vi "VIP_Phase_3.vi"() -> ()   [LabVIEW 2024]
uses:
  <vilib>/DAQmx/read.llb/DAQmx Read (Digital 1D Bool 1Chan 1Samp).vi
  <vilib>/Utility/file.llb/Write To Spreadsheet File (DBL).vi
  <vilib>/DAQmx/create/channels.llb/DAQmx Create Channel (DI-Digital Input).vi
  <vilib>/DAQmx/miscellaneous.llb/DAQmx Fill In Error Info.vi
  <vilib>/ptbypt/NI_PtbyPt.lvlib
panel:
  in  "LED 4":tag="Dev1/port0/line23"
  in  "LED 3":tag="Dev1/port0/line22"
  in  "LED 2":tag="Dev1/port0/line21"
  out "LED 4 (i)":dbl
  out "LED 3 (i)":dbl
  out "LED 2 (i)":dbl
  in  "LED 1":tag="Dev1/port0/line20"
  out "LED 1(i)":dbl
  out "4.2":bool
  out "mouse 4.2":cluster{"Y":dbl[], "Y":dbl[]}[](graph)
  out "mouse 4.1":cluster{"Y":dbl[], "Y":dbl[]}[](graph)
  in  "fake 4.2":bool
  in  "fake 4.1":bool
  out "ratio 4.2R":cluster{"Y":dbl[], "Y":dbl[]}[](graph)=[{"Y"=[2.5380001068115234, 12.063000202178955, 24.592000007629395, 36.145999908447266, 48.69600009918213, 58.23899984359741, 67.79099988937378, 81.40899991989136, 91.96199989318848, 99.9980001449585], "Y"=[0.0, 0.0, 0.0, 0.0, 0.0, 0.0, 0.0, 0.0, 0.0, 0.0]}]
  out "ratio 4.1L":cluster{"Y":dbl[], "Y":dbl[]}[](graph)=[{"Y"=[2.5380001068115234, 12.063000202178955, 24.592000007629395, 36.145999908447266, 48.69600009918213, 58.23899984359741, 67.79099988937378, 81.40899991989136, 91.96199989318848, 99.9980001449585], "Y"=[0.0, 0.0, 0.0, 0.0, 0.0, 0.0, 0.0, 0.0, 0.0, 0.0]}]
  out "ratio 4.2R":dbl
  out "ratio 4.1L":dbl
  in  "water dur (ms) 4.2":dbl=11.5
  in  "water port 4.2":tag="Dev1/port2/line0"
  out "Mouse path 4":path=path "C:/Users/Administrator/Documents/LabVIEW Data/a-lick-20140707-145848"
  out "Mouse file 4":string="a-lick-20140707-145848"
  in  "Mouse ID 4":string
  in  "water dur (ms) 4.1":dbl=9.0
  in  "water port 4.1":tag="Dev1/port1/line7"
  in  "free water 4.2":bool
  in  "free water 4.1":bool
  out "4.1":bool
  out "state 4.2":enum16{"waiting", "sound", "ITI"}(ring)=enum."ITI"
  out "state 4.1":enum16{"waiting", "sound", "ITI"}(ring)=enum."ITI"
  out "water # 4.1L":dbl
  out "water # 4.2R":dbl
  out "lick # 4.2R":dbl
  out "lick # 4.1L":dbl
  out "last water 4.2R":dbl
  out "last water 4.1L":dbl
  out "mistake # 4.2R":dbl
  out "mistake # 4.1L":dbl
  out "ratio 3.2R":cluster{"Y":dbl[], "Y":dbl[]}[](graph)=[{"Y"=[2.5380001068115234, 12.063000202178955, 24.592000007629395, 36.145999908447266, 48.69600009918213, 58.23899984359741, 67.79099988937378, 81.40899991989136, 91.96199989318848, 99.9980001449585], "Y"=[0.0, 0.0, 0.0, 0.0, 0.0, 0.0, 0.0, 0.0, 0.0, 0.0]}]
  out "ratio 3.1L":cluster{"Y":dbl[], "Y":dbl[]}[](graph)=[{"Y"=[2.5380001068115234, 12.063000202178955, 24.592000007629395, 36.145999908447266, 48.69600009918213, 58.23899984359741, 67.79099988937378, 81.40899991989136, 91.96199989318848, 99.9980001449585], "Y"=[0.0, 0.0, 0.0, 0.0, 0.0, 0.0, 0.0, 0.0, 0.0, 0.0]}]
  in  "free water 3.2":bool
  in  "free water 3.1":bool
  in  "water dur (ms) 3. 2":dbl=27.0
  in  "water dur (ms) 3.1":dbl=27.0
  out "mouse 3.2":cluster{"Y":dbl[], "Y":dbl[]}[](graph)
  out "mouse 3.1":cluster{"Y":dbl[], "Y":dbl[]}[](graph)
  in  "fake 3.2":bool
  in  "fake 3.1":bool
  out "last water 3.2R":dbl
  out "last water 3.1L":dbl
  out "mistake # 3.2R":dbl
  out "mistake # 3.1L":dbl
  out "water # 3.2R":dbl
  out "water # 3.1L":dbl
  out "lick # 3.2R":dbl
  out "lick # 3.1L":dbl
  out "ratio 3.2R":dbl
  out "ratio 3.1L":dbl
  in  "water port 3.2":tag="Dev1/port1/line6"
  out "3.2":bool
  out "state 3.2":enum16{"waiting", "sound", "ITI"}(ring)=enum."ITI"
  out "state 3.1":enum16{"waiting", "sound", "ITI"}(ring)=enum."ITI"
  out "3.1":bool
  out "Mouse path 3":path=path "C:/Users/Administrator/Documents/LabVIEW Data/a-lick-20140707-145848"
  out "Mouse file 3":string="a-lick-20140707-145848"
  in  "water port 3.1":tag="Dev1/port1/line5"
  in  "Mouse ID 3":string
  out "ratio 2.2R":cluster{"Y":dbl[], "Y":dbl[]}[](graph)=[{"Y"=[2.5380001068115234, 12.063000202178955, 24.592000007629395, 36.145999908447266, 48.69600009918213, 58.23899984359741, 67.79099988937378, 81.40899991989136, 91.96199989318848, 99.9980001449585], "Y"=[0.0, 0.0, 0.0, 0.0, 0.0, 0.0, 0.0, 0.0, 0.0, 0.0]}]
  out "ratio 2.1L":cluster{"Y":dbl[], "Y":dbl[]}[](graph)=[{"Y"=[2.5380001068115234, 12.063000202178955, 24.592000007629395, 36.145999908447266, 48.69600009918213, 58.23899984359741, 67.79099988937378, 81.40899991989136, 91.96199989318848, 99.9980001449585], "Y"=[0.0, 0.0, 0.0, 0.0, 0.0, 0.0, 0.0, 0.0, 0.0, 0.0]}]
  out "ratio 1.2R":cluster{"Y":dbl[], "Y":dbl[]}[](graph)=[{"Y"=[2.5380001068115234, 12.063000202178955, 24.592000007629395, 36.145999908447266, 48.69600009918213, 58.23899984359741, 67.79099988937378, 81.40899991989136, 91.96199989318848, 99.9980001449585], "Y"=[0.0, 0.0, 0.0, 0.0, 0.0, 0.0, 0.0, 0.0, 0.0, 0.0]}]
  out "mouse 2.2":cluster{"Y":dbl[], "Y":dbl[]}[](graph)
  out "mouse 2.1":cluster{"Y":dbl[], "Y":dbl[]}[](graph)
  in  "free water 2.2":bool
  in  "free water 2.1":bool
  out "last water 2.2R":dbl
  out "last water 2.1L":dbl
  out "mistake # 2.2R":dbl
  out "mistake # 2.1L":dbl
  out "water # 2.2R":dbl
  out "water # 2.1L":dbl
  out "lick  #  2.2R":dbl
  out "lick  #  2.1L":dbl
  out "2.1":bool
  out "ratio 2.2R":dbl
  out "ratio 2.1L":dbl
  out "2.2":bool
  in  "fake 2.2":bool
  in  "fake 2.1":bool
  out "Mouse path 2":path=path "C:/Users/Administrator/Documents/LabVIEW Data/a-lick-20140707-145848"
  out "Mouse file 2":string="a-lick-20140707-145848"
  in  "Mouse ID 2":string
  in  "water dur (ms) 2.2":dbl=27.5
  in  "water dur (ms) 2.1":dbl=36.5
  in  "water port 2.2":tag="Dev1/port1/line4"
  in  "water port 2.1":tag="Dev1/port1/line3"
  out "state 2.2":enum16{"waiting", "sound", "ITI"}(ring)=enum."ITI"
  out "state 2.1":enum16{"waiting", "sound", "ITI"}(ring)=enum."ITI"
  in  "sound port 2":tag="Dev1/ao1"
  out "time (s)":dbl=103.38100004196167
  out "mistake # 1.2R":dbl
  out "mistake # 1.1L":dbl
  in  "water dur (ms) 1.1":dbl=36.0
  in  "water port 1.1":tag="Dev1/port1/line1"
  in  "water dur (ms) 1.2":dbl=28.0
  in  "water port 1.2":tag="Dev1/port1/line2"
  out "1.1":bool
  out "1.2":bool
  out "state 1.2":enum16{"waiting", "sound", "ITI"}(ring)=enum."ITI"
  out "lick # 1.2R":dbl
  out "water # 1.2R":dbl
  in  "fake 1.2":bool
  in  "free water 1.2":bool
  out "mouse 1.2":cluster{"Y":dbl[], "Y":dbl[]}[](graph)
  out "ratio 1.2R":dbl
  out "last water 1.2R":dbl
  out "ratio 1.1L":dbl
  out "ratio 1.1L":cluster{"Y":dbl[], "Y":dbl[]}[](graph)=[{"Y"=[2.5380001068115234, 12.063000202178955, 24.592000007629395, 36.145999908447266, 48.69600009918213, 58.23899984359741, 67.79099988937378, 81.40899991989136, 91.96199989318848, 99.9980001449585], "Y"=[0.0, 0.0, 0.0, 0.0, 0.0, 0.0, 0.0, 0.0, 0.0, 0.0]}]
  in  "free water 1.1":bool
  out "Right Speaker":dbl=5.0
  out "Left Speaker":dbl=5.0
  in  "sound file 2":path=path "C:/Users/cvm-gritton-lab/Documents/Lab View Programs/Lab View Programs/LabVIEW VIs/Tones/New_Phase_2_Sounds/200k_target2.wav"
  in  "ITI max (ms)":dbl=7000.0
  in  "ITI min (ms)":dbl=5000.0
  in  "reaction dur (ms)":dbl=1750.0
  in  "sound dur (ms)":dbl=3000.0
  in  "sound file 1":path=path "C:/Users/cvm-gritton-lab/Documents/Lab View Programs/Lab View Programs/LabVIEW VIs/Tones/New_Phase_2_Sounds/200k_target1.wav"
  in  "sound port 1":tag="Dev1/ao0"
  out "trial state":T1(ring)=enum."ITI"
  out "trial #":dbl=10.0
  out "current sound":dbl=1.0
  out "next sound":dbl[](array[numeric])
  out "Mouse path 1":path=path "C:/Users/Administrator/Documents/LabVIEW Data/a-lick-20140707-145848"
  in  "fake 1.1":bool
  out "mouse 1.1":cluster{"Y":dbl[], "Y":dbl[]}[](graph)
  out "ITI (s)":dbl=6.5
  out "last water 1.1L":dbl
  out "state 1.1":enum16{"waiting", "sound", "ITI"}(ring)=enum."ITI"
  out "water # 1.1L":dbl
  out "lick # 1.1L":dbl
  out "Mouse file 1":string="a-lick-20140707-145848"
  out "data folder":path=path "C:/LabVIEW VIs/LabVIEW data"
  in  "Mouse ID 1":string="VIP_1"
  in  "lick port":tag="Dev1/port0/line0:7"
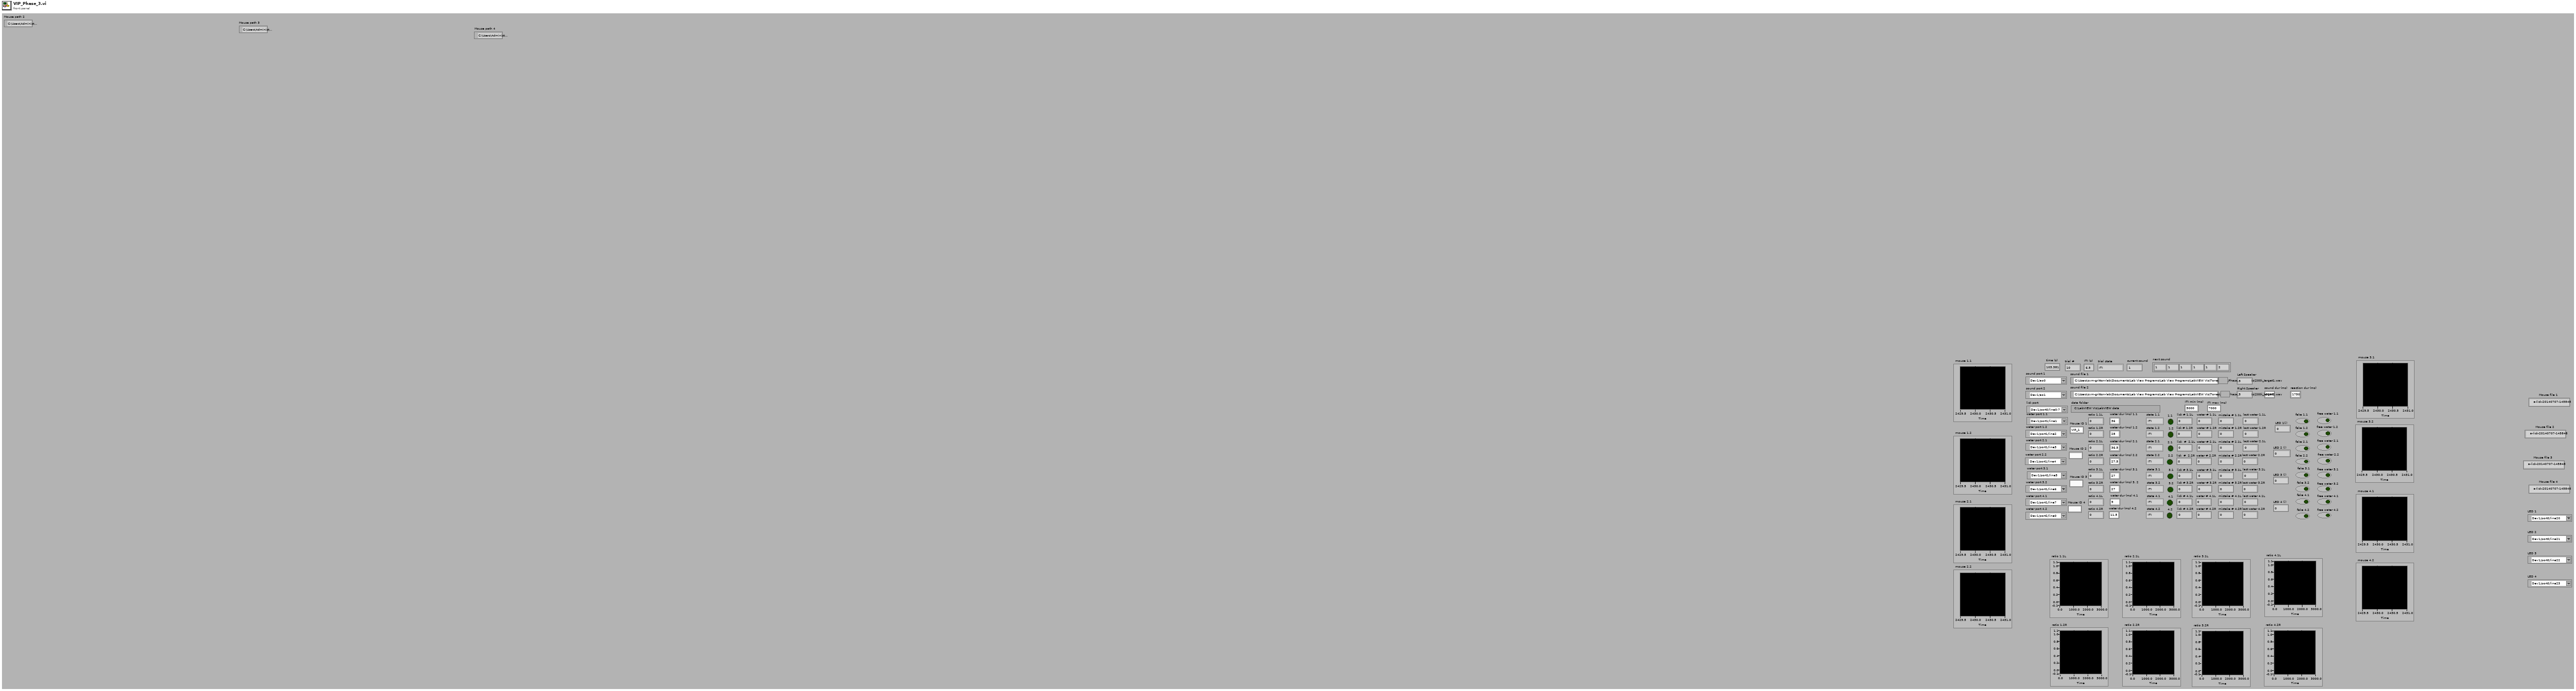
[diagram p1: front panel]
types:
  T1 = enum16{"prepare", "sound", "reaction window", "ITI", "free water", "graph", "data collection"}
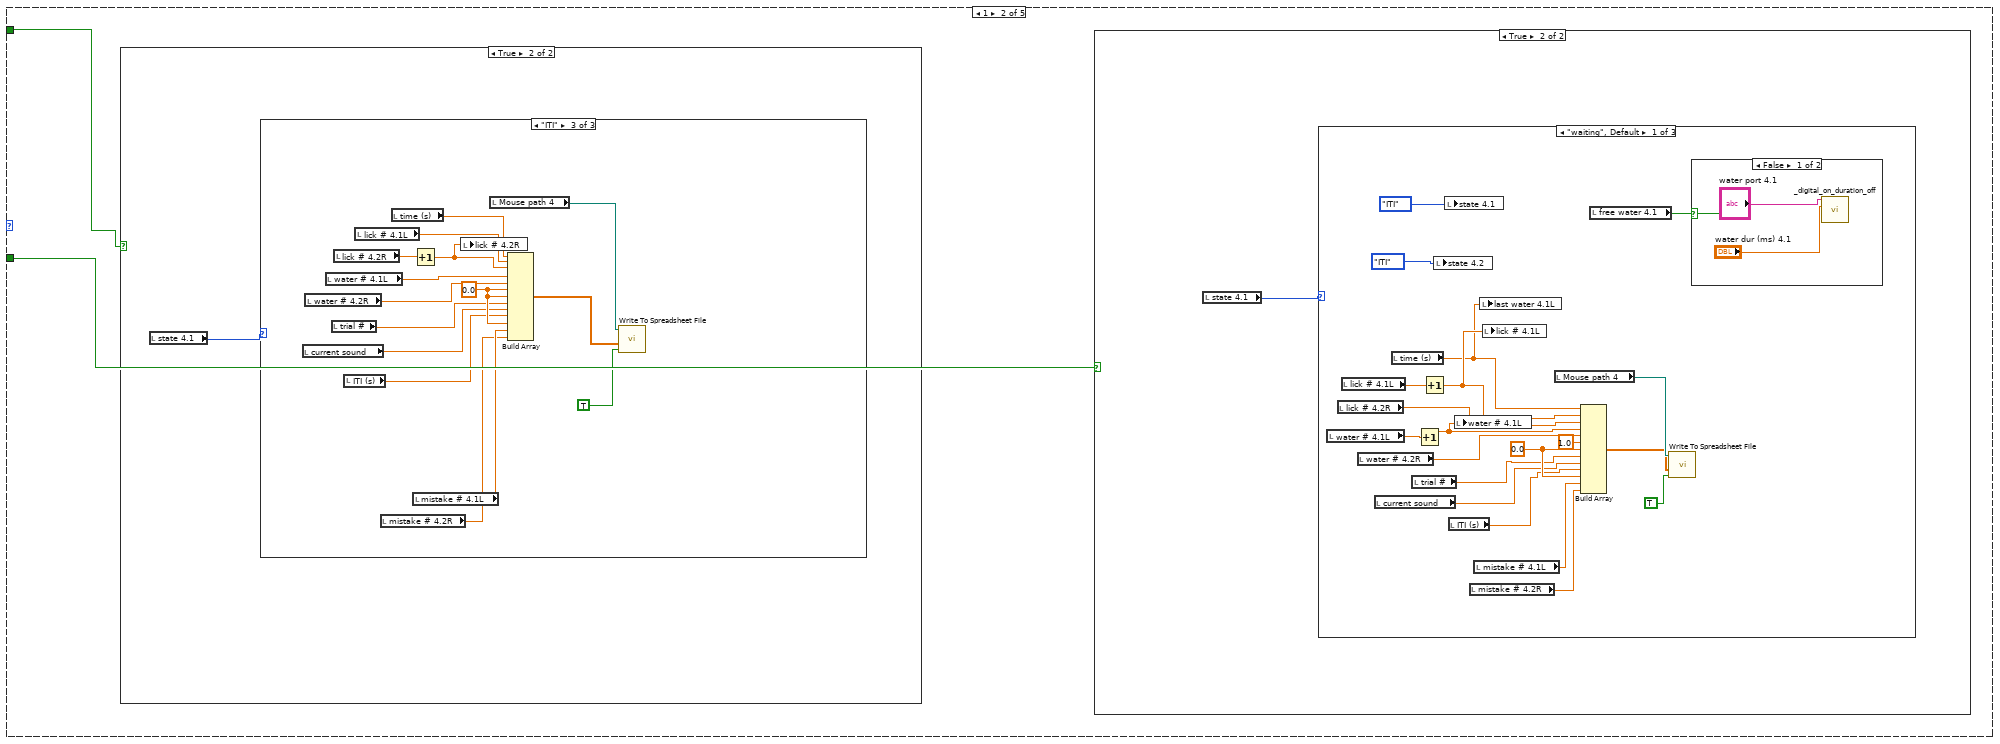
[diagram p3: hidden frame]
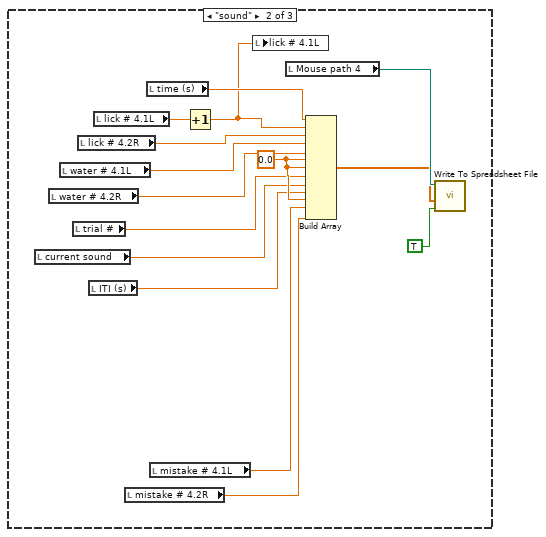
[diagram p6: hidden frame]
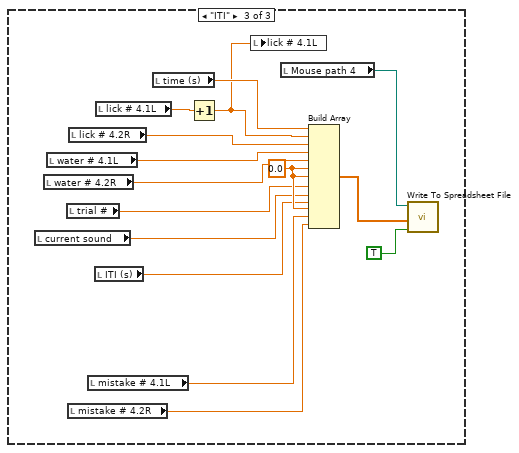
[diagram p7: hidden frame]
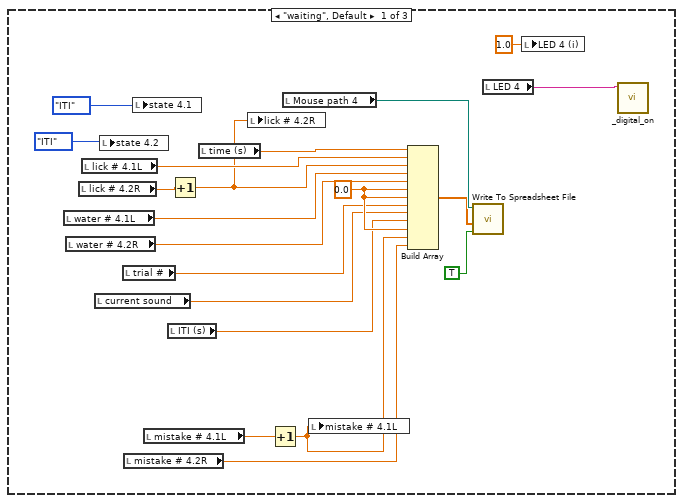
[diagram p9: hidden frame]
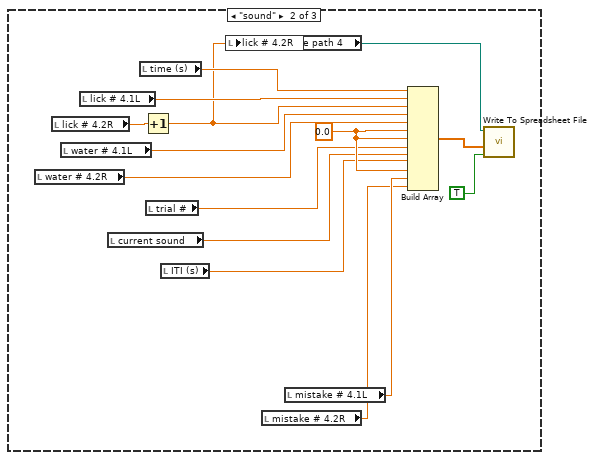
[diagram p10: hidden frame]
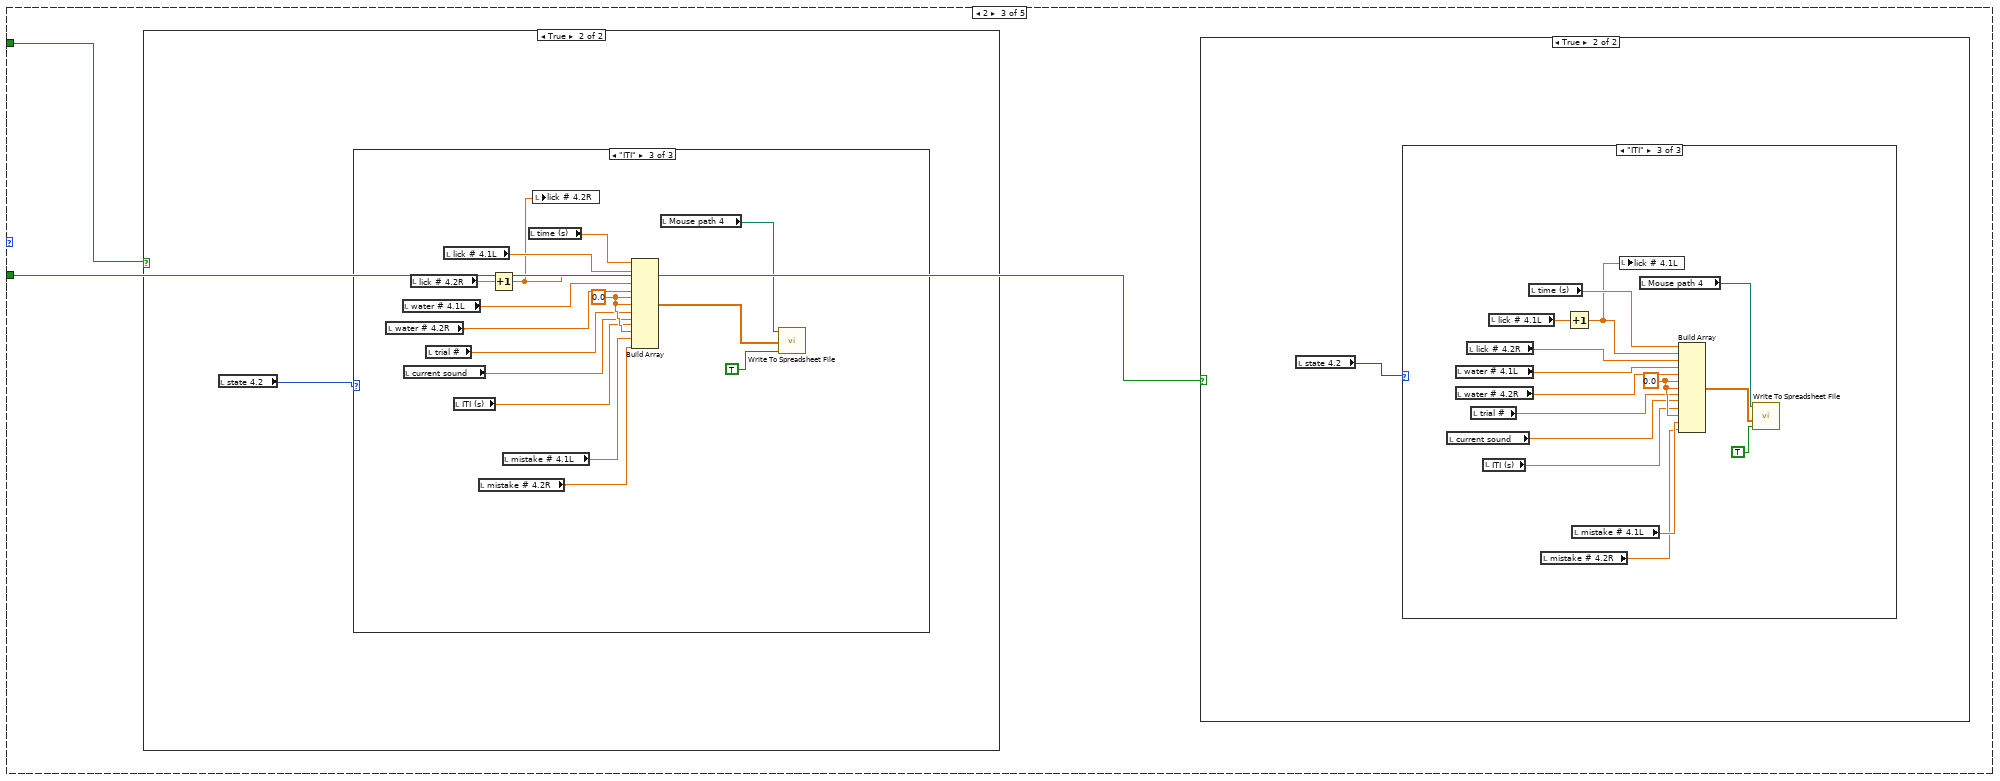
[diagram p11: hidden frame]
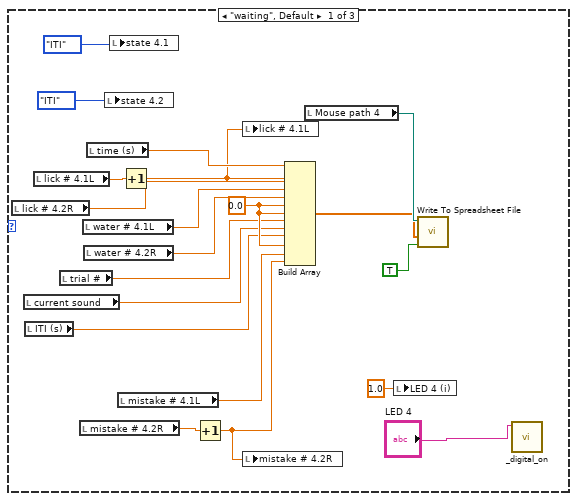
[diagram p13: hidden frame]
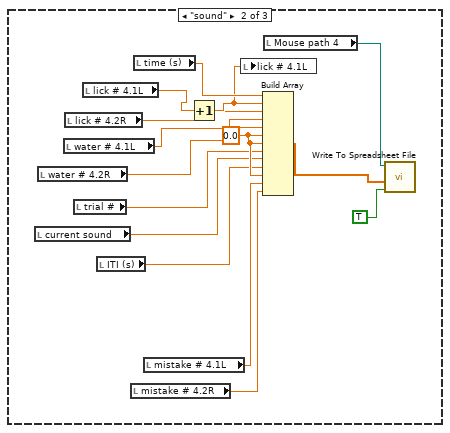
[diagram p14: hidden frame]
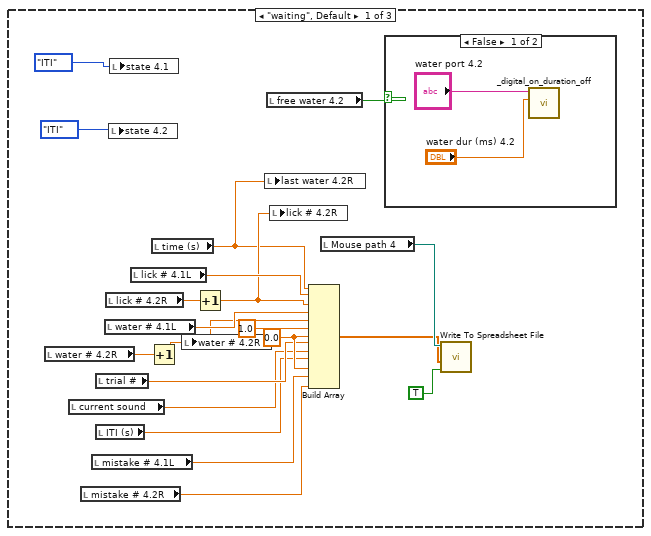
[diagram p16: hidden frame]
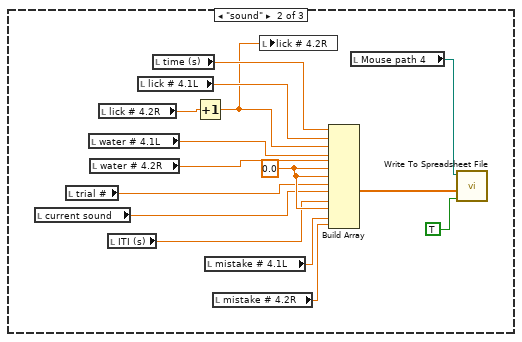
[diagram p18: hidden frame]
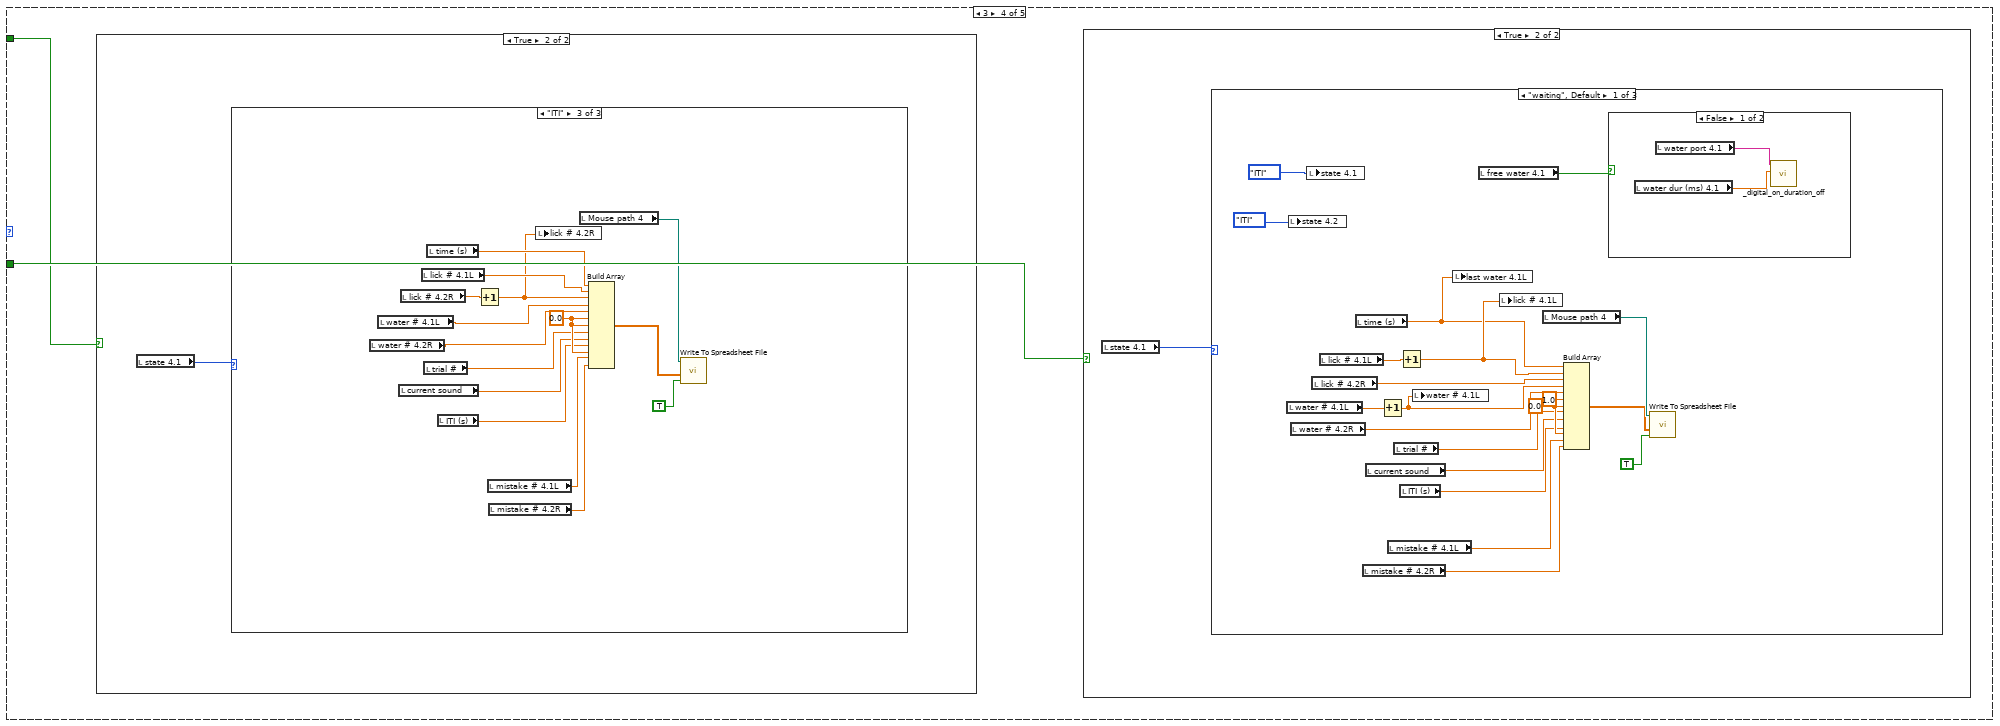
[diagram p19: hidden frame]
diagram:
  n1 = flat-sequence {
    frame #0 {
      w1 = 0.0 ("LED 1 (R)")
      w11 = 0.0 ("mistake # 1.1L")
      w3 = 0
      w21 = 0
      w10 = 0
      w2 = 0
      w9 = enum16{"waiting", "sound", "ITI"}."sound"
      n2 = Get Date/Time In Seconds() -> (seconds since 1Jan1904=w23:timestamp)
      n3 = call <vilib>:"Dflt Data Dir.vi"() -> ("App:Default Data Directory"=w5:path)
      "data folder" <- w5
      n4 = Format Date/Time String(time format string (%c)="%m%d%Y-%H%M%S-", seconds (now)=w23) -> (date/time string=w8:string)  [unwired: 1 in]
      n5 = Concatenate Strings(w8, "Mouse ID 1") -> (w26:string)
      "Mouse file 1" <- w26
      n6 = Concatenate Strings(w8, "Mouse ID 4") -> (w6:string)
      "Mouse file 4" <- w6
      n7 = Concatenate Strings(w8, "Mouse ID 2") -> (w16:string)
      "Mouse file 2" <- w16
      n8 = Concatenate Strings(w8, "Mouse ID 3") -> (w13:string)
      "Mouse file 3" <- w13
      n9 = Build Path(base path=w5, name or relative path=w26) -> (appended path=→"Mouse path 1":path)
      n10 = Build Path(base path=w5, name or relative path=w16) -> (appended path=→"Mouse path 2":path)
      n11 = Build Path(base path=w5, name or relative path=w13) -> (appended path=→"Mouse path 3":path)
      n12 = Build Path(base path=w5, name or relative path=w6) -> (appended path=→"Mouse path 4":path)
      n13 = call "_array_shuffle.vi"("total number"=70, "input array"=i32[] [1, 2, 3, 4, 1, 2, 3, 4]) -> ("output array"=→"next sound":dbl[])  [unwired: 9 in]
      n14 = local write "time (s)"(w21) -> ()
      "water # 1.1L" <- w2
      "lick # 1.1L" <- w2
      "state 1.1" <- w9
      "last water 1.1L" <- w10
      "current sound" <- w21
      "trial #" <- w21
      "ITI (s)" <- w21
      "Left Speaker" <- w21
      "Right Speaker" <- w21
      "ratio 1.1L" <- w3
      "last water 1.2R" <- w10
      "ratio 1.2R" <- w3
      "water # 1.2R" <- w2
      "lick # 1.2R" <- w2
      "state 1.2" <- w9
      "mistake # 1.1L" <- w11
      "mistake # 1.2R" <- w11
      "state 2.1" <- w9
      "state 2.2" <- w9
      "ratio 2.1L" <- w3
      "ratio 2.2R" <- w3
      "lick  #  2.1L" <- w2
      "lick  #  2.2R" <- w2
      "water # 2.1L" <- w2
      "water # 2.2R" <- w2
      "mistake # 2.1L" <- w11
      "mistake # 2.2R" <- w11
      "last water 2.1L" <- w10
      "last water 2.2R" <- w10
      "state 3.1" <- w9
      "state 3.2" <- w9
      "ratio 3.1L" <- w3
      "ratio 3.2R" <- w3
      "lick # 3.1L" <- w2
      "lick # 3.2R" <- w2
      "water # 3.1L" <- w2
      "water # 3.2R" <- w2
      "mistake # 3.1L" <- w11
      "mistake # 3.2R" <- w11
      "last water 3.1L" <- w10
      "last water 3.2R" <- w10
      "mistake # 4.1L" <- w11
      "mistake # 4.2R" <- w11
      "last water 4.1L" <- w10
      "last water 4.2R" <- w10
      "lick # 4.1L" <- w2
      "lick # 4.2R" <- w2
      "water # 4.2R" <- w2
      "water # 4.1L" <- w2
      "state 4.1" <- w9
      "state 4.2" <- w9
      "ratio 4.1L" <- w3
      "ratio 4.2R" <- w3
      "LED 1(i)" <- w1
      "LED 2 (i)" <- w1
      "LED 3 (i)" <- w1
      "LED 4 (i)" <- w1
    }
    frame #1 {
      # "file format:\n1. time stamp\n2. lick #\n3. water #\n4. water triggered by lick?\n5. trial start?\n6. trial #\n7. trial sound\n8. trial ITI\n9. free water?"
      n15 = call-poly <vilib>:"DAQmx Create Virtual Channel.vi"("lines"="lick port") -> ("task out"=w28:refnum<k21>)  [unwired: 13 in, 1 out]
      n16 = call <vilib>:"DAQmx Start Task.vi"("task/channels in"=w28) -> ("task out"=w29:refnum<k21>)  [unwired: 13 in, 1 out]
      n17 = while {
        tunnel: w29 -> [w88]
        tunnel: [w87] -> w30
        shift-right: [w78] -> _
        shift-left: _ -> [w86]
        shift-right: [w83] -> _
        shift-left: _ -> [w84]
        stop <- FALSE stop-if-true
        n18 = call-poly <vilib>:"DAQmx Read.vi"("task/channels in"=w88) -> ("task out"=w87:refnum<k21>, "data"=w79:bool[])  [unwired: 12 in, 1 out]
        n19 = Build Array("fake 1.1", "fake 1.2", "fake 2.1", "fake 2.2", "fake 3.1", "fake 3.2", "fake 4.1", "fake 4.2") -> (w75:bool[])
        n20 = Or(x=w79, y=w75) -> (x .or. y?=w78:bool[])
        n21 = Index Array(array=w78) -> (element #1=w81:bool, element #2=w67:bool, element #3=w58:bool, element #4=w55:bool, element #5=w47:bool, element #6=w44:bool, element #7=w39:bool, element #8=w35:bool)  [unwired: 8 in]
        n22 = call "Collector1."("Signals"=w58) -> ("Collected Signals"=w59:dynamicdata)  [unwired: 9 in, 1 out]
        n23 = call "Collector1.2"("Signals"=w67) -> ("Collected Signals"=w66:dynamicdata)  [unwired: 9 in, 1 out]
        n24 = call "Collector1.7"("Signals"=w35) -> ("Collected Signals"=w37:dynamicdata)  [unwired: 9 in, 1 out]
        n25 = call "Collector1.3"("Signals"=w55) -> ("Collected Signals"=w56:dynamicdata)  [unwired: 9 in, 1 out]
        n26 = call "Collector1.6"("Signals"=w39) -> ("Collected Signals"=w40:dynamicdata)  [unwired: 9 in, 1 out]
        n27 = call "Collector1.1"("Signals"=w81) -> ("Collected Signals"=w68:dynamicdata)  [unwired: 9 in, 1 out]
        n28 = call "Collector1.5"("Signals"=w44) -> ("Collected Signals"=w45:dynamicdata)  [unwired: 9 in, 1 out]
        n29 = call "Collector1.4"("Signals"=w47) -> ("Collected Signals"=w48:dynamicdata)  [unwired: 9 in, 1 out]
        n30 = local read "time (s)"() -> (w82:dbl)
        n31 = call "Collector"("Signals"=w82) -> ("Collected Signals"=w34:dynamicdata)  [unwired: 9 in, 1 out]
        n32 = call "Build XY Graph1.1"("Y Input"=w68, "X Input"=w34) -> ("XY Graph"=→"mouse 1.1":cluster{"Y":dbl[], "Y":dbl[]}[])  [unwired: 3 in, 6 out]
        n33 = call "Build XY Graph1."("Y Input"=w59, "X Input"=w34) -> ("XY Graph"=→"mouse 2.1":cluster{"Y":dbl[], "Y":dbl[]}[])  [unwired: 3 in, 6 out]
        n34 = call "Build XY Graph1.2"("Y Input"=w66, "X Input"=w34) -> ("XY Graph"=→"mouse 1.2":cluster{"Y":dbl[], "Y":dbl[]}[])  [unwired: 3 in, 6 out]
        n35 = call "Build XY Graph1.7"("Y Input"=w37, "X Input"=w34) -> ("XY Graph"=→"mouse 4.2":cluster{"Y":dbl[], "Y":dbl[]}[])  [unwired: 3 in, 6 out]
        n36 = call "Build XY Graph1.3"("Y Input"=w56, "X Input"=w34) -> ("XY Graph"=→"mouse 2.2":cluster{"Y":dbl[], "Y":dbl[]}[])  [unwired: 3 in, 6 out]
        n37 = call "Build XY Graph1.6"("Y Input"=w40, "X Input"=w34) -> ("XY Graph"=→"mouse 4.1":cluster{"Y":dbl[], "Y":dbl[]}[])  [unwired: 3 in, 6 out]
        n38 = call "Build XY Graph1.5"("Y Input"=w45, "X Input"=w34) -> ("XY Graph"=→"mouse 3.2":cluster{"Y":dbl[], "Y":dbl[]}[])  [unwired: 3 in, 6 out]
        n39 = call "Build XY Graph1.4"("Y Input"=w48, "X Input"=w34) -> ("XY Graph"=→"mouse 3.1":cluster{"Y":dbl[], "Y":dbl[]}[])  [unwired: 3 in, 6 out]
        n40 = Greater?(x=w78, y=w86) -> (0:w85:bool[])
        n41 = Index Array(array=w85) -> (element #1=w73:bool, element #2=w72:bool, element #3=w61:bool, element #4=w62:bool, element #5=w53:bool, element #6=w52:bool, element #7=w32:bool, element #8=w33:bool)  [unwired: 8 in]
        "1.2" <- w72
        "1.1" <- w73
        "2.2" <- w62
        "2.1" <- w61
        "3.1" <- w53
        "3.2" <- w52
        "4.1" <- w32
        "4.2" <- w33
        n42 = local read "current sound"() -> (w71:dbl)
        n43 = local read "current sound"() -> (w65:dbl)
        n44 = local read "current sound"() -> (w43:dbl)
        n45 = local read "current sound"() -> (w54:dbl)
        n46 = case shown="4" w54 {
          tunnel: w53 -> [_ w514 w620 w726 w832]
          tunnel: w52 -> [_ w513 w619 w725 w831]
          frame 0, Default {
          }
          frame 1 {
            n47 = case shown="True" w514 {
              frame False {
              }
              frame True {
                n48 = local read "state 3.1"() -> (w566:enum16{"waiting", "sound", "ITI"})
                n49 = case shown="\"waiting\", Default" w566 {
                  frame "waiting", Default {
                    w575 = 0.0 ("element")
                    n50 = local write "state 3.2"(enum16{"waiting", "sound", "ITI"}."ITI") -> ()
                    n51 = local read "free water 3.1"() -> (w586:bool)
                    n52 = local write "state 3.1"(enum16{"waiting", "sound", "ITI"}."ITI") -> ()
                    n53 = local read "water # 3.1L"() -> (w578:dbl)
                    n54 = local read "lick # 3.2R"() -> (w579:dbl)
                    n55 = local read "lick # 3.1L"() -> (w581:dbl)
                    n56 = local read "water # 3.2R"() -> (w576:dbl)
                    n57 = local read "current sound"() -> (w568:dbl)
                    n58 = case shown="False" w586 {
                      frame False {
                        n59 = call "_digital_on_duration_off.vi"("duration (ms)"="water dur (ms) 3.1", "digital port"="water port 3.1") -> ()  [unwired: 10 in]
                      }
                      frame True {
                      }
                    }
                    n60 = local read "mistake # 3.2R"() -> (w573:dbl)
                    n61 = local read "mistake # 3.1L"() -> (w574:dbl)
                    n62 = local read "ITI (s)"() -> (w567:dbl)
                    n63 = local read "trial #"() -> (w569:dbl)
                    n64 = Increment(x=w578) -> (x+1=w577:dbl)
                    n65 = Increment(x=w581) -> (x+1=w580:dbl)
                    n66 = local read "time (s)"() -> (w582:dbl)
                    n67 = local write "water # 3.1L"(w577) -> ()
                    n68 = local write "lick # 3.1L"(w580) -> ()
                    n69 = local write "last water 3.1L"(w582) -> ()
                    n70 = local read "Mouse path 3"() -> (w585:path)
                    n71 = Build Array(w582, w580, w579, w577, w576, 1.0 ("element"), w575, w569, w568, w567, w575, w574, w573) -> (w583:dbl[])
                    n72 = call-poly <vilib>:"Write To Spreadsheet File.vi"("append to file? (new file:F)"=TRUE, "1D data"=w583, "file path (dialog if empty)"=w585) -> ()  [unwired: 5 in, 1 out]
                  }
                  frame "sound" {
                    w594 = 0.0 ("element")
                    n73 = local read "current sound"() -> (w590:dbl)
                    n74 = local read "trial #"() -> (w591:dbl)
                    n75 = local read "water # 3.2R"() -> (w595:dbl)
                    n76 = local read "water # 3.1L"() -> (w596:dbl)
                    n77 = local read "mistake # 3.2R"() -> (w592:dbl)
                    n78 = local read "lick # 3.2R"() -> (w597:dbl)
                    n79 = local read "lick # 3.1L"() -> (w599:dbl)
                    n80 = local read "ITI (s)"() -> (w589:dbl)
                    n81 = local read "mistake # 3.1L"() -> (w593:dbl)
                    n82 = local read "time (s)"() -> (w600:dbl)
                    n83 = Increment(x=w599) -> (x+1=w598:dbl)
                    n84 = local write "lick # 3.1L"(w598) -> ()
                    n85 = local read "Mouse path 3"() -> (w603:path)
                    n86 = Build Array(w600, w598, w597, w596, w595, w594, w594, w591, w590, w589, w594, w593, w592) -> (w601:dbl[])
                    n87 = call-poly <vilib>:"Write To Spreadsheet File.vi"("append to file? (new file:F)"=TRUE, "1D data"=w601, "file path (dialog if empty)"=w603) -> ()  [unwired: 5 in, 1 out]
                  }
                  frame "ITI" {
                    w609 = 0.0 ("element")
                    n88 = local read "water # 3.2R"() -> (w610:dbl)
                    n89 = local read "current sound"() -> (w605:dbl)
                    n90 = local read "lick # 3.2R"() -> (w612:dbl)
                    n91 = local read "lick # 3.1L"() -> (w614:dbl)
                    n92 = local read "water # 3.1L"() -> (w611:dbl)
                    n93 = local read "trial #"() -> (w606:dbl)
                    n94 = local read "ITI (s)"() -> (w604:dbl)
                    n95 = local read "time (s)"() -> (w615:dbl)
                    n96 = Increment(x=w614) -> (x+1=w613:dbl)
                    n97 = local read "mistake # 3.1L"() -> (w608:dbl)
                    n98 = local read "mistake # 3.2R"() -> (w607:dbl)
                    n99 = local write "lick # 3.1L"(w613) -> ()
                    n100 = local read "Mouse path 3"() -> (w618:path)
                    n101 = Build Array(w615, w613, w612, w611, w610, w609, w609, w606, w605, w604, w609, w608, w607) -> (w616:dbl[])
                    n102 = call-poly <vilib>:"Write To Spreadsheet File.vi"("append to file? (new file:F)"=TRUE, "1D data"=w616, "file path (dialog if empty)"=w618) -> ()  [unwired: 5 in, 1 out]
                  }
                }
              }
            }
            n103 = case shown="True" w513 {
              frame False {
              }
              frame True {
                n104 = local read "state 3.1"() -> (w515:enum16{"waiting", "sound", "ITI"})
                n105 = case shown="\"ITI\"" w515 {
                  frame "waiting", Default {
                    w524 = 0.0 ("element")
                    n106 = local read "mistake # 3.1L"() -> (w523:dbl)
                    n107 = local write "state 3.2"(enum16{"waiting", "sound", "ITI"}."ITI") -> ()
                    n108 = local write "state 3.1"(enum16{"waiting", "sound", "ITI"}."ITI") -> ()
                    n109 = Increment(x=w523) -> (x+1=w522:dbl)
                    n110 = local read "water # 3.2R"() -> (w525:dbl)
                    n111 = local read "water # 3.1L"() -> (w526:dbl)
                    n112 = local read "lick # 3.2R"() -> (w528:dbl)
                    n113 = local read "current sound"() -> (w517:dbl)
                    n114 = local read "mistake # 3.2R"() -> (w521:dbl)
                    n115 = local write "mistake # 3.1L"(w522) -> ()
                    n116 = local read "lick # 3.1L"() -> (w529:dbl)
                    n117 = local read "ITI (s)"() -> (w516:dbl)
                    n118 = local read "trial #"() -> (w518:dbl)
                    n119 = local read "time (s)"() -> (w530:dbl)
                    n120 = Increment(x=w528) -> (x+1=w527:dbl)
                    n121 = local write "lick # 3.2R"(w527) -> ()
                    n122 = Build Array(w530, w529, w527, w526, w525, w524, w524, w518, w517, w516, w524, w522, w521) -> (w531:dbl[])
                    n123 = local read "Mouse path 3"() -> (w533:path)
                    n124 = call "_digital_on.vi"("digital port"="LED 3") -> ()  [unwired: 11 in]
                    n125 = call-poly <vilib>:"Write To Spreadsheet File.vi"("append to file? (new file:F)"=TRUE, "1D data"=w531, "file path (dialog if empty)"=w533) -> ()  [unwired: 5 in, 1 out]
                    n126 = local write "LED 3 (i)"(1.0 ("LED 3 (i)")) -> ()
                  }
                  frame "sound" {
                    w541 = 0.0 ("element")
                    n127 = local read "water # 3.1L"() -> (w543:dbl)
                    n128 = local read "lick # 3.2R"() -> (w545:dbl)
                    n129 = local read "water # 3.2R"() -> (w542:dbl)
                    n130 = local read "lick # 3.1L"() -> (w546:dbl)
                    n131 = local read "current sound"() -> (w537:dbl)
                    n132 = local read "trial #"() -> (w538:dbl)
                    n133 = local read "time (s)"() -> (w547:dbl)
                    n134 = Increment(x=w545) -> (x+1=w544:dbl)
                    n135 = local read "ITI (s)"() -> (w536:dbl)
                    n136 = local read "mistake # 3.2R"() -> (w539:dbl)
                    n137 = local read "mistake # 3.1L"() -> (w540:dbl)
                    n138 = local write "lick # 3.2R"(w544) -> ()
                    n139 = local read "Mouse path 3"() -> (w549:path)
                    n140 = Build Array(w547, w546, w544, w543, w542, w541, w541, w538, w537, w536, w541, w540, w539) -> (w548:dbl[])
                    n141 = call-poly <vilib>:"Write To Spreadsheet File.vi"("append to file? (new file:F)"=TRUE, "1D data"=w548, "file path (dialog if empty)"=w549) -> ()  [unwired: 5 in, 1 out]
                  }
                  frame "ITI" {
                    w556 = 0.0 ("element")
                    n142 = local read "water # 3.2R"() -> (w557:dbl)
                    n143 = local read "water # 3.1L"() -> (w558:dbl)
                    n144 = local read "lick # 3.2R"() -> (w560:dbl)
                    n145 = local read "current sound"() -> (w552:dbl)
                    n146 = local read "lick # 3.1L"() -> (w561:dbl)
                    n147 = local read "trial #"() -> (w553:dbl)
                    n148 = Increment(x=w560) -> (x+1=w559:dbl)
                    n149 = local read "time (s)"() -> (w562:dbl)
                    n150 = local read "mistake # 3.2R"() -> (w554:dbl)
                    n151 = local read "ITI (s)"() -> (w551:dbl)
                    n152 = local read "mistake # 3.1L"() -> (w555:dbl)
                    n153 = local write "lick # 3.2R"(w559) -> ()
                    n154 = local read "Mouse path 3"() -> (w564:path)
                    n155 = Build Array(w562, w561, w559, w558, w557, w556, w556, w553, w552, w551, w556, w555, w554) -> (w563:dbl[])
                    n156 = call-poly <vilib>:"Write To Spreadsheet File.vi"("append to file? (new file:F)"=TRUE, "1D data"=w563, "file path (dialog if empty)"=w564) -> ()  [unwired: 5 in, 1 out]
                  }
                }
              }
            }
          }
          frame 2 {
            n157 = case shown="True" w620 {
              frame False {
              }
              frame True {
                n158 = local read "state 3.2"() -> (w674:enum16{"waiting", "sound", "ITI"})
                n159 = case shown="\"waiting\", Default" w674 {
                  frame "waiting", Default {
                    w683 = 0.0 ("element")
                    n160 = local read "water # 3.2R"() -> (w684:dbl)
                    n161 = local read "water # 3.1L"() -> (w685:dbl)
                    n162 = local read "lick # 3.2R"() -> (w686:dbl)
                    n163 = local read "lick # 3.1L"() -> (w688:dbl)
                    n164 = local read "current sound"() -> (w676:dbl)
                    n165 = local write "state 3.2"(enum16{"waiting", "sound", "ITI"}."ITI") -> ()
                    n166 = local read "trial #"() -> (w677:dbl)
                    n167 = local read "ITI (s)"() -> (w675:dbl)
                    n168 = local read "mistake # 3.1L"() -> (w682:dbl)
                    n169 = local read "time (s)"() -> (w689:dbl)
                    n170 = local read "mistake # 3.2R"() -> (w681:dbl)
                    n171 = local write "state 3.1"(enum16{"waiting", "sound", "ITI"}."ITI") -> ()
                    n172 = Increment(x=w688) -> (x+1=w687:dbl)
                    n173 = local write "lick # 3.1L"(w687) -> ()
                    n174 = local read "Mouse path 3"() -> (w691:path)
                    n175 = Increment(x=w681) -> (x+1=w680:dbl)
                    n176 = local write "mistake # 3.2R"(w680) -> ()
                    n177 = Build Array(w689, w687, w686, w685, w684, w683, w683, w677, w676, w675, w683, w682, w680) -> (w690:dbl[])
                    n178 = local read "LED 3"() -> (w679:tag)
                    n179 = call-poly <vilib>:"Write To Spreadsheet File.vi"("append to file? (new file:F)"=TRUE, "1D data"=w690, "file path (dialog if empty)"=w691) -> ()  [unwired: 5 in, 1 out]
                    n180 = local write "LED 3 (i)"(1.0 ("LED 3 (i)")) -> ()
                    n181 = call "_digital_on.vi"("digital port"=w679) -> ()  [unwired: 11 in]
                  }
                  frame "sound" {
                    w700 = 0.0 ("element")
                    n182 = local read "current sound"() -> (w696:dbl)
                    n183 = local read "water # 3.2R"() -> (w701:dbl)
                    n184 = local read "water # 3.1L"() -> (w702:dbl)
                    n185 = local read "trial #"() -> (w697:dbl)
                    n186 = local read "lick # 3.2R"() -> (w703:dbl)
                    n187 = local read "lick # 3.1L"() -> (w705:dbl)
                    n188 = local read "ITI (s)"() -> (w695:dbl)
                    n189 = local read "mistake # 3.2R"() -> (w698:dbl)
                    n190 = local read "time (s)"() -> (w706:dbl)
                    n191 = local read "mistake # 3.1L"() -> (w699:dbl)
                    n192 = Increment(x=w705) -> (x+1=w704:dbl)
                    n193 = local write "lick # 3.1L"(w704) -> ()
                    n194 = local read "Mouse path 3"() -> (w708:path)
                    n195 = Build Array(w706, w704, w703, w702, w701, w700, w700, w697, w696, w695, w700, w699, w698) -> (w707:dbl[])
                    n196 = call-poly <vilib>:"Write To Spreadsheet File.vi"("append to file? (new file:F)"=TRUE, "1D data"=w707, "file path (dialog if empty)"=w708) -> ()  [unwired: 5 in, 1 out]
                  }
                  frame "ITI" {
                    w715 = 0.0 ("element")
                    n197 = local read "current sound"() -> (w711:dbl)
                    n198 = local read "water # 3.2R"() -> (w716:dbl)
                    n199 = local read "water # 3.1L"() -> (w717:dbl)
                    n200 = local read "lick # 3.2R"() -> (w718:dbl)
                    n201 = local read "trial #"() -> (w712:dbl)
                    n202 = local read "lick # 3.1L"() -> (w720:dbl)
                    n203 = local read "ITI (s)"() -> (w710:dbl)
                    n204 = local read "mistake # 3.2R"() -> (w713:dbl)
                    n205 = local read "time (s)"() -> (w721:dbl)
                    n206 = local read "mistake # 3.1L"() -> (w714:dbl)
                    n207 = Increment(x=w720) -> (x+1=w719:dbl)
                    n208 = local write "lick # 3.1L"(w719) -> ()
                    n209 = local read "Mouse path 3"() -> (w723:path)
                    n210 = Build Array(w721, w719, w718, w717, w716, w715, w715, w712, w711, w710, w715, w714, w713) -> (w722:dbl[])
                    n211 = call-poly <vilib>:"Write To Spreadsheet File.vi"("append to file? (new file:F)"=TRUE, "1D data"=w722, "file path (dialog if empty)"=w723) -> ()  [unwired: 5 in, 1 out]
                  }
                }
              }
            }
            n212 = case shown="True" w619 {
              frame False {
              }
              frame True {
                n213 = local read "state 3.2"() -> (w621:enum16{"waiting", "sound", "ITI"})
                n214 = case shown="\"ITI\"" w621 {
                  frame "waiting", Default {
                    w629 = 0.0 ("element")
                    n215 = local read "water # 3.2R"() -> (w631:dbl)
                    n216 = local read "current sound"() -> (w623:dbl)
                    n217 = local read "lick # 3.2R"() -> (w634:dbl)
                    n218 = local read "water # 3.1L"() -> (w632:dbl)
                    n219 = local read "trial #"() -> (w624:dbl)
                    n220 = local read "mistake # 3.2R"() -> (w627:dbl)
                    n221 = local write "state 3.1"(enum16{"waiting", "sound", "ITI"}."ITI") -> ()
                    n222 = local write "state 3.2"(enum16{"waiting", "sound", "ITI"}."ITI") -> ()
                    n223 = local read "ITI (s)"() -> (w622:dbl)
                    n224 = local read "lick # 3.1L"() -> (w635:dbl)
                    n225 = local read "mistake # 3.1L"() -> (w628:dbl)
                    n226 = local read "time (s)"() -> (w626:dbl)
                    n227 = Increment(x=w631) -> (x+1=w630:dbl)
                    n228 = Increment(x=w634) -> (x+1=w633:dbl)
                    n229 = local read "free water 3.2"() -> (w641:bool)
                    n230 = local write "water # 3.2R"(w630) -> ()
                    n231 = local write "last water 3.2R"(w626) -> ()
                    n232 = local write "lick # 3.2R"(w633) -> ()
                    n233 = local read "Mouse path 3"() -> (w637:path)
                    n234 = Build Array(w626, w635, w633, w632, w630, 1.0 ("element"), w629, w624, w623, w622, w629, w628, w627) -> (w636:dbl[])
                    n235 = case shown="False" w641 {
                      frame False {
                        n236 = call "_digital_on_duration_off.vi"("duration (ms)"="water dur (ms) 3. 2", "digital port"="water port 3.2") -> ()  [unwired: 10 in]
                      }
                      frame True {
                      }
                    }
                    n237 = call-poly <vilib>:"Write To Spreadsheet File.vi"("append to file? (new file:F)"=TRUE, "1D data"=w636, "file path (dialog if empty)"=w637) -> ()  [unwired: 5 in, 1 out]
                  }
                  frame "sound" {
                    w649 = 0.0 ("element")
                    n238 = local read "lick # 3.2R"() -> (w653:dbl)
                    n239 = local read "water # 3.1L"() -> (w651:dbl)
                    n240 = local read "current sound"() -> (w645:dbl)
                    n241 = local read "trial #"() -> (w646:dbl)
                    n242 = local read "water # 3.2R"() -> (w650:dbl)
                    n243 = local read "lick # 3.1L"() -> (w654:dbl)
                    n244 = local read "ITI (s)"() -> (w644:dbl)
                    n245 = local read "mistake # 3.2R"() -> (w647:dbl)
                    n246 = Increment(x=w653) -> (x+1=w652:dbl)
                    n247 = local read "mistake # 3.1L"() -> (w648:dbl)
                    n248 = local read "time (s)"() -> (w655:dbl)
                    n249 = local write "lick # 3.2R"(w652) -> ()
                    n250 = local read "Mouse path 3"() -> (w658:path)
                    n251 = Build Array(w655, w654, w652, w651, w650, w649, w649, w646, w645, w644, w649, w648, w647) -> (w656:dbl[])
                    n252 = call-poly <vilib>:"Write To Spreadsheet File.vi"("append to file? (new file:F)"=TRUE, "1D data"=w656, "file path (dialog if empty)"=w658) -> ()  [unwired: 5 in, 1 out]
                  }
                  frame "ITI" {
                    w664 = 0.0 ("element")
                    n253 = local read "water # 3.2R"() -> (w665:dbl)
                    n254 = local read "lick # 3.2R"() -> (w668:dbl)
                    n255 = local read "current sound"() -> (w660:dbl)
                    n256 = local read "water # 3.1L"() -> (w666:dbl)
                    n257 = local read "lick # 3.1L"() -> (w669:dbl)
                    n258 = local read "trial #"() -> (w661:dbl)
                    n259 = local read "ITI (s)"() -> (w659:dbl)
                    n260 = local read "time (s)"() -> (w670:dbl)
                    n261 = Increment(x=w668) -> (x+1=w667:dbl)
                    n262 = local read "mistake # 3.2R"() -> (w662:dbl)
                    n263 = local read "mistake # 3.1L"() -> (w663:dbl)
                    n264 = local write "lick # 3.2R"(w667) -> ()
                    n265 = local read "Mouse path 3"() -> (w672:path)
                    n266 = Build Array(w670, w669, w667, w666, w665, w664, w664, w661, w660, w659, w664, w663, w662) -> (w671:dbl[])
                    n267 = call-poly <vilib>:"Write To Spreadsheet File.vi"("append to file? (new file:F)"=TRUE, "1D data"=w671, "file path (dialog if empty)"=w672) -> ()  [unwired: 5 in, 1 out]
                  }
                }
              }
            }
          }
          frame 3 {
            n268 = case shown="True" w726 {
              frame False {
              }
              frame True {
                n269 = local read "state 3.1"() -> (w778:enum16{"waiting", "sound", "ITI"})
                n270 = case shown="\"ITI\"" w778 {
                  frame "waiting", Default {
                    w785 = 0.0 ("element")
                    n271 = local read "water # 3.2R"() -> (w787:dbl)
                    n272 = local read "water # 3.1L"() -> (w789:dbl)
                    n273 = local read "lick # 3.1L"() -> (w792:dbl)
                    n274 = local write "state 3.2"(enum16{"waiting", "sound", "ITI"}."ITI") -> ()
                    n275 = local read "lick # 3.2R"() -> (w790:dbl)
                    n276 = local write "state 3.1"(enum16{"waiting", "sound", "ITI"}."ITI") -> ()
                    n277 = local read "time (s)"() -> (w786:dbl)
                    n278 = local read "current sound"() -> (w781:dbl)
                    n279 = Increment(x=w792) -> (x+1=w791:dbl)
                    n280 = Increment(x=w789) -> (x+1=w788:dbl)
                    n281 = local read "trial #"() -> (w782:dbl)
                    n282 = local read "mistake # 3.2R"() -> (w783:dbl)
                    n283 = local read "free water 3.1"() -> (w796:bool)
                    n284 = local write "water # 3.1L"(w788) -> ()
                    n285 = local write "lick # 3.1L"(w791) -> ()
                    n286 = local write "last water 3.1L"(w786) -> ()
                    n287 = local read "ITI (s)"() -> (w780:dbl)
                    n288 = local read "mistake # 3.1L"() -> (w784:dbl)
                    n289 = local read "Mouse path 3"() -> (w795:path)
                    n290 = case shown="False" w796 {
                      frame False {
                        n291 = local read "water dur (ms) 3.1"() -> (w799:dbl)
                        n292 = local read "water port 3.1"() -> (w800:tag)
                        n293 = call "_digital_on_duration_off.vi"("duration (ms)"=w799, "digital port"=w800) -> ()  [unwired: 10 in]
                      }
                      frame True {
                      }
                    }
                    n294 = Build Array(w786, w791, w790, w788, w787, 1.0 ("element"), w785, w782, w781, w780, w785, w784, w783) -> (w793:dbl[])
                    n295 = call-poly <vilib>:"Write To Spreadsheet File.vi"("append to file? (new file:F)"=TRUE, "1D data"=w793, "file path (dialog if empty)"=w795) -> ()  [unwired: 5 in, 1 out]
                  }
                  frame "sound" {
                    w806 = 0.0 ("element")
                    n296 = local read "lick # 3.2R"() -> (w809:dbl)
                    n297 = local read "water # 3.2R"() -> (w807:dbl)
                    n298 = local read "water # 3.1L"() -> (w808:dbl)
                    n299 = local read "current sound"() -> (w802:dbl)
                    n300 = local read "lick # 3.1L"() -> (w811:dbl)
                    n301 = local read "trial #"() -> (w803:dbl)
                    n302 = local read "ITI (s)"() -> (w801:dbl)
                    n303 = Increment(x=w811) -> (x+1=w810:dbl)
                    n304 = local read "mistake # 3.2R"() -> (w804:dbl)
                    n305 = local read "time (s)"() -> (w812:dbl)
                    n306 = local read "mistake # 3.1L"() -> (w805:dbl)
                    n307 = local write "lick # 3.1L"(w810) -> ()
                    n308 = local read "Mouse path 3"() -> (w814:path)
                    n309 = Build Array(w812, w810, w809, w808, w807, w806, w806, w803, w802, w801, w806, w805, w804) -> (w813:dbl[])
                    n310 = call-poly <vilib>:"Write To Spreadsheet File.vi"("append to file? (new file:F)"=TRUE, "1D data"=w813, "file path (dialog if empty)"=w814) -> ()  [unwired: 5 in, 1 out]
                  }
                  frame "ITI" {
                    w821 = 0.0 ("element")
                    n311 = local read "water # 3.2R"() -> (w822:dbl)
                    n312 = local read "water # 3.1L"() -> (w823:dbl)
                    n313 = local read "lick # 3.2R"() -> (w824:dbl)
                    n314 = local read "lick # 3.1L"() -> (w826:dbl)
                    n315 = local read "current sound"() -> (w817:dbl)
                    n316 = local read "trial #"() -> (w818:dbl)
                    n317 = local read "ITI (s)"() -> (w816:dbl)
                    n318 = local read "time (s)"() -> (w827:dbl)
                    n319 = local read "mistake # 3.2R"() -> (w819:dbl)
                    n320 = local read "mistake # 3.1L"() -> (w820:dbl)
                    n321 = Increment(x=w826) -> (x+1=w825:dbl)
                    n322 = local write "lick # 3.1L"(w825) -> ()
                    n323 = local read "Mouse path 3"() -> (w829:path)
                    n324 = Build Array(w827, w825, w824, w823, w822, w821, w821, w818, w817, w816, w821, w820, w819) -> (w828:dbl[])
                    n325 = call-poly <vilib>:"Write To Spreadsheet File.vi"("append to file? (new file:F)"=TRUE, "1D data"=w828, "file path (dialog if empty)"=w829) -> ()  [unwired: 5 in, 1 out]
                  }
                }
              }
            }
            n326 = case shown="True" w725 {
              frame False {
              }
              frame True {
                n327 = local read "state 3.1"() -> (w727:enum16{"waiting", "sound", "ITI"})
                n328 = case shown="\"ITI\"" w727 {
                  frame "waiting", Default {
                    w736 = 0.0 ("element")
                    n329 = local write "state 3.2"(enum16{"waiting", "sound", "ITI"}."ITI") -> ()
                    n330 = local write "state 3.1"(enum16{"waiting", "sound", "ITI"}."ITI") -> ()
                    n331 = local read "current sound"() -> (w729:dbl)
                    n332 = local read "trial #"() -> (w730:dbl)
                    n333 = local read "ITI (s)"() -> (w728:dbl)
                    n334 = local read "lick # 3.2R"() -> (w740:dbl)
                    n335 = local read "water # 3.2R"() -> (w737:dbl)
                    n336 = local read "water # 3.1L"() -> (w738:dbl)
                    n337 = local read "mistake # 3.1L"() -> (w735:dbl)
                    n338 = local read "mistake # 3.2R"() -> (w733:dbl)
                    n339 = local read "lick # 3.1L"() -> (w741:dbl)
                    n340 = local read "time (s)"() -> (w742:dbl)
                    n341 = Increment(x=w740) -> (x+1=w739:dbl)
                    n342 = Increment(x=w735) -> (x+1=w734:dbl)
                    n343 = local write "lick # 3.2R"(w739) -> ()
                    n344 = local write "mistake # 3.1L"(w734) -> ()
                    n345 = local read "Mouse path 3"() -> (w743:path)
                    n346 = Build Array(w742, w741, w739, w738, w737, w736, w736, w730, w729, w728, w736, w734, w733) -> (w744:dbl[])
                    n347 = call-poly <vilib>:"Write To Spreadsheet File.vi"("append to file? (new file:F)"=TRUE, "1D data"=w744, "file path (dialog if empty)"=w743) -> ()  [unwired: 5 in, 1 out]
                    n348 = local read "LED 3"() -> (w732:tag)
                    n349 = local write "LED 3 (i)"(1.0 ("LED 3 (i)")) -> ()
                    n350 = call "_digital_on.vi"("digital port"=w732) -> ()  [unwired: 11 in]
                  }
                  frame "sound" {
                    w753 = 0.0 ("element")
                    n351 = local read "current sound"() -> (w749:dbl)
                    n352 = local read "water # 3.2R"() -> (w754:dbl)
                    n353 = local read "trial #"() -> (w750:dbl)
                    n354 = local read "ITI (s)"() -> (w748:dbl)
                    n355 = local read "water # 3.1L"() -> (w755:dbl)
                    n356 = local read "lick # 3.2R"() -> (w757:dbl)
                    n357 = local read "mistake # 3.2R"() -> (w751:dbl)
                    n358 = local read "lick # 3.1L"() -> (w758:dbl)
                    n359 = local read "mistake # 3.1L"() -> (w752:dbl)
                    n360 = local read "time (s)"() -> (w759:dbl)
                    n361 = Increment(x=w757) -> (x+1=w756:dbl)
                    n362 = local read "Mouse path 3"() -> (w761:path)
                    n363 = local write "lick # 3.2R"(w756) -> ()
                    n364 = Build Array(w759, w758, w756, w755, w754, w753, w753, w750, w749, w748, w753, w752, w751) -> (w760:dbl[])
                    n365 = call-poly <vilib>:"Write To Spreadsheet File.vi"("append to file? (new file:F)"=TRUE, "1D data"=w760, "file path (dialog if empty)"=w761) -> ()  [unwired: 5 in, 1 out]
                  }
                  frame "ITI" {
                    w768 = 0.0 ("element")
                    n366 = local read "current sound"() -> (w764:dbl)
                    n367 = local read "lick # 3.2R"() -> (w772:dbl)
                    n368 = local read "water # 3.2R"() -> (w769:dbl)
                    n369 = local read "water # 3.1L"() -> (w770:dbl)
                    n370 = local read "lick # 3.1L"() -> (w773:dbl)
                    n371 = local read "trial #"() -> (w765:dbl)
                    n372 = local read "ITI (s)"() -> (w763:dbl)
                    n373 = local read "mistake # 3.1L"() -> (w767:dbl)
                    n374 = local read "mistake # 3.2R"() -> (w766:dbl)
                    n375 = Increment(x=w772) -> (x+1=w771:dbl)
                    n376 = local read "time (s)"() -> (w774:dbl)
                    n377 = local write "lick # 3.2R"(w771) -> ()
                    n378 = local read "Mouse path 3"() -> (w776:path)
                    n379 = Build Array(w774, w773, w771, w770, w769, w768, w768, w765, w764, w763, w768, w767, w766) -> (w775:dbl[])
                    n380 = call-poly <vilib>:"Write To Spreadsheet File.vi"("append to file? (new file:F)"=TRUE, "1D data"=w775, "file path (dialog if empty)"=w776) -> ()  [unwired: 5 in, 1 out]
                  }
                }
              }
            }
          }
          frame 4 {
            n381 = case shown="True" w832 {
              frame False {
              }
              frame True {
                n382 = local read "state 3.2"() -> (w886:enum16{"waiting", "sound", "ITI"})
                n383 = case shown="\"ITI\"" w886 {
                  frame "waiting", Default {
                    w895 = 0.0 ("element")
                    n384 = local read "current sound"() -> (w888:dbl)
                    n385 = local read "mistake # 3.2R"() -> (w893:dbl)
                    n386 = local read "trial #"() -> (w889:dbl)
                    n387 = local read "mistake # 3.1L"() -> (w894:dbl)
                    n388 = local read "water # 3.2R"() -> (w896:dbl)
                    n389 = local read "water # 3.1L"() -> (w897:dbl)
                    n390 = local read "ITI (s)"() -> (w887:dbl)
                    n391 = local read "lick # 3.2R"() -> (w898:dbl)
                    n392 = local read "lick # 3.1L"() -> (w900:dbl)
                    n393 = local write "state 3.2"(enum16{"waiting", "sound", "ITI"}."ITI") -> ()
                    n394 = local read "LED 3"() -> (w890:tag)
                    n395 = local write "state 3.1"(enum16{"waiting", "sound", "ITI"}."ITI") -> ()
                    n396 = local write "LED 3 (i)"(1.0 ("LED 3 (i)")) -> ()
                    n397 = local read "time (s)"() -> (w901:dbl)
                    n398 = Increment(x=w893) -> (x+1=w892:dbl)
                    n399 = Increment(x=w900) -> (x+1=w899:dbl)
                    n400 = local write "mistake # 3.2R"(w892) -> ()
                    n401 = local write "lick # 3.1L"(w899) -> ()
                    n402 = local read "Mouse path 3"() -> (w903:path)
                    n403 = Build Array(w901, w899, w898, w897, w896, w895, w895, w889, w888, w887, w895, w894, w892) -> (w902:dbl[])
                    n404 = call "_digital_on.vi"("digital port"=w890) -> ()  [unwired: 11 in]
                    n405 = call-poly <vilib>:"Write To Spreadsheet File.vi"("append to file? (new file:F)"=TRUE, "1D data"=w902, "file path (dialog if empty)"=w903) -> ()  [unwired: 5 in, 1 out]
                  }
                  frame "sound" {
                    w912 = 0.0 ("element")
                    n406 = local read "current sound"() -> (w908:dbl)
                    n407 = local read "mistake # 3.2R"() -> (w910:dbl)
                    n408 = local read "water # 3.2R"() -> (w913:dbl)
                    n409 = local read "trial #"() -> (w909:dbl)
                    n410 = local read "mistake # 3.1L"() -> (w911:dbl)
                    n411 = local read "ITI (s)"() -> (w907:dbl)
                    n412 = local read "water # 3.1L"() -> (w914:dbl)
                    n413 = local read "lick # 3.2R"() -> (w915:dbl)
                    n414 = local read "lick # 3.1L"() -> (w917:dbl)
                    n415 = local read "time (s)"() -> (w918:dbl)
                    n416 = Increment(x=w917) -> (x+1=w916:dbl)
                    n417 = local read "Mouse path 3"() -> (w920:path)
                    n418 = local write "lick # 3.1L"(w916) -> ()
                    n419 = Build Array(w918, w916, w915, w914, w913, w912, w912, w909, w908, w907, w912, w911, w910) -> (w919:dbl[])
                    n420 = call-poly <vilib>:"Write To Spreadsheet File.vi"("append to file? (new file:F)"=TRUE, "1D data"=w919, "file path (dialog if empty)"=w920) -> ()  [unwired: 5 in, 1 out]
                  }
                  frame "ITI" {
                    w927 = 0.0 ("element")
                    n421 = local read "water # 3.1L"() -> (w929:dbl)
                    n422 = local read "water # 3.2R"() -> (w928:dbl)
                    n423 = local read "current sound"() -> (w923:dbl)
                    n424 = local read "lick # 3.2R"() -> (w930:dbl)
                    n425 = local read "lick # 3.1L"() -> (w932:dbl)
                    n426 = local read "trial #"() -> (w924:dbl)
                    n427 = local read "ITI (s)"() -> (w922:dbl)
                    n428 = local read "mistake # 3.1L"() -> (w926:dbl)
                    n429 = local read "mistake # 3.2R"() -> (w925:dbl)
                    n430 = local read "time (s)"() -> (w933:dbl)
                    n431 = Increment(x=w932) -> (x+1=w931:dbl)
                    n432 = local write "lick # 3.1L"(w931) -> ()
                    n433 = Build Array(w933, w931, w930, w929, w928, w927, w927, w924, w923, w922, w927, w926, w925) -> (w934:dbl[])
                    n434 = local read "Mouse path 3"() -> (w935:path)
                    n435 = call-poly <vilib>:"Write To Spreadsheet File.vi"("append to file? (new file:F)"=TRUE, "1D data"=w934, "file path (dialog if empty)"=w935) -> ()  [unwired: 5 in, 1 out]
                  }
                }
              }
            }
            n436 = case shown="True" w831 {
              frame False {
              }
              frame True {
                n437 = local read "state 3.2"() -> (w833:enum16{"waiting", "sound", "ITI"})
                n438 = case shown="\"ITI\"" w833 {
                  frame "waiting", Default {
                    w842 = 0.0 ("element")
                    n439 = local read "lick # 3.2R"() -> (w847:dbl)
                    n440 = local read "water # 3.2R"() -> (w844:dbl)
                    n441 = local read "water # 3.1L"() -> (w845:dbl)
                    n442 = local read "current sound"() -> (w835:dbl)
                    n443 = local read "lick # 3.1L"() -> (w848:dbl)
                    n444 = local read "trial #"() -> (w836:dbl)
                    n445 = local read "mistake # 3.1L"() -> (w841:dbl)
                    n446 = local read "mistake # 3.2R"() -> (w840:dbl)
                    n447 = local read "time (s)"() -> (w838:dbl)
                    n448 = local read "ITI (s)"() -> (w834:dbl)
                    n449 = Increment(x=w847) -> (x+1=w846:dbl)
                    n450 = Increment(x=w844) -> (x+1=w843:dbl)
                    n451 = local write "water # 3.2R"(w843) -> ()
                    n452 = local write "state 3.2"(enum16{"waiting", "sound", "ITI"}."ITI") -> ()
                    n453 = local write "state 3.1"(enum16{"waiting", "sound", "ITI"}."ITI") -> ()
                    n454 = local write "last water 3.2R"(w838) -> ()
                    n455 = local write "lick # 3.2R"(w846) -> ()
                    n456 = local read "Mouse path 3"() -> (w850:path)
                    n457 = local read "free water 3.2"() -> (w839:bool)
                    n458 = Build Array(w838, w848, w846, w845, w843, 1.0 ("element"), w842, w836, w835, w834, w842, w841, w840) -> (w849:dbl[])
                    n459 = call-poly <vilib>:"Write To Spreadsheet File.vi"("append to file? (new file:F)"=TRUE, "1D data"=w849, "file path (dialog if empty)"=w850) -> ()  [unwired: 5 in, 1 out]
                    n460 = case shown="False" w839 {
                      frame False {
                        n461 = local read "water dur (ms) 3. 2"() -> (w855:dbl)
                        n462 = local read "water port 3.2"() -> (w854:tag)
                        n463 = call "_digital_on_duration_off.vi"("duration (ms)"=w855, "digital port"=w854) -> ()  [unwired: 10 in]
                      }
                      frame True {
                      }
                    }
                  }
                  frame "sound" {
                    w861 = 0.0 ("element")
                    n464 = local read "water # 3.2R"() -> (w862:dbl)
                    n465 = local read "water # 3.1L"() -> (w863:dbl)
                    n466 = local read "lick # 3.2R"() -> (w865:dbl)
                    n467 = local read "current sound"() -> (w857:dbl)
                    n468 = local read "lick # 3.1L"() -> (w866:dbl)
                    n469 = local read "trial #"() -> (w858:dbl)
                    n470 = local read "ITI (s)"() -> (w856:dbl)
                    n471 = local read "mistake # 3.2R"() -> (w859:dbl)
                    n472 = local read "time (s)"() -> (w867:dbl)
                    n473 = local read "mistake # 3.1L"() -> (w860:dbl)
                    n474 = Increment(x=w865) -> (x+1=w864:dbl)
                    n475 = local write "lick # 3.2R"(w864) -> ()
                    n476 = local read "Mouse path 3"() -> (w869:path)
                    n477 = Build Array(w867, w866, w864, w863, w862, w861, w861, w858, w857, w856, w861, w860, w859) -> (w868:dbl[])
                    n478 = call-poly <vilib>:"Write To Spreadsheet File.vi"("append to file? (new file:F)"=TRUE, "1D data"=w868, "file path (dialog if empty)"=w869) -> ()  [unwired: 5 in, 1 out]
                  }
                  frame "ITI" {
                    w876 = 0.0 ("element")
                    n479 = local read "water # 3.2R"() -> (w877:dbl)
                    n480 = local read "lick # 3.2R"() -> (w880:dbl)
                    n481 = local read "water # 3.1L"() -> (w878:dbl)
                    n482 = local read "current sound"() -> (w872:dbl)
                    n483 = local read "ITI (s)"() -> (w871:dbl)
                    n484 = local read "trial #"() -> (w873:dbl)
                    n485 = local read "lick # 3.1L"() -> (w881:dbl)
                    n486 = local read "time (s)"() -> (w882:dbl)
                    n487 = local read "mistake # 3.2R"() -> (w874:dbl)
                    n488 = local read "mistake # 3.1L"() -> (w875:dbl)
                    n489 = Increment(x=w880) -> (x+1=w879:dbl)
                    n490 = local write "lick # 3.2R"(w879) -> ()
                    n491 = local read "Mouse path 3"() -> (w884:path)
                    n492 = Build Array(w882, w881, w879, w878, w877, w876, w876, w873, w872, w871, w876, w875, w874) -> (w883:dbl[])
                    n493 = call-poly <vilib>:"Write To Spreadsheet File.vi"("append to file? (new file:F)"=TRUE, "1D data"=w883, "file path (dialog if empty)"=w884) -> ()  [unwired: 5 in, 1 out]
                  }
                }
              }
            }
          }
        }
        n494 = case shown="4" w65 {
          tunnel: w61 -> [_ w938 w1044 w1150 w1256]
          tunnel: w62 -> [_ w937 w1043 w1149 w1255]
          frame 0, Default {
          }
          frame 1 {
            n495 = case shown="True" w938 {
              frame False {
              }
              frame True {
                n496 = local read "state 2.1"() -> (w990:enum16{"waiting", "sound", "ITI"})
                n497 = case shown="\"waiting\", Default" w990 {
                  frame "waiting", Default {
                    w992 = 0.0 ("element")
                    n498 = local read "free water 2.1"() -> (w996:bool)
                    n499 = case shown="False" w996 {
                      frame False {
                        n500 = call "_digital_on_duration_off.vi"("duration (ms)"="water dur (ms) 2.1", "digital port"="water port 2.1") -> ()  [unwired: 10 in]
                      }
                      frame True {
                      }
                    }
                    n501 = local write "state 2.2"(enum16{"waiting", "sound", "ITI"}."ITI") -> ()
                    n502 = local write "state 2.1"(enum16{"waiting", "sound", "ITI"}."ITI") -> ()
                    n503 = local read "lick  #  2.1L"() -> (w1005:dbl)
                    n504 = local read "water # 2.2R"() -> (w1000:dbl)
                    n505 = local read "water # 2.1L"() -> (w1002:dbl)
                    n506 = local read "lick  #  2.2R"() -> (w1003:dbl)
                    n507 = local read "current sound"() -> (w994:dbl)
                    n508 = Increment(x=w1005) -> (x+1=w1004:dbl)
                    n509 = local read "mistake # 2.2R"() -> (w998:dbl)
                    n510 = local read "mistake # 2.1L"() -> (w999:dbl)
                    n511 = Increment(x=w1002) -> (x+1=w1001:dbl)
                    n512 = local read "time (s)"() -> (w997:dbl)
                    n513 = local read "trial #"() -> (w995:dbl)
                    n514 = local read "ITI (s)"() -> (w993:dbl)
                    n515 = local write "lick  #  2.1L"(w1004) -> ()
                    n516 = local write "water # 2.1L"(w1001) -> ()
                    n517 = local write "last water 2.1L"(w997) -> ()
                    n518 = local read "Mouse path 2"() -> (w1008:path)
                    n519 = Build Array(w997, w1004, w1003, w1001, w1000, 1.0 ("element"), w992, w995, w994, w993, w992, w999, w998) -> (w1006:dbl[])
                    n520 = call-poly <vilib>:"Write To Spreadsheet File.vi"("append to file? (new file:F)"=TRUE, "1D data"=w1006, "file path (dialog if empty)"=w1008) -> ()  [unwired: 5 in, 1 out]
                  }
                  frame "sound" {
                    w1018 = 0.0 ("element")
                    n521 = local read "water # 2.2R"() -> (w1019:dbl)
                    n522 = local read "water # 2.1L"() -> (w1020:dbl)
                    n523 = local read "lick  #  2.2R"() -> (w1021:dbl)
                    n524 = local read "lick  #  2.1L"() -> (w1023:dbl)
                    n525 = local read "current sound"() -> (w1014:dbl)
                    n526 = local read "trial #"() -> (w1015:dbl)
                    n527 = local read "ITI (s)"() -> (w1013:dbl)
                    n528 = local read "mistake # 2.2R"() -> (w1016:dbl)
                    n529 = local read "mistake # 2.1L"() -> (w1017:dbl)
                    n530 = local read "time (s)"() -> (w1024:dbl)
                    n531 = Increment(x=w1023) -> (x+1=w1022:dbl)
                    n532 = local write "lick  #  2.1L"(w1022) -> ()
                    n533 = local read "Mouse path 2"() -> (w1027:path)
                    n534 = Build Array(w1024, w1022, w1021, w1020, w1019, w1018, w1018, w1015, w1014, w1013, w1018, w1017, w1016) -> (w1025:dbl[])
                    n535 = call-poly <vilib>:"Write To Spreadsheet File.vi"("append to file? (new file:F)"=TRUE, "1D data"=w1025, "file path (dialog if empty)"=w1027) -> ()  [unwired: 5 in, 1 out]
                  }
                  frame "ITI" {
                    w1033 = 0.0 ("element")
                    n536 = local read "water # 2.2R"() -> (w1034:dbl)
                    n537 = local read "water # 2.1L"() -> (w1035:dbl)
                    n538 = local read "lick  #  2.2R"() -> (w1036:dbl)
                    n539 = local read "current sound"() -> (w1029:dbl)
                    n540 = local read "lick  #  2.1L"() -> (w1038:dbl)
                    n541 = local read "trial #"() -> (w1030:dbl)
                    n542 = local read "ITI (s)"() -> (w1028:dbl)
                    n543 = local read "time (s)"() -> (w1039:dbl)
                    n544 = Increment(x=w1038) -> (x+1=w1037:dbl)
                    n545 = local read "mistake # 2.2R"() -> (w1031:dbl)
                    n546 = local read "mistake # 2.1L"() -> (w1032:dbl)
                    n547 = local write "lick  #  2.1L"(w1037) -> ()
                    n548 = local read "Mouse path 2"() -> (w1041:path)
                    n549 = Build Array(w1039, w1037, w1036, w1035, w1034, w1033, w1033, w1030, w1029, w1028, w1033, w1032, w1031) -> (w1040:dbl[])
                    n550 = call-poly <vilib>:"Write To Spreadsheet File.vi"("append to file? (new file:F)"=TRUE, "1D data"=w1040, "file path (dialog if empty)"=w1041) -> ()  [unwired: 5 in, 1 out]
                  }
                }
              }
            }
            n551 = case shown="True" w937 {
              frame False {
              }
              frame True {
                n552 = local read "state 2.1"() -> (w939:enum16{"waiting", "sound", "ITI"})
                n553 = case shown="\"waiting\", Default" w939 {
                  frame "waiting", Default {
                    w948 = 0.0 ("element")
                    n554 = local write "LED 2 (i)"(1.0 ("LED 2 (i)")) -> ()
                    n555 = local read "water # 2.2R"() -> (w949:dbl)
                    n556 = local read "lick  #  2.2R"() -> (w953:dbl)
                    n557 = local read "water # 2.1L"() -> (w950:dbl)
                    n558 = local read "mistake # 2.1L"() -> (w947:dbl)
                    n559 = local read "lick  #  2.1L"() -> (w952:dbl)
                    n560 = local read "mistake # 2.2R"() -> (w945:dbl)
                    n561 = local read "current sound"() -> (w941:dbl)
                    n562 = local read "trial #"() -> (w942:dbl)
                    n563 = local write "state 2.2"(enum16{"waiting", "sound", "ITI"}."ITI") -> ()
                    n564 = local read "time (s)"() -> (w954:dbl)
                    n565 = Increment(x=w953) -> (x+1=w951:dbl)
                    n566 = local read "ITI (s)"() -> (w940:dbl)
                    n567 = Increment(x=w947) -> (x+1=w946:dbl)
                    n568 = local write "state 2.1"(enum16{"waiting", "sound", "ITI"}."ITI") -> ()
                    n569 = local write "lick  #  2.2R"(w951) -> ()
                    n570 = local write "mistake # 2.1L"(w946) -> ()
                    n571 = local read "Mouse path 2"() -> (w957:path)
                    n572 = Build Array(w954, w952, w951, w950, w949, w948, w948, w942, w941, w940, w948, w946, w945) -> (w956:dbl[])
                    n573 = call-poly <vilib>:"Write To Spreadsheet File.vi"("append to file? (new file:F)"=TRUE, "1D data"=w956, "file path (dialog if empty)"=w957) -> ()  [unwired: 5 in, 1 out]
                    n574 = call "_digital_on.vi"("digital port"="LED 2") -> ()  [unwired: 11 in]
                  }
                  frame "ITI" {
                    w965 = 0.0 ("element")
                    n575 = local read "water # 2.2R"() -> (w966:dbl)
                    n576 = local read "lick  #  2.2R"() -> (w969:dbl)
                    n577 = local read "water # 2.1L"() -> (w967:dbl)
                    n578 = local read "current sound"() -> (w961:dbl)
                    n579 = local read "lick  #  2.1L"() -> (w970:dbl)
                    n580 = Increment(x=w969) -> (x+1=w968:dbl)
                    n581 = local read "trial #"() -> (w962:dbl)
                    n582 = local read "time (s)"() -> (w971:dbl)
                    n583 = local read "ITI (s)"() -> (w960:dbl)
                    n584 = local read "mistake # 2.2R"() -> (w963:dbl)
                    n585 = local write "lick  #  2.2R"(w968) -> ()
                    n586 = local read "mistake # 2.1L"() -> (w964:dbl)
                    n587 = local read "Mouse path 2"() -> (w973:path)
                    n588 = Build Array(w971, w970, w968, w967, w966, w965, w965, w962, w961, w960, w965, w964, w963) -> (w972:dbl[])
                    n589 = call-poly <vilib>:"Write To Spreadsheet File.vi"("append to file? (new file:F)"=TRUE, "1D data"=w972, "file path (dialog if empty)"=w973) -> ()  [unwired: 5 in, 1 out]
                  }
                  frame "sound" {
                    w980 = 0.0 ("element")
                    n590 = local read "water # 2.2R"() -> (w981:dbl)
                    n591 = local read "water # 2.1L"() -> (w982:dbl)
                    n592 = local read "lick  #  2.2R"() -> (w984:dbl)
                    n593 = local read "lick  #  2.1L"() -> (w985:dbl)
                    n594 = local read "current sound"() -> (w976:dbl)
                    n595 = local read "trial #"() -> (w977:dbl)
                    n596 = Increment(x=w984) -> (x+1=w983:dbl)
                    n597 = local read "ITI (s)"() -> (w975:dbl)
                    n598 = local read "time (s)"() -> (w986:dbl)
                    n599 = local write "lick  #  2.2R"(w983) -> ()
                    n600 = local read "mistake # 2.2R"() -> (w978:dbl)
                    n601 = local read "mistake # 2.1L"() -> (w979:dbl)
                    n602 = local read "Mouse path 2"() -> (w988:path)
                    n603 = Build Array(w986, w985, w983, w982, w981, w980, w980, w977, w976, w975, w980, w979, w978) -> (w987:dbl[])
                    n604 = call-poly <vilib>:"Write To Spreadsheet File.vi"("append to file? (new file:F)"=TRUE, "1D data"=w987, "file path (dialog if empty)"=w988) -> ()  [unwired: 5 in, 1 out]
                  }
                }
              }
            }
          }
          frame 2 {
            n605 = case shown="True" w1044 {
              frame False {
              }
              frame True {
                n606 = local read "state 2.2"() -> (w1098:enum16{"waiting", "sound", "ITI"})
                n607 = case shown="\"waiting\", Default" w1098 {
                  frame "waiting", Default {
                    w1107 = 0.0 ("element")
                    n608 = local read "LED 2"() -> (w1102:tag)
                    n609 = local write "state 2.2"(enum16{"waiting", "sound", "ITI"}."ITI") -> ()
                    n610 = local write "state 2.1"(enum16{"waiting", "sound", "ITI"}."ITI") -> ()
                    n611 = local read "current sound"() -> (w1100:dbl)
                    n612 = local read "water # 2.2R"() -> (w1108:dbl)
                    n613 = local read "water # 2.1L"() -> (w1109:dbl)
                    n614 = local read "trial #"() -> (w1101:dbl)
                    n615 = local read "lick  #  2.2R"() -> (w1110:dbl)
                    n616 = local read "lick  #  2.1L"() -> (w1112:dbl)
                    n617 = local read "mistake # 2.2R"() -> (w1105:dbl)
                    n618 = call "_digital_on.vi"("digital port"=w1102) -> ()  [unwired: 11 in]
                    n619 = local read "ITI (s)"() -> (w1099:dbl)
                    n620 = local read "mistake # 2.1L"() -> (w1106:dbl)
                    n621 = local read "time (s)"() -> (w1113:dbl)
                    n622 = Increment(x=w1112) -> (x+1=w1111:dbl)
                    n623 = Increment(x=w1105) -> (x+1=w1104:dbl)
                    n624 = local write "lick  #  2.1L"(w1111) -> ()
                    n625 = local read "Mouse path 2"() -> (w1115:path)
                    n626 = local write "mistake # 2.2R"(w1104) -> ()
                    n627 = Build Array(w1113, w1111, w1110, w1109, w1108, w1107, w1107, w1101, w1100, w1099, w1107, w1106, w1104) -> (w1114:dbl[])
                    n628 = local write "LED 2 (i)"(1.0 ("LED 2 (i)")) -> ()
                    n629 = call-poly <vilib>:"Write To Spreadsheet File.vi"("append to file? (new file:F)"=TRUE, "1D data"=w1114, "file path (dialog if empty)"=w1115) -> ()  [unwired: 5 in, 1 out]
                  }
                  frame "sound" {
                    w1124 = 0.0 ("element")
                    n630 = local read "water # 2.2R"() -> (w1125:dbl)
                    n631 = local read "current sound"() -> (w1120:dbl)
                    n632 = local read "water # 2.1L"() -> (w1126:dbl)
                    n633 = local read "lick  #  2.2R"() -> (w1127:dbl)
                    n634 = local read "lick  #  2.1L"() -> (w1129:dbl)
                    n635 = local read "trial #"() -> (w1121:dbl)
                    n636 = local read "ITI (s)"() -> (w1119:dbl)
                    n637 = local read "mistake # 2.2R"() -> (w1122:dbl)
                    n638 = local read "mistake # 2.1L"() -> (w1123:dbl)
                    n639 = Increment(x=w1129) -> (x+1=w1128:dbl)
                    n640 = local read "time (s)"() -> (w1130:dbl)
                    n641 = local write "lick  #  2.1L"(w1128) -> ()
                    n642 = local read "Mouse path 2"() -> (w1132:path)
                    n643 = Build Array(w1130, w1128, w1127, w1126, w1125, w1124, w1124, w1121, w1120, w1119, w1124, w1123, w1122) -> (w1131:dbl[])
                    n644 = call-poly <vilib>:"Write To Spreadsheet File.vi"("append to file? (new file:F)"=TRUE, "1D data"=w1131, "file path (dialog if empty)"=w1132) -> ()  [unwired: 5 in, 1 out]
                  }
                  frame "ITI" {
                    w1139 = 0.0 ("element")
                    n645 = local read "water # 2.2R"() -> (w1140:dbl)
                    n646 = local read "water # 2.1L"() -> (w1141:dbl)
                    n647 = local read "lick  #  2.1L"() -> (w1144:dbl)
                    n648 = local read "lick  #  2.2R"() -> (w1142:dbl)
                    n649 = local read "current sound"() -> (w1135:dbl)
                    n650 = local read "time (s)"() -> (w1145:dbl)
                    n651 = local read "trial #"() -> (w1136:dbl)
                    n652 = Increment(x=w1144) -> (x+1=w1143:dbl)
                    n653 = local read "ITI (s)"() -> (w1134:dbl)
                    n654 = local read "mistake # 2.2R"() -> (w1137:dbl)
                    n655 = local read "mistake # 2.1L"() -> (w1138:dbl)
                    n656 = local write "lick  #  2.1L"(w1143) -> ()
                    n657 = local read "Mouse path 2"() -> (w1147:path)
                    n658 = Build Array(w1145, w1143, w1142, w1141, w1140, w1139, w1139, w1136, w1135, w1134, w1139, w1138, w1137) -> (w1146:dbl[])
                    n659 = call-poly <vilib>:"Write To Spreadsheet File.vi"("append to file? (new file:F)"=TRUE, "1D data"=w1146, "file path (dialog if empty)"=w1147) -> ()  [unwired: 5 in, 1 out]
                  }
                }
              }
            }
            n660 = case shown="True" w1043 {
              frame False {
              }
              frame True {
                n661 = local read "state 2.2"() -> (w1045:enum16{"waiting", "sound", "ITI"})
                n662 = case shown="\"waiting\", Default" w1045 {
                  frame "waiting", Default {
                    w1056 = 0.0 ("element")
                    n663 = local read "water # 2.2R"() -> (w1051:dbl)
                    n664 = local read "water # 2.1L"() -> (w1057:dbl)
                    n665 = local read "lick  #  2.2R"() -> (w1059:dbl)
                    n666 = local read "lick  #  2.1L"() -> (w1060:dbl)
                    n667 = local read "current sound"() -> (w1048:dbl)
                    n668 = local read "time (s)"() -> (w1053:dbl)
                    n669 = Increment(x=w1051) -> (x+1=w1050:dbl)
                    n670 = Increment(x=w1059) -> (x+1=w1058:dbl)
                    n671 = local read "trial #"() -> (w1049:dbl)
                    n672 = local read "ITI (s)"() -> (w1047:dbl)
                    n673 = local read "mistake # 2.2R"() -> (w1054:dbl)
                    n674 = local write "water # 2.2R"(w1050) -> ()
                    n675 = local read "mistake # 2.1L"() -> (w1055:dbl)
                    n676 = local read "free water 2.2"() -> (w1052:bool)
                    n677 = local write "lick  #  2.2R"(w1058) -> ()
                    n678 = local write "last water 2.2R"(w1053) -> ()
                    n679 = local read "Mouse path 2"() -> (w1062:path)
                    n680 = Build Array(w1053, w1060, w1058, w1057, w1050, 1.0 ("element"), w1056, w1049, w1048, w1047, w1056, w1055, w1054) -> (w1061:dbl[])
                    n681 = case shown="False" w1052 {
                      frame False {
                        n682 = call "_digital_on_duration_off.vi"("duration (ms)"="water dur (ms) 2.2", "digital port"="water port 2.2") -> ()  [unwired: 10 in]
                      }
                      frame True {
                      }
                    }
                    n683 = local write "state 2.2"(enum16{"waiting", "sound", "ITI"}."ITI") -> ()
                    n684 = call-poly <vilib>:"Write To Spreadsheet File.vi"("append to file? (new file:F)"=TRUE, "1D data"=w1061, "file path (dialog if empty)"=w1062) -> ()  [unwired: 5 in, 1 out]
                    n685 = local write "state 2.1"(enum16{"waiting", "sound", "ITI"}."ITI") -> ()
                  }
                  frame "ITI" {
                    w1073 = 0.0 ("element")
                    n686 = local read "water # 2.2R"() -> (w1074:dbl)
                    n687 = local read "water # 2.1L"() -> (w1075:dbl)
                    n688 = local read "current sound"() -> (w1069:dbl)
                    n689 = local read "lick  #  2.2R"() -> (w1077:dbl)
                    n690 = local read "lick  #  2.1L"() -> (w1078:dbl)
                    n691 = local read "trial #"() -> (w1070:dbl)
                    n692 = local read "ITI (s)"() -> (w1068:dbl)
                    n693 = Increment(x=w1077) -> (x+1=w1076:dbl)
                    n694 = local read "mistake # 2.2R"() -> (w1071:dbl)
                    n695 = local read "mistake # 2.1L"() -> (w1072:dbl)
                    n696 = local write "lick  #  2.2R"(w1076) -> ()
                    n697 = local read "time (s)"() -> (w1079:dbl)
                    n698 = local read "Mouse path 2"() -> (w1082:path)
                    n699 = Build Array(w1079, w1078, w1076, w1075, w1074, w1073, w1073, w1070, w1069, w1068, w1073, w1072, w1071) -> (w1080:dbl[])
                    n700 = call-poly <vilib>:"Write To Spreadsheet File.vi"("append to file? (new file:F)"=TRUE, "1D data"=w1080, "file path (dialog if empty)"=w1082) -> ()  [unwired: 5 in, 1 out]
                  }
                  frame "sound" {
                    w1088 = 0.0 ("element")
                    n701 = local read "water # 2.2R"() -> (w1089:dbl)
                    n702 = local read "water # 2.1L"() -> (w1090:dbl)
                    n703 = local read "current sound"() -> (w1084:dbl)
                    n704 = local read "trial #"() -> (w1085:dbl)
                    n705 = local read "lick  #  2.2R"() -> (w1092:dbl)
                    n706 = local read "lick  #  2.1L"() -> (w1093:dbl)
                    n707 = local read "ITI (s)"() -> (w1083:dbl)
                    n708 = local read "mistake # 2.2R"() -> (w1086:dbl)
                    n709 = local read "time (s)"() -> (w1094:dbl)
                    n710 = Increment(x=w1092) -> (x+1=w1091:dbl)
                    n711 = local read "mistake # 2.1L"() -> (w1087:dbl)
                    n712 = local write "lick  #  2.2R"(w1091) -> ()
                    n713 = local read "Mouse path 2"() -> (w1097:path)
                    n714 = Build Array(w1094, w1093, w1091, w1090, w1089, w1088, w1088, w1085, w1084, w1083, w1088, w1087, w1086) -> (w1095:dbl[])
                    n715 = call-poly <vilib>:"Write To Spreadsheet File.vi"("append to file? (new file:F)"=TRUE, "1D data"=w1095, "file path (dialog if empty)"=w1097) -> ()  [unwired: 5 in, 1 out]
                  }
                }
              }
            }
          }
          frame 3 {
            n716 = case shown="True" w1150 {
              frame False {
              }
              frame True {
                n717 = local read "state 2.1"() -> (w1202:enum16{"waiting", "sound", "ITI"})
                n718 = case shown="\"sound\"" w1202 {
                  frame "waiting", Default {
                    w1211 = 0.0 ("element")
                    n719 = local read "water # 2.1L"() -> (w1214:dbl)
                    n720 = local read "lick  #  2.2R"() -> (w1215:dbl)
                    n721 = local read "lick  #  2.1L"() -> (w1217:dbl)
                    n722 = local read "water # 2.2R"() -> (w1212:dbl)
                    n723 = local write "state 2.2"(enum16{"waiting", "sound", "ITI"}."ITI") -> ()
                    n724 = local write "state 2.1"(enum16{"waiting", "sound", "ITI"}."ITI") -> ()
                    n725 = local read "mistake # 2.2R"() -> (w1209:dbl)
                    n726 = local read "mistake # 2.1L"() -> (w1210:dbl)
                    n727 = Increment(x=w1214) -> (x+1=w1213:dbl)
                    n728 = Increment(x=w1217) -> (x+1=w1216:dbl)
                    n729 = local read "time (s)"() -> (w1208:dbl)
                    n730 = local read "current sound"() -> (w1204:dbl)
                    n731 = local read "free water 2.1"() -> (w1207:bool)
                    n732 = local write "water # 2.1L"(w1213) -> ()
                    n733 = local read "ITI (s)"() -> (w1203:dbl)
                    n734 = local read "trial #"() -> (w1205:dbl)
                    n735 = local write "lick  #  2.1L"(w1216) -> ()
                    n736 = local write "last water 2.1L"(w1208) -> ()
                    n737 = case shown="False" w1207 {
                      frame False {
                        n738 = local read "water dur (ms) 2.1"() -> (w1224:dbl)
                        n739 = local read "water port 2.1"() -> (w1223:tag)
                        n740 = call "_digital_on_duration_off.vi"("duration (ms)"=w1224, "digital port"=w1223) -> ()  [unwired: 10 in]
                      }
                      frame True {
                      }
                    }
                    n741 = Build Array(w1208, w1216, w1215, w1213, w1212, 1.0 ("element"), w1211, w1205, w1204, w1203, w1211, w1210, w1209) -> (w1218:dbl[])
                    n742 = local read "Mouse path 2"() -> (w1219:path)
                    n743 = call-poly <vilib>:"Write To Spreadsheet File.vi"("append to file? (new file:F)"=TRUE, "1D data"=w1218, "file path (dialog if empty)"=w1219) -> ()  [unwired: 5 in, 1 out]
                  }
                  frame "ITI" {
                    w1230 = 0.0 ("element")
                    n744 = local read "lick  #  2.2R"() -> (w1233:dbl)
                    n745 = local read "water # 2.2R"() -> (w1231:dbl)
                    n746 = local read "water # 2.1L"() -> (w1232:dbl)
                    n747 = local read "lick  #  2.1L"() -> (w1235:dbl)
                    n748 = local read "current sound"() -> (w1226:dbl)
                    n749 = local read "mistake # 2.2R"() -> (w1228:dbl)
                    n750 = local read "trial #"() -> (w1227:dbl)
                    n751 = local read "ITI (s)"() -> (w1225:dbl)
                    n752 = local read "mistake # 2.1L"() -> (w1229:dbl)
                    n753 = local read "time (s)"() -> (w1236:dbl)
                    n754 = Increment(x=w1235) -> (x+1=w1234:dbl)
                    n755 = local write "lick  #  2.1L"(w1234) -> ()
                    n756 = local read "Mouse path 2"() -> (w1238:path)
                    n757 = Build Array(w1236, w1234, w1233, w1232, w1231, w1230, w1230, w1227, w1226, w1225, w1230, w1229, w1228) -> (w1237:dbl[])
                    n758 = call-poly <vilib>:"Write To Spreadsheet File.vi"("append to file? (new file:F)"=TRUE, "1D data"=w1237, "file path (dialog if empty)"=w1238) -> ()  [unwired: 5 in, 1 out]
                  }
                  frame "sound" {
                    w1245 = 0.0 ("element")
                    n759 = local read "current sound"() -> (w1241:dbl)
                    n760 = local read "water # 2.2R"() -> (w1246:dbl)
                    n761 = local read "water # 2.1L"() -> (w1247:dbl)
                    n762 = local read "lick  #  2.1L"() -> (w1250:dbl)
                    n763 = local read "trial #"() -> (w1242:dbl)
                    n764 = local read "ITI (s)"() -> (w1240:dbl)
                    n765 = local read "mistake # 2.2R"() -> (w1243:dbl)
                    n766 = local read "lick  #  2.2R"() -> (w1248:dbl)
                    n767 = local read "mistake # 2.1L"() -> (w1244:dbl)
                    n768 = local read "time (s)"() -> (w1251:dbl)
                    n769 = Increment(x=w1250) -> (x+1=w1249:dbl)
                    n770 = local read "Mouse path 2"() -> (w1253:path)
                    n771 = local write "lick  #  2.1L"(w1249) -> ()
                    n772 = Build Array(w1251, w1249, w1248, w1247, w1246, w1245, w1245, w1242, w1241, w1240, w1245, w1244, w1243) -> (w1252:dbl[])
                    n773 = call-poly <vilib>:"Write To Spreadsheet File.vi"("append to file? (new file:F)"=TRUE, "1D data"=w1252, "file path (dialog if empty)"=w1253) -> ()  [unwired: 5 in, 1 out]
                  }
                }
              }
            }
            n774 = case shown="True" w1149 {
              frame False {
              }
              frame True {
                n775 = local read "state 2.1"() -> (w1151:enum16{"waiting", "sound", "ITI"})
                n776 = case shown="\"waiting\", Default" w1151 {
                  frame "waiting", Default {
                    w1160 = 0.0 ("element")
                    n777 = local read "LED 2"() -> (w1156:tag)
                    n778 = local write "LED 2 (i)"(1.0 ("LED 2 (i)")) -> ()
                    n779 = local write "state 2.2"(enum16{"waiting", "sound", "ITI"}."ITI") -> ()
                    n780 = local write "state 2.1"(enum16{"waiting", "sound", "ITI"}."ITI") -> ()
                    n781 = local read "water # 2.2R"() -> (w1161:dbl)
                    n782 = local read "mistake # 2.2R"() -> (w1157:dbl)
                    n783 = local read "current sound"() -> (w1153:dbl)
                    n784 = local read "water # 2.1L"() -> (w1162:dbl)
                    n785 = local read "lick  #  2.2R"() -> (w1164:dbl)
                    n786 = local read "mistake # 2.1L"() -> (w1159:dbl)
                    n787 = call "_digital_on.vi"("digital port"=w1156) -> ()  [unwired: 11 in]
                    n788 = local read "trial #"() -> (w1154:dbl)
                    n789 = local read "ITI (s)"() -> (w1152:dbl)
                    n790 = local read "lick  #  2.1L"() -> (w1165:dbl)
                    n791 = local read "time (s)"() -> (w1166:dbl)
                    n792 = Increment(x=w1164) -> (x+1=w1163:dbl)
                    n793 = Increment(x=w1159) -> (x+1=w1158:dbl)
                    n794 = local write "mistake # 2.1L"(w1158) -> ()
                    n795 = local write "lick  #  2.2R"(w1163) -> ()
                    n796 = local read "Mouse path 2"() -> (w1169:path)
                    n797 = Build Array(w1166, w1165, w1163, w1162, w1161, w1160, w1160, w1154, w1153, w1152, w1160, w1158, w1157) -> (w1167:dbl[])
                    n798 = call-poly <vilib>:"Write To Spreadsheet File.vi"("append to file? (new file:F)"=TRUE, "1D data"=w1167, "file path (dialog if empty)"=w1169) -> ()  [unwired: 5 in, 1 out]
                  }
                  frame "ITI" {
                    w1177 = 0.0 ("element")
                    n799 = local read "water # 2.2R"() -> (w1178:dbl)
                    n800 = local read "water # 2.1L"() -> (w1179:dbl)
                    n801 = local read "lick  #  2.2R"() -> (w1181:dbl)
                    n802 = local read "current sound"() -> (w1173:dbl)
                    n803 = local read "mistake # 2.2R"() -> (w1175:dbl)
                    n804 = local read "mistake # 2.1L"() -> (w1176:dbl)
                    n805 = local read "lick  #  2.1L"() -> (w1182:dbl)
                    n806 = local read "trial #"() -> (w1174:dbl)
                    n807 = local read "ITI (s)"() -> (w1172:dbl)
                    n808 = local read "time (s)"() -> (w1183:dbl)
                    n809 = Increment(x=w1181) -> (x+1=w1180:dbl)
                    n810 = local write "lick  #  2.2R"(w1180) -> ()
                    n811 = local read "Mouse path 2"() -> (w1185:path)
                    n812 = Build Array(w1183, w1182, w1180, w1179, w1178, w1177, w1177, w1174, w1173, w1172, w1177, w1176, w1175) -> (w1184:dbl[])
                    n813 = call-poly <vilib>:"Write To Spreadsheet File.vi"("append to file? (new file:F)"=TRUE, "1D data"=w1184, "file path (dialog if empty)"=w1185) -> ()  [unwired: 5 in, 1 out]
                  }
                  frame "sound" {
                    w1192 = 0.0 ("element")
                    n814 = local read "water # 2.2R"() -> (w1193:dbl)
                    n815 = local read "current sound"() -> (w1188:dbl)
                    n816 = local read "water # 2.1L"() -> (w1194:dbl)
                    n817 = local read "lick  #  2.2R"() -> (w1196:dbl)
                    n818 = local read "trial #"() -> (w1189:dbl)
                    n819 = local read "ITI (s)"() -> (w1187:dbl)
                    n820 = local read "lick  #  2.1L"() -> (w1197:dbl)
                    n821 = local read "mistake # 2.2R"() -> (w1190:dbl)
                    n822 = local read "mistake # 2.1L"() -> (w1191:dbl)
                    n823 = Increment(x=w1196) -> (x+1=w1195:dbl)
                    n824 = local read "time (s)"() -> (w1198:dbl)
                    n825 = local write "lick  #  2.2R"(w1195) -> ()
                    n826 = local read "Mouse path 2"() -> (w1200:path)
                    n827 = Build Array(w1198, w1197, w1195, w1194, w1193, w1192, w1192, w1189, w1188, w1187, w1192, w1191, w1190) -> (w1199:dbl[])
                    n828 = call-poly <vilib>:"Write To Spreadsheet File.vi"("append to file? (new file:F)"=TRUE, "1D data"=w1199, "file path (dialog if empty)"=w1200) -> ()  [unwired: 5 in, 1 out]
                  }
                }
              }
            }
          }
          frame 4 {
            n829 = case shown="True" w1256 {
              frame False {
              }
              frame True {
                n830 = local read "state 2.2"() -> (w1310:enum16{"waiting", "sound", "ITI"})
                n831 = case shown="\"ITI\"" w1310 {
                  frame "waiting", Default {
                    w1319 = 0.0 ("element")
                    n832 = local read "LED 2"() -> (w1315:tag)
                    n833 = local write "LED 2 (i)"(1.0 ("LED 2 (i)")) -> ()
                    n834 = local read "lick  #  2.2R"() -> (w1322:dbl)
                    n835 = call "_digital_on.vi"("digital port"=w1315) -> ()  [unwired: 11 in]
                    n836 = local read "lick  #  2.1L"() -> (w1324:dbl)
                    n837 = local read "current sound"() -> (w1312:dbl)
                    n838 = local read "water # 2.2R"() -> (w1320:dbl)
                    n839 = local read "water # 2.1L"() -> (w1321:dbl)
                    n840 = local read "trial #"() -> (w1313:dbl)
                    n841 = local read "mistake # 2.2R"() -> (w1317:dbl)
                    n842 = local read "mistake # 2.1L"() -> (w1318:dbl)
                    n843 = local read "ITI (s)"() -> (w1311:dbl)
                    n844 = local read "time (s)"() -> (w1325:dbl)
                    n845 = Increment(x=w1324) -> (x+1=w1323:dbl)
                    n846 = local write "lick  #  2.1L"(w1323) -> ()
                    n847 = local read "Mouse path 2"() -> (w1327:path)
                    n848 = Increment(x=w1317) -> (x+1=w1316:dbl)
                    n849 = local write "mistake # 2.2R"(w1316) -> ()
                    n850 = Build Array(w1325, w1323, w1322, w1321, w1320, w1319, w1319, w1313, w1312, w1311, w1319, w1318, w1316) -> (w1326:dbl[])
                    n851 = call-poly <vilib>:"Write To Spreadsheet File.vi"("append to file? (new file:F)"=TRUE, "1D data"=w1326, "file path (dialog if empty)"=w1327) -> ()  [unwired: 5 in, 1 out]
                    n852 = local write "state 2.2"(enum16{"waiting", "sound", "ITI"}."ITI") -> ()
                    n853 = local write "state 2.1"(enum16{"waiting", "sound", "ITI"}."ITI") -> ()
                  }
                  frame "sound" {
                    w1336 = 0.0 ("element")
                    n854 = local read "current sound"() -> (w1332:dbl)
                    n855 = local read "lick  #  2.2R"() -> (w1339:dbl)
                    n856 = local read "lick  #  2.1L"() -> (w1341:dbl)
                    n857 = local read "water # 2.2R"() -> (w1337:dbl)
                    n858 = local read "trial #"() -> (w1333:dbl)
                    n859 = local read "ITI (s)"() -> (w1331:dbl)
                    n860 = local read "water # 2.1L"() -> (w1338:dbl)
                    n861 = local read "mistake # 2.2R"() -> (w1334:dbl)
                    n862 = local read "time (s)"() -> (w1342:dbl)
                    n863 = local read "mistake # 2.1L"() -> (w1335:dbl)
                    n864 = Increment(x=w1341) -> (x+1=w1340:dbl)
                    n865 = local write "lick  #  2.1L"(w1340) -> ()
                    n866 = local read "Mouse path 2"() -> (w1344:path)
                    n867 = Build Array(w1342, w1340, w1339, w1338, w1337, w1336, w1336, w1333, w1332, w1331, w1336, w1335, w1334) -> (w1343:dbl[])
                    n868 = call-poly <vilib>:"Write To Spreadsheet File.vi"("append to file? (new file:F)"=TRUE, "1D data"=w1343, "file path (dialog if empty)"=w1344) -> ()  [unwired: 5 in, 1 out]
                  }
                  frame "ITI" {
                    w1351 = 0.0 ("element")
                    n869 = local read "water # 2.1L"() -> (w1353:dbl)
                    n870 = local read "water # 2.2R"() -> (w1352:dbl)
                    n871 = local read "current sound"() -> (w1347:dbl)
                    n872 = local read "lick  #  2.2R"() -> (w1354:dbl)
                    n873 = local read "lick  #  2.1L"() -> (w1356:dbl)
                    n874 = local read "trial #"() -> (w1348:dbl)
                    n875 = local read "ITI (s)"() -> (w1346:dbl)
                    n876 = local read "mistake # 2.2R"() -> (w1349:dbl)
                    n877 = local read "mistake # 2.1L"() -> (w1350:dbl)
                    n878 = local read "time (s)"() -> (w1357:dbl)
                    n879 = Increment(x=w1356) -> (x+1=w1355:dbl)
                    n880 = local write "lick  #  2.1L"(w1355) -> ()
                    n881 = local read "Mouse path 2"() -> (w1359:path)
                    n882 = Build Array(w1357, w1355, w1354, w1353, w1352, w1351, w1351, w1348, w1347, w1346, w1351, w1350, w1349) -> (w1358:dbl[])
                    n883 = call-poly <vilib>:"Write To Spreadsheet File.vi"("append to file? (new file:F)"=TRUE, "1D data"=w1358, "file path (dialog if empty)"=w1359) -> ()  [unwired: 5 in, 1 out]
                  }
                }
              }
            }
            n884 = case shown="True" w1255 {
              frame False {
              }
              frame True {
                n885 = local read "state 2.2"() -> (w1257:enum16{"waiting", "sound", "ITI"})
                n886 = case shown="\"ITI\"" w1257 {
                  frame "waiting", Default {
                    w1265 = 0.0 ("element")
                    n887 = local read "water # 2.2R"() -> (w1267:dbl)
                    n888 = local read "lick  #  2.2R"() -> (w1270:dbl)
                    n889 = local read "water # 2.1L"() -> (w1268:dbl)
                    n890 = local read "lick  #  2.1L"() -> (w1271:dbl)
                    n891 = local read "current sound"() -> (w1259:dbl)
                    n892 = local read "trial #"() -> (w1260:dbl)
                    n893 = local read "time (s)"() -> (w1272:dbl)
                    n894 = local read "ITI (s)"() -> (w1258:dbl)
                    n895 = local read "mistake # 2.2R"() -> (w1263:dbl)
                    n896 = local read "mistake # 2.1L"() -> (w1264:dbl)
                    n897 = Increment(x=w1270) -> (x+1=w1269:dbl)
                    n898 = Increment(x=w1267) -> (x+1=w1266:dbl)
                    n899 = local write "state 2.1"(enum16{"waiting", "sound", "ITI"}."ITI") -> ()
                    n900 = local write "state 2.2"(enum16{"waiting", "sound", "ITI"}."ITI") -> ()
                    n901 = local write "water # 2.2R"(w1266) -> ()
                    n902 = local write "lick  #  2.2R"(w1269) -> ()
                    n903 = local read "Mouse path 2"() -> (w1274:path)
                    n904 = Build Array(w1272, w1271, w1269, w1268, w1266, 1.0 ("element"), w1265, w1260, w1259, w1258, w1265, w1264, w1263) -> (w1273:dbl[])
                    n905 = call-poly <vilib>:"Write To Spreadsheet File.vi"("append to file? (new file:F)"=TRUE, "1D data"=w1273, "file path (dialog if empty)"=w1274) -> ()  [unwired: 5 in, 1 out]
                    n906 = local read "free water 2.2"() -> (w1262:bool)
                    n907 = case shown="False" w1262 {
                      frame False {
                        n908 = local read "water dur (ms) 2.2"() -> (w1279:dbl)
                        n909 = local read "water port 2.2"() -> (w1278:tag)
                        n910 = call "_digital_on_duration_off.vi"("duration (ms)"=w1279, "digital port"=w1278) -> ()  [unwired: 10 in]
                      }
                      frame True {
                      }
                    }
                  }
                  frame "sound" {
                    w1285 = 0.0 ("element")
                    n911 = local read "current sound"() -> (w1281:dbl)
                    n912 = local read "water # 2.1L"() -> (w1287:dbl)
                    n913 = local read "water # 2.2R"() -> (w1286:dbl)
                    n914 = local read "lick  #  2.2R"() -> (w1289:dbl)
                    n915 = local read "lick  #  2.1L"() -> (w1290:dbl)
                    n916 = local read "trial #"() -> (w1282:dbl)
                    n917 = local read "ITI (s)"() -> (w1280:dbl)
                    n918 = local read "mistake # 2.2R"() -> (w1283:dbl)
                    n919 = local read "time (s)"() -> (w1291:dbl)
                    n920 = local read "mistake # 2.1L"() -> (w1284:dbl)
                    n921 = Increment(x=w1289) -> (x+1=w1288:dbl)
                    n922 = local write "lick  #  2.2R"(w1288) -> ()
                    n923 = local read "Mouse path 2"() -> (w1294:path)
                    n924 = Build Array(w1291, w1290, w1288, w1287, w1286, w1285, w1285, w1282, w1281, w1280, w1285, w1284, w1283) -> (w1292:dbl[])
                    n925 = call-poly <vilib>:"Write To Spreadsheet File.vi"("append to file? (new file:F)"=TRUE, "1D data"=w1292, "file path (dialog if empty)"=w1294) -> ()  [unwired: 5 in, 1 out]
                  }
                  frame "ITI" {
                    w1300 = 0.0 ("element")
                    n926 = local read "water # 2.2R"() -> (w1301:dbl)
                    n927 = local read "water # 2.1L"() -> (w1302:dbl)
                    n928 = local read "current sound"() -> (w1296:dbl)
                    n929 = local read "lick  #  2.2R"() -> (w1304:dbl)
                    n930 = local read "trial #"() -> (w1297:dbl)
                    n931 = local read "lick  #  2.1L"() -> (w1305:dbl)
                    n932 = local read "ITI (s)"() -> (w1295:dbl)
                    n933 = local read "time (s)"() -> (w1306:dbl)
                    n934 = Increment(x=w1304) -> (x+1=w1303:dbl)
                    n935 = local write "lick  #  2.2R"(w1303) -> ()
                    n936 = local read "mistake # 2.2R"() -> (w1298:dbl)
                    n937 = local read "mistake # 2.1L"() -> (w1299:dbl)
                    n938 = local read "Mouse path 2"() -> (w1307:path)
                    n939 = Build Array(w1306, w1305, w1303, w1302, w1301, w1300, w1300, w1297, w1296, w1295, w1300, w1299, w1298) -> (w1308:dbl[])
                    n940 = call-poly <vilib>:"Write To Spreadsheet File.vi"("append to file? (new file:F)"=TRUE, "1D data"=w1308, "file path (dialog if empty)"=w1307) -> ()  [unwired: 5 in, 1 out]
                  }
                }
              }
            }
          }
        }
        n941 = case shown="4" w43 {
          tunnel: w32 -> [_ w89 w196 w302 w408]
          tunnel: w33 -> [_ w90 w195 w301 w407]
          frame 0, Default {
          }
          frame 1 {
            n942 = case shown="True" w90 {
              frame False {
              }
              frame True {
                n943 = local read "state 4.1"() -> (w144:enum16{"waiting", "sound", "ITI"})
                n944 = case shown="\"ITI\"" w144 {
                  frame "waiting", Default {
                    w153 = 0.0 ("element")
                    n945 = local read "water # 4.1L"() -> (w155:dbl)
                    n946 = local read "water # 4.2R"() -> (w154:dbl)
                    n947 = local read "lick # 4.2R"() -> (w157:dbl)
                    n948 = local read "lick # 4.1L"() -> (w158:dbl)
                    n949 = local read "current sound"() -> (w146:dbl)
                    n950 = local write "state 4.2"(enum16{"waiting", "sound", "ITI"}."ITI") -> ()
                    n951 = local read "trial #"() -> (w147:dbl)
                    n952 = local read "mistake # 4.2R"() -> (w150:dbl)
                    n953 = local write "state 4.1"(enum16{"waiting", "sound", "ITI"}."ITI") -> ()
                    n954 = local read "mistake # 4.1L"() -> (w152:dbl)
                    n955 = local read "ITI (s)"() -> (w145:dbl)
                    n956 = Increment(x=w157) -> (x+1=w156:dbl)
                    n957 = local read "time (s)"() -> (w159:dbl)
                    n958 = local write "lick # 4.2R"(w156) -> ()
                    n959 = Increment(x=w152) -> (x+1=w151:dbl)
                    n960 = local read "Mouse path 4"() -> (w161:path)
                    n961 = local write "mistake # 4.1L"(w151) -> ()
                    n962 = Build Array(w159, w158, w156, w155, w154, w153, w153, w147, w146, w145, w153, w151, w150) -> (w160:dbl[])
                    n963 = call-poly <vilib>:"Write To Spreadsheet File.vi"("append to file? (new file:F)"=TRUE, "1D data"=w160, "file path (dialog if empty)"=w161) -> ()  [unwired: 5 in, 1 out]
                    n964 = local read "LED 4"() -> (w148:tag)
                    n965 = local write "LED 4 (i)"(1.0 ("LED 4 (i)")) -> ()
                    n966 = call "_digital_on.vi"("digital port"=w148) -> ()  [unwired: 11 in]
                  }
                  frame "sound" {
                    w170 = 0.0 ("element")
                    n967 = local read "water # 4.2R"() -> (w171:dbl)
                    n968 = local read "lick # 4.2R"() -> (w174:dbl)
                    n969 = local read "water # 4.1L"() -> (w172:dbl)
                    n970 = local read "lick # 4.1L"() -> (w175:dbl)
                    n971 = local read "current sound"() -> (w166:dbl)
                    n972 = local read "time (s)"() -> (w176:dbl)
                    n973 = Increment(x=w174) -> (x+1=w173:dbl)
                    n974 = local read "trial #"() -> (w167:dbl)
                    n975 = local read "ITI (s)"() -> (w165:dbl)
                    n976 = local write "lick # 4.2R"(w173) -> ()
                    n977 = local read "mistake # 4.2R"() -> (w168:dbl)
                    n978 = local read "Mouse path 4"() -> (w178:path)
                    n979 = local read "mistake # 4.1L"() -> (w169:dbl)
                    n980 = Build Array(w176, w175, w173, w172, w171, w170, w170, w167, w166, w165, w170, w169, w168) -> (w177:dbl[])
                    n981 = call-poly <vilib>:"Write To Spreadsheet File.vi"("append to file? (new file:F)"=TRUE, "1D data"=w177, "file path (dialog if empty)"=w178) -> ()  [unwired: 5 in, 1 out]
                  }
                  frame "ITI" {
                    w185 = 0.0 ("element")
                    n982 = local read "current sound"() -> (w181:dbl)
                    n983 = local read "water # 4.2R"() -> (w186:dbl)
                    n984 = local read "water # 4.1L"() -> (w187:dbl)
                    n985 = local read "trial #"() -> (w182:dbl)
                    n986 = local read "lick # 4.2R"() -> (w189:dbl)
                    n987 = local read "ITI (s)"() -> (w180:dbl)
                    n988 = local read "lick # 4.1L"() -> (w190:dbl)
                    n989 = local read "mistake # 4.2R"() -> (w183:dbl)
                    n990 = local read "time (s)"() -> (w191:dbl)
                    n991 = Increment(x=w189) -> (x+1=w188:dbl)
                    n992 = local read "mistake # 4.1L"() -> (w184:dbl)
                    n993 = local write "lick # 4.2R"(w188) -> ()
                    n994 = local read "Mouse path 4"() -> (w193:path)
                    n995 = Build Array(w191, w190, w188, w187, w186, w185, w185, w182, w181, w180, w185, w184, w183) -> (w192:dbl[])
                    n996 = call-poly <vilib>:"Write To Spreadsheet File.vi"("append to file? (new file:F)"=TRUE, "1D data"=w192, "file path (dialog if empty)"=w193) -> ()  [unwired: 5 in, 1 out]
                  }
                }
              }
            }
            n997 = case shown="True" w89 {
              frame False {
              }
              frame True {
                n998 = local read "state 4.1"() -> (w91:enum16{"waiting", "sound", "ITI"})
                n999 = case shown="\"waiting\", Default" w91 {
                  frame "waiting", Default {
                    w99 = 0.0 ("element")
                    n1000 = local read "water # 4.1L"() -> (w102:dbl)
                    n1001 = local read "lick # 4.2R"() -> (w103:dbl)
                    n1002 = local read "lick # 4.1L"() -> (w105:dbl)
                    n1003 = local read "water # 4.2R"() -> (w100:dbl)
                    n1004 = local read "current sound"() -> (w93:dbl)
                    n1005 = local read "time (s)"() -> (w96:dbl)
                    n1006 = local read "trial #"() -> (w94:dbl)
                    n1007 = Increment(x=w102) -> (x+1=w101:dbl)
                    n1008 = Increment(x=w105) -> (x+1=w104:dbl)
                    n1009 = local write "state 4.2"(enum16{"waiting", "sound", "ITI"}."ITI") -> ()
                    n1010 = local write "state 4.1"(enum16{"waiting", "sound", "ITI"}."ITI") -> ()
                    n1011 = local read "ITI (s)"() -> (w92:dbl)
                    n1012 = local write "water # 4.1L"(w101) -> ()
                    n1013 = local read "mistake # 4.2R"() -> (w97:dbl)
                    n1014 = local read "mistake # 4.1L"() -> (w98:dbl)
                    n1015 = local write "last water 4.1L"(w96) -> ()
                    n1016 = local write "lick # 4.1L"(w104) -> ()
                    n1017 = local read "Mouse path 4"() -> (w107:path)
                    n1018 = Build Array(w96, w104, w103, w101, w100, 1.0 ("element"), w99, w94, w93, w92, w99, w98, w97) -> (w106:dbl[])
                    n1019 = local read "free water 4.1"() -> (w109:bool)
                    n1020 = call-poly <vilib>:"Write To Spreadsheet File.vi"("append to file? (new file:F)"=TRUE, "1D data"=w106, "file path (dialog if empty)"=w107) -> ()  [unwired: 5 in, 1 out]
                    n1021 = case shown="False" w109 {
                      frame False {
                        n1022 = call "_digital_on_duration_off.vi"("duration (ms)"="water dur (ms) 4.1", "digital port"="water port 4.1") -> ()  [unwired: 10 in]
                      }
                      frame True {
                      }
                    }
                  }
                  frame "sound" {
                    w119 = 0.0 ("element")
                    n1023 = local read "current sound"() -> (w115:dbl)
                    n1024 = local read "water # 4.2R"() -> (w120:dbl)
                    n1025 = local read "water # 4.1L"() -> (w121:dbl)
                    n1026 = local read "trial #"() -> (w116:dbl)
                    n1027 = local read "lick # 4.2R"() -> (w122:dbl)
                    n1028 = local read "ITI (s)"() -> (w114:dbl)
                    n1029 = local read "lick # 4.1L"() -> (w124:dbl)
                    n1030 = local read "mistake # 4.2R"() -> (w117:dbl)
                    n1031 = local read "time (s)"() -> (w125:dbl)
                    n1032 = local read "mistake # 4.1L"() -> (w118:dbl)
                    n1033 = Increment(x=w124) -> (x+1=w123:dbl)
                    n1034 = local write "lick # 4.1L"(w123) -> ()
                    n1035 = local read "Mouse path 4"() -> (w127:path)
                    n1036 = Build Array(w125, w123, w122, w121, w120, w119, w119, w116, w115, w114, w119, w118, w117) -> (w126:dbl[])
                    n1037 = call-poly <vilib>:"Write To Spreadsheet File.vi"("append to file? (new file:F)"=TRUE, "1D data"=w126, "file path (dialog if empty)"=w127) -> ()  [unwired: 5 in, 1 out]
                  }
                  frame "ITI" {
                    w134 = 0.0 ("element")
                    n1038 = local read "current sound"() -> (w130:dbl)
                    n1039 = local read "water # 4.2R"() -> (w135:dbl)
                    n1040 = local read "water # 4.1L"() -> (w136:dbl)
                    n1041 = local read "trial #"() -> (w131:dbl)
                    n1042 = local read "mistake # 4.2R"() -> (w132:dbl)
                    n1043 = local read "lick # 4.2R"() -> (w137:dbl)
                    n1044 = local read "mistake # 4.1L"() -> (w133:dbl)
                    n1045 = local read "ITI (s)"() -> (w129:dbl)
                    n1046 = local read "lick # 4.1L"() -> (w139:dbl)
                    n1047 = local read "time (s)"() -> (w140:dbl)
                    n1048 = Increment(x=w139) -> (x+1=w138:dbl)
                    n1049 = local write "lick # 4.1L"(w138) -> ()
                    n1050 = local read "Mouse path 4"() -> (w142:path)
                    n1051 = Build Array(w140, w138, w137, w136, w135, w134, w134, w131, w130, w129, w134, w133, w132) -> (w141:dbl[])
                    n1052 = call-poly <vilib>:"Write To Spreadsheet File.vi"("append to file? (new file:F)"=TRUE, "1D data"=w141, "file path (dialog if empty)"=w142) -> ()  [unwired: 5 in, 1 out]
                  }
                }
              }
            }
          }
          frame 2 {
            n1053 = case shown="True" w195 {
              frame False {
              }
              frame True {
                n1054 = local read "state 4.2"() -> (w248:enum16{"waiting", "sound", "ITI"})
                n1055 = case shown="\"ITI\"" w248 {
                  frame "waiting", Default {
                    w256 = 0.0 ("element")
                    n1056 = local read "water # 4.2R"() -> (w258:dbl)
                    n1057 = local read "current sound"() -> (w250:dbl)
                    n1058 = local read "mistake # 4.2R"() -> (w254:dbl)
                    n1059 = local read "mistake # 4.1L"() -> (w255:dbl)
                    n1060 = local read "trial #"() -> (w251:dbl)
                    n1061 = local read "ITI (s)"() -> (w249:dbl)
                    n1062 = local read "water # 4.1L"() -> (w259:dbl)
                    n1063 = local read "lick # 4.2R"() -> (w261:dbl)
                    n1064 = local write "state 4.2"(enum16{"waiting", "sound", "ITI"}."ITI") -> ()
                    n1065 = local write "state 4.1"(enum16{"waiting", "sound", "ITI"}."ITI") -> ()
                    n1066 = local read "lick # 4.1L"() -> (w262:dbl)
                    n1067 = Increment(x=w258) -> (x+1=w257:dbl)
                    n1068 = local read "time (s)"() -> (w253:dbl)
                    n1069 = local write "water # 4.2R"(w257) -> ()
                    n1070 = Increment(x=w261) -> (x+1=w260:dbl)
                    n1071 = local write "last water 4.2R"(w253) -> ()
                    n1072 = local read "free water 4.2"() -> (w266:bool)
                    n1073 = local write "lick # 4.2R"(w260) -> ()
                    n1074 = Build Array(w253, w262, w260, w259, w257, 1.0 ("element"), w256, w251, w250, w249, w256, w255, w254) -> (w263:dbl[])
                    n1075 = local read "Mouse path 4"() -> (w264:path)
                    n1076 = case shown="False" w266 {
                      frame False {
                        n1077 = call "_digital_on_duration_off.vi"("duration (ms)"="water dur (ms) 4.2", "digital port"="water port 4.2") -> ()  [unwired: 10 in]
                      }
                      frame True {
                      }
                    }
                    n1078 = call-poly <vilib>:"Write To Spreadsheet File.vi"("append to file? (new file:F)"=TRUE, "1D data"=w263, "file path (dialog if empty)"=w264) -> ()  [unwired: 5 in, 1 out]
                  }
                  frame "sound" {
                    w276 = 0.0 ("element")
                    n1079 = local read "current sound"() -> (w272:dbl)
                    n1080 = local read "trial #"() -> (w273:dbl)
                    n1081 = local read "water # 4.1L"() -> (w278:dbl)
                    n1082 = local read "water # 4.2R"() -> (w277:dbl)
                    n1083 = local read "lick # 4.2R"() -> (w280:dbl)
                    n1084 = local read "ITI (s)"() -> (w271:dbl)
                    n1085 = local read "lick # 4.1L"() -> (w281:dbl)
                    n1086 = local read "time (s)"() -> (w282:dbl)
                    n1087 = Increment(x=w280) -> (x+1=w279:dbl)
                    n1088 = local read "mistake # 4.1L"() -> (w275:dbl)
                    n1089 = local read "mistake # 4.2R"() -> (w274:dbl)
                    n1090 = local write "lick # 4.2R"(w279) -> ()
                    n1091 = Build Array(w282, w281, w279, w278, w277, w276, w276, w273, w272, w271, w276, w275, w274) -> (w283:dbl[])
                    n1092 = local read "Mouse path 4"() -> (w284:path)
                    n1093 = call-poly <vilib>:"Write To Spreadsheet File.vi"("append to file? (new file:F)"=TRUE, "1D data"=w283, "file path (dialog if empty)"=w284) -> ()  [unwired: 5 in, 1 out]
                  }
                  frame "ITI" {
                    w291 = 0.0 ("element")
                    n1094 = local read "water # 4.2R"() -> (w292:dbl)
                    n1095 = local read "water # 4.1L"() -> (w293:dbl)
                    n1096 = local read "current sound"() -> (w287:dbl)
                    n1097 = local read "lick # 4.2R"() -> (w295:dbl)
                    n1098 = local read "trial #"() -> (w288:dbl)
                    n1099 = local read "lick # 4.1L"() -> (w296:dbl)
                    n1100 = local read "ITI (s)"() -> (w286:dbl)
                    n1101 = local read "mistake # 4.2R"() -> (w289:dbl)
                    n1102 = Increment(x=w295) -> (x+1=w294:dbl)
                    n1103 = local read "mistake # 4.1L"() -> (w290:dbl)
                    n1104 = local read "time (s)"() -> (w297:dbl)
                    n1105 = local write "lick # 4.2R"(w294) -> ()
                    n1106 = Build Array(w297, w296, w294, w293, w292, w291, w291, w288, w287, w286, w291, w290, w289) -> (w298:dbl[])
                    n1107 = local read "Mouse path 4"() -> (w299:path)
                    n1108 = call-poly <vilib>:"Write To Spreadsheet File.vi"("append to file? (new file:F)"=TRUE, "1D data"=w298, "file path (dialog if empty)"=w299) -> ()  [unwired: 5 in, 1 out]
                  }
                }
              }
            }
            n1109 = case shown="True" w196 {
              frame False {
              }
              frame True {
                n1110 = local read "state 4.2"() -> (w197:enum16{"waiting", "sound", "ITI"})
                n1111 = case shown="\"ITI\"" w197 {
                  frame "waiting", Default {
                    w206 = 0.0 ("element")
                    n1112 = local read "lick # 4.2R"() -> (w209:dbl)
                    n1113 = local read "current sound"() -> (w199:dbl)
                    n1114 = local read "ITI (s)"() -> (w198:dbl)
                    n1115 = local read "lick # 4.1L"() -> (w211:dbl)
                    n1116 = local read "trial #"() -> (w200:dbl)
                    n1117 = local read "mistake # 4.2R"() -> (w204:dbl)
                    n1118 = local read "water # 4.1L"() -> (w208:dbl)
                    n1119 = local read "water # 4.2R"() -> (w207:dbl)
                    n1120 = local read "time (s)"() -> (w212:dbl)
                    n1121 = local write "state 4.2"(enum16{"waiting", "sound", "ITI"}."ITI") -> ()
                    n1122 = local write "state 4.1"(enum16{"waiting", "sound", "ITI"}."ITI") -> ()
                    n1123 = local read "mistake # 4.1L"() -> (w205:dbl)
                    n1124 = Increment(x=w211) -> (x+1=w210:dbl)
                    n1125 = Increment(x=w204) -> (x+1=w203:dbl)
                    n1126 = local write "lick # 4.1L"(w210) -> ()
                    n1127 = local write "mistake # 4.2R"(w203) -> ()
                    n1128 = Build Array(w212, w210, w209, w208, w207, w206, w206, w200, w199, w198, w206, w205, w203) -> (w213:dbl[])
                    n1129 = local read "Mouse path 4"() -> (w214:path)
                    n1130 = local write "LED 4 (i)"(1.0 ("LED 4 (i)")) -> ()
                    n1131 = call-poly <vilib>:"Write To Spreadsheet File.vi"("append to file? (new file:F)"=TRUE, "1D data"=w213, "file path (dialog if empty)"=w214) -> ()  [unwired: 5 in, 1 out]
                    n1132 = call "_digital_on.vi"("digital port"="LED 4") -> ()  [unwired: 11 in]
                  }
                  frame "sound" {
                    w223 = 0.0 ("element")
                    n1133 = local read "current sound"() -> (w219:dbl)
                    n1134 = local read "water # 4.2R"() -> (w224:dbl)
                    n1135 = local read "water # 4.1L"() -> (w225:dbl)
                    n1136 = local read "lick # 4.2R"() -> (w226:dbl)
                    n1137 = local read "trial #"() -> (w220:dbl)
                    n1138 = local read "lick # 4.1L"() -> (w228:dbl)
                    n1139 = local read "ITI (s)"() -> (w218:dbl)
                    n1140 = local read "mistake # 4.2R"() -> (w221:dbl)
                    n1141 = local read "time (s)"() -> (w229:dbl)
                    n1142 = local read "mistake # 4.1L"() -> (w222:dbl)
                    n1143 = Increment(x=w228) -> (x+1=w227:dbl)
                    n1144 = local write "lick # 4.1L"(w227) -> ()
                    n1145 = Build Array(w229, w227, w226, w225, w224, w223, w223, w220, w219, w218, w223, w222, w221) -> (w230:dbl[])
                    n1146 = local read "Mouse path 4"() -> (w231:path)
                    n1147 = call-poly <vilib>:"Write To Spreadsheet File.vi"("append to file? (new file:F)"=TRUE, "1D data"=w230, "file path (dialog if empty)"=w231) -> ()  [unwired: 5 in, 1 out]
                  }
                  frame "ITI" {
                    w238 = 0.0 ("element")
                    n1148 = local read "current sound"() -> (w234:dbl)
                    n1149 = local read "water # 4.1L"() -> (w240:dbl)
                    n1150 = local read "water # 4.2R"() -> (w239:dbl)
                    n1151 = local read "lick # 4.2R"() -> (w241:dbl)
                    n1152 = local read "trial #"() -> (w235:dbl)
                    n1153 = local read "ITI (s)"() -> (w233:dbl)
                    n1154 = local read "lick # 4.1L"() -> (w243:dbl)
                    n1155 = local read "time (s)"() -> (w244:dbl)
                    n1156 = local read "mistake # 4.2R"() -> (w236:dbl)
                    n1157 = Increment(x=w243) -> (x+1=w242:dbl)
                    n1158 = local read "mistake # 4.1L"() -> (w237:dbl)
                    n1159 = local write "lick # 4.1L"(w242) -> ()
                    n1160 = local read "Mouse path 4"() -> (w246:path)
                    n1161 = Build Array(w244, w242, w241, w240, w239, w238, w238, w235, w234, w233, w238, w237, w236) -> (w245:dbl[])
                    n1162 = call-poly <vilib>:"Write To Spreadsheet File.vi"("append to file? (new file:F)"=TRUE, "1D data"=w245, "file path (dialog if empty)"=w246) -> ()  [unwired: 5 in, 1 out]
                  }
                }
              }
            }
          }
          frame 3 {
            n1163 = case shown="True" w301 {
              frame False {
              }
              frame True {
                n1164 = local read "state 4.1"() -> (w356:enum16{"waiting", "sound", "ITI"})
                n1165 = case shown="\"ITI\"" w356 {
                  frame "waiting", Default {
                    w365 = 0.0 ("element")
                    n1166 = local write "state 4.2"(enum16{"waiting", "sound", "ITI"}."ITI") -> ()
                    n1167 = local write "state 4.1"(enum16{"waiting", "sound", "ITI"}."ITI") -> ()
                    n1168 = local read "mistake # 4.1L"() -> (w364:dbl)
                    n1169 = local read "water # 4.2R"() -> (w366:dbl)
                    n1170 = local read "current sound"() -> (w358:dbl)
                    n1171 = local read "water # 4.1L"() -> (w367:dbl)
                    n1172 = local read "mistake # 4.2R"() -> (w362:dbl)
                    n1173 = local read "lick # 4.2R"() -> (w369:dbl)
                    n1174 = local read "trial #"() -> (w359:dbl)
                    n1175 = local read "ITI (s)"() -> (w357:dbl)
                    n1176 = local read "lick # 4.1L"() -> (w370:dbl)
                    n1177 = local read "time (s)"() -> (w371:dbl)
                    n1178 = Increment(x=w364) -> (x+1=w363:dbl)
                    n1179 = Increment(x=w369) -> (x+1=w368:dbl)
                    n1180 = local write "mistake # 4.1L"(w363) -> ()
                    n1181 = local write "lick # 4.2R"(w368) -> ()
                    n1182 = local read "Mouse path 4"() -> (w373:path)
                    n1183 = local read "LED 4"() -> (w360:tag)
                    n1184 = local write "LED 4 (i)"(1.0 ("LED 4 (i)")) -> ()
                    n1185 = Build Array(w371, w370, w368, w367, w366, w365, w365, w359, w358, w357, w365, w363, w362) -> (w372:dbl[])
                    n1186 = call "_digital_on.vi"("digital port"=w360) -> ()  [unwired: 11 in]
                    n1187 = call-poly <vilib>:"Write To Spreadsheet File.vi"("append to file? (new file:F)"=TRUE, "1D data"=w372, "file path (dialog if empty)"=w373) -> ()  [unwired: 5 in, 1 out]
                  }
                  frame "sound" {
                    w382 = 0.0 ("element")
                    n1188 = local read "lick # 4.2R"() -> (w386:dbl)
                    n1189 = local read "water # 4.1L"() -> (w384:dbl)
                    n1190 = local read "water # 4.2R"() -> (w383:dbl)
                    n1191 = local read "lick # 4.1L"() -> (w387:dbl)
                    n1192 = local read "current sound"() -> (w378:dbl)
                    n1193 = local read "time (s)"() -> (w388:dbl)
                    n1194 = local read "ITI (s)"() -> (w377:dbl)
                    n1195 = local read "trial #"() -> (w379:dbl)
                    n1196 = Increment(x=w386) -> (x+1=w385:dbl)
                    n1197 = local read "mistake # 4.2R"() -> (w380:dbl)
                    n1198 = local read "mistake # 4.1L"() -> (w381:dbl)
                    n1199 = local write "lick # 4.2R"(w385) -> ()
                    n1200 = Build Array(w388, w387, w385, w384, w383, w382, w382, w379, w378, w377, w382, w381, w380) -> (w389:dbl[])
                    n1201 = local read "Mouse path 4"() -> (w390:path)
                    n1202 = call-poly <vilib>:"Write To Spreadsheet File.vi"("append to file? (new file:F)"=TRUE, "1D data"=w389, "file path (dialog if empty)"=w390) -> ()  [unwired: 5 in, 1 out]
                  }
                  frame "ITI" {
                    w397 = 0.0 ("element")
                    n1203 = local read "water # 4.2R"() -> (w398:dbl)
                    n1204 = local read "water # 4.1L"() -> (w399:dbl)
                    n1205 = local read "current sound"() -> (w393:dbl)
                    n1206 = local read "lick # 4.2R"() -> (w401:dbl)
                    n1207 = local read "lick # 4.1L"() -> (w402:dbl)
                    n1208 = local read "trial #"() -> (w394:dbl)
                    n1209 = local read "time (s)"() -> (w403:dbl)
                    n1210 = local read "ITI (s)"() -> (w392:dbl)
                    n1211 = Increment(x=w401) -> (x+1=w400:dbl)
                    n1212 = local read "mistake # 4.1L"() -> (w396:dbl)
                    n1213 = local read "mistake # 4.2R"() -> (w395:dbl)
                    n1214 = local write "lick # 4.2R"(w400) -> ()
                    n1215 = local read "Mouse path 4"() -> (w405:path)
                    n1216 = Build Array(w403, w402, w400, w399, w398, w397, w397, w394, w393, w392, w397, w396, w395) -> (w404:dbl[])
                    n1217 = call-poly <vilib>:"Write To Spreadsheet File.vi"("append to file? (new file:F)"=TRUE, "1D data"=w404, "file path (dialog if empty)"=w405) -> ()  [unwired: 5 in, 1 out]
                  }
                }
              }
            }
            n1218 = case shown="True" w302 {
              frame False {
              }
              frame True {
                n1219 = local read "state 4.1"() -> (w303:enum16{"waiting", "sound", "ITI"})
                n1220 = case shown="\"waiting\", Default" w303 {
                  frame "waiting", Default {
                    w311 = 0.0 ("element")
                    n1221 = local read "water # 4.1L"() -> (w314:dbl)
                    n1222 = local write "state 4.2"(enum16{"waiting", "sound", "ITI"}."ITI") -> ()
                    n1223 = local read "water # 4.2R"() -> (w312:dbl)
                    n1224 = local write "state 4.1"(enum16{"waiting", "sound", "ITI"}."ITI") -> ()
                    n1225 = local read "lick # 4.2R"() -> (w315:dbl)
                    n1226 = local read "lick # 4.1L"() -> (w317:dbl)
                    n1227 = local read "time (s)"() -> (w308:dbl)
                    n1228 = local read "mistake # 4.2R"() -> (w309:dbl)
                    n1229 = local read "current sound"() -> (w305:dbl)
                    n1230 = Increment(x=w314) -> (x+1=w313:dbl)
                    n1231 = local read "mistake # 4.1L"() -> (w310:dbl)
                    n1232 = local read "trial #"() -> (w306:dbl)
                    n1233 = Increment(x=w317) -> (x+1=w316:dbl)
                    n1234 = local read "ITI (s)"() -> (w304:dbl)
                    n1235 = local write "water # 4.1L"(w313) -> ()
                    n1236 = local write "last water 4.1L"(w308) -> ()
                    n1237 = local read "free water 4.1"() -> (w323:bool)
                    n1238 = local write "lick # 4.1L"(w316) -> ()
                    n1239 = local read "Mouse path 4"() -> (w319:path)
                    n1240 = Build Array(w308, w316, w315, w313, w312, 1.0 ("element"), w311, w306, w305, w304, w311, w310, w309) -> (w318:dbl[])
                    n1241 = case shown="False" w323 {
                      frame False {
                        n1242 = local read "water dur (ms) 4.1"() -> (w324:dbl)
                        n1243 = local read "water port 4.1"() -> (w325:tag)
                        n1244 = call "_digital_on_duration_off.vi"("duration (ms)"=w324, "digital port"=w325) -> ()  [unwired: 10 in]
                      }
                      frame True {
                      }
                    }
                    n1245 = call-poly <vilib>:"Write To Spreadsheet File.vi"("append to file? (new file:F)"=TRUE, "1D data"=w318, "file path (dialog if empty)"=w319) -> ()  [unwired: 5 in, 1 out]
                  }
                  frame "sound" {
                    w331 = 0.0 ("element")
                    n1246 = local read "water # 4.1L"() -> (w333:dbl)
                    n1247 = local read "water # 4.2R"() -> (w332:dbl)
                    n1248 = local read "lick # 4.2R"() -> (w334:dbl)
                    n1249 = local read "lick # 4.1L"() -> (w336:dbl)
                    n1250 = local read "current sound"() -> (w327:dbl)
                    n1251 = Increment(x=w336) -> (x+1=w335:dbl)
                    n1252 = local read "mistake # 4.2R"() -> (w329:dbl)
                    n1253 = local read "time (s)"() -> (w337:dbl)
                    n1254 = local read "mistake # 4.1L"() -> (w330:dbl)
                    n1255 = local read "trial #"() -> (w328:dbl)
                    n1256 = local read "ITI (s)"() -> (w326:dbl)
                    n1257 = local write "lick # 4.1L"(w335) -> ()
                    n1258 = Build Array(w337, w335, w334, w333, w332, w331, w331, w328, w327, w326, w331, w330, w329) -> (w338:dbl[])
                    n1259 = local read "Mouse path 4"() -> (w339:path)
                    n1260 = call-poly <vilib>:"Write To Spreadsheet File.vi"("append to file? (new file:F)"=TRUE, "1D data"=w338, "file path (dialog if empty)"=w339) -> ()  [unwired: 5 in, 1 out]
                  }
                  frame "ITI" {
                    w346 = 0.0 ("element")
                    n1261 = local read "water # 4.2R"() -> (w347:dbl)
                    n1262 = local read "lick # 4.2R"() -> (w349:dbl)
                    n1263 = local read "water # 4.1L"() -> (w348:dbl)
                    n1264 = local read "lick # 4.1L"() -> (w351:dbl)
                    n1265 = local read "current sound"() -> (w342:dbl)
                    n1266 = local read "trial #"() -> (w343:dbl)
                    n1267 = local read "ITI (s)"() -> (w341:dbl)
                    n1268 = Increment(x=w351) -> (x+1=w350:dbl)
                    n1269 = local read "time (s)"() -> (w352:dbl)
                    n1270 = local read "mistake # 4.1L"() -> (w345:dbl)
                    n1271 = local read "mistake # 4.2R"() -> (w344:dbl)
                    n1272 = local write "lick # 4.1L"(w350) -> ()
                    n1273 = local read "Mouse path 4"() -> (w354:path)
                    n1274 = Build Array(w352, w350, w349, w348, w347, w346, w346, w343, w342, w341, w346, w345, w344) -> (w353:dbl[])
                    n1275 = call-poly <vilib>:"Write To Spreadsheet File.vi"("append to file? (new file:F)"=TRUE, "1D data"=w353, "file path (dialog if empty)"=w354) -> ()  [unwired: 5 in, 1 out]
                  }
                }
              }
            }
          }
          frame 4 {
            n1276 = case shown="True" w407 {
              frame False {
              }
              frame True {
                n1277 = local read "state 4.2"() -> (w460:enum16{"waiting", "sound", "ITI"})
                n1278 = case shown="\"waiting\", Default" w460 {
                  frame "waiting", Default {
                    w468 = 0.0 ("element")
                    n1279 = local read "water # 4.2R"() -> (w470:dbl)
                    n1280 = local read "lick # 4.2R"() -> (w473:dbl)
                    n1281 = local read "water # 4.1L"() -> (w471:dbl)
                    n1282 = local read "lick # 4.1L"() -> (w474:dbl)
                    n1283 = local read "current sound"() -> (w462:dbl)
                    n1284 = local read "trial #"() -> (w463:dbl)
                    n1285 = local read "mistake # 4.2R"() -> (w466:dbl)
                    n1286 = local read "time (s)"() -> (w465:dbl)
                    n1287 = local read "ITI (s)"() -> (w461:dbl)
                    n1288 = Increment(x=w473) -> (x+1=w472:dbl)
                    n1289 = local read "mistake # 4.1L"() -> (w467:dbl)
                    n1290 = Increment(x=w470) -> (x+1=w469:dbl)
                    n1291 = local write "water # 4.2R"(w469) -> ()
                    n1292 = local write "state 4.2"(enum16{"waiting", "sound", "ITI"}."ITI") -> ()
                    n1293 = local write "lick # 4.2R"(w472) -> ()
                    n1294 = local write "last water 4.2R"(w465) -> ()
                    n1295 = local read "Mouse path 4"() -> (w476:path)
                    n1296 = local write "state 4.1"(enum16{"waiting", "sound", "ITI"}."ITI") -> ()
                    n1297 = local read "free water 4.2"() -> (w478:bool)
                    n1298 = Build Array(w465, w474, w472, w471, w469, 1.0 ("element"), w468, w463, w462, w461, w468, w467, w466) -> (w475:dbl[])
                    n1299 = call-poly <vilib>:"Write To Spreadsheet File.vi"("append to file? (new file:F)"=TRUE, "1D data"=w475, "file path (dialog if empty)"=w476) -> ()  [unwired: 5 in, 1 out]
                    n1300 = case shown="False" w478 {
                      frame False {
                        n1301 = local read "water dur (ms) 4.2"() -> (w481:dbl)
                        n1302 = local read "water port 4.2"() -> (w482:tag)
                        n1303 = call "_digital_on_duration_off.vi"("duration (ms)"=w481, "digital port"=w482) -> ()  [unwired: 10 in]
                      }
                      frame True {
                      }
                    }
                  }
                  frame "sound" {
                    w486 = 0.0 ("element")
                    n1304 = local read "water # 4.2R"() -> (w489:dbl)
                    n1305 = local read "water # 4.1L"() -> (w490:dbl)
                    n1306 = local read "current sound"() -> (w484:dbl)
                    n1307 = local read "lick # 4.2R"() -> (w492:dbl)
                    n1308 = local read "trial #"() -> (w485:dbl)
                    n1309 = local read "lick # 4.1L"() -> (w493:dbl)
                    n1310 = local read "ITI (s)"() -> (w483:dbl)
                    n1311 = local read "mistake # 4.2R"() -> (w487:dbl)
                    n1312 = Increment(x=w492) -> (x+1=w491:dbl)
                    n1313 = local read "mistake # 4.1L"() -> (w488:dbl)
                    n1314 = local write "lick # 4.2R"(w491) -> ()
                    n1315 = local read "time (s)"() -> (w494:dbl)
                    n1316 = Build Array(w494, w493, w491, w490, w489, w486, w486, w485, w484, w483, w486, w488, w487) -> (w495:dbl[])
                    n1317 = local read "Mouse path 4"() -> (w496:path)
                    n1318 = call-poly <vilib>:"Write To Spreadsheet File.vi"("append to file? (new file:F)"=TRUE, "1D data"=w495, "file path (dialog if empty)"=w496) -> ()  [unwired: 5 in, 1 out]
                  }
                  frame "ITI" {
                    w503 = 0.0 ("element")
                    n1319 = local read "water # 4.2R"() -> (w504:dbl)
                    n1320 = local read "lick # 4.2R"() -> (w507:dbl)
                    n1321 = local read "water # 4.1L"() -> (w505:dbl)
                    n1322 = local read "lick # 4.1L"() -> (w508:dbl)
                    n1323 = local read "current sound"() -> (w499:dbl)
                    n1324 = local read "ITI (s)"() -> (w498:dbl)
                    n1325 = local read "trial #"() -> (w500:dbl)
                    n1326 = Increment(x=w507) -> (x+1=w506:dbl)
                    n1327 = local read "mistake # 4.2R"() -> (w501:dbl)
                    n1328 = local read "mistake # 4.1L"() -> (w502:dbl)
                    n1329 = local read "time (s)"() -> (w509:dbl)
                    n1330 = local write "lick # 4.2R"(w506) -> ()
                    n1331 = Build Array(w509, w508, w506, w505, w504, w503, w503, w500, w499, w498, w503, w502, w501) -> (w510:dbl[])
                    n1332 = local read "Mouse path 4"() -> (w511:path)
                    n1333 = call-poly <vilib>:"Write To Spreadsheet File.vi"("append to file? (new file:F)"=TRUE, "1D data"=w510, "file path (dialog if empty)"=w511) -> ()  [unwired: 5 in, 1 out]
                  }
                }
              }
            }
            n1334 = case shown="True" w408 {
              frame False {
              }
              frame True {
                n1335 = local read "state 4.2"() -> (w409:enum16{"waiting", "sound", "ITI"})
                n1336 = case shown="\"waiting\", Default" w409 {
                  frame "waiting", Default {
                    w411 = 0.0 ("element")
                    n1337 = local read "current sound"() -> (w414:dbl)
                    n1338 = local read "trial #"() -> (w415:dbl)
                    n1339 = local read "LED 4"() -> (w417:tag)
                    n1340 = local read "water # 4.2R"() -> (w419:dbl)
                    n1341 = local read "water # 4.1L"() -> (w420:dbl)
                    n1342 = local read "lick # 4.2R"() -> (w421:dbl)
                    n1343 = local read "lick # 4.1L"() -> (w423:dbl)
                    n1344 = local read "ITI (s)"() -> (w410:dbl)
                    n1345 = local write "LED 4 (i)"(1.0 ("LED 4 (i)")) -> ()
                    n1346 = local read "mistake # 4.2R"() -> (w418:dbl)
                    n1347 = local read "mistake # 4.1L"() -> (w412:dbl)
                    n1348 = local read "time (s)"() -> (w424:dbl)
                    n1349 = Increment(x=w423) -> (x+1=w422:dbl)
                    n1350 = call "_digital_on.vi"("digital port"=w417) -> ()  [unwired: 11 in]
                    n1351 = Increment(x=w418) -> (x+1=w413:dbl)
                    n1352 = local write "lick # 4.1L"(w422) -> ()
                    n1353 = local write "mistake # 4.2R"(w413) -> ()
                    n1354 = local read "Mouse path 4"() -> (w426:path)
                    n1355 = Build Array(w424, w422, w421, w420, w419, w411, w411, w415, w414, w410, w411, w412, w413) -> (w425:dbl[])
                    n1356 = local write "state 4.1"(enum16{"waiting", "sound", "ITI"}."ITI") -> ()
                    n1357 = local write "state 4.2"(enum16{"waiting", "sound", "ITI"}."ITI") -> ()
                    n1358 = call-poly <vilib>:"Write To Spreadsheet File.vi"("append to file? (new file:F)"=TRUE, "1D data"=w425, "file path (dialog if empty)"=w426) -> ()  [unwired: 5 in, 1 out]
                  }
                  frame "sound" {
                    w435 = 0.0 ("element")
                    n1359 = local read "lick # 4.2R"() -> (w438:dbl)
                    n1360 = local read "water # 4.2R"() -> (w436:dbl)
                    n1361 = local read "current sound"() -> (w431:dbl)
                    n1362 = local read "water # 4.1L"() -> (w437:dbl)
                    n1363 = local read "lick # 4.1L"() -> (w440:dbl)
                    n1364 = local read "trial #"() -> (w432:dbl)
                    n1365 = local read "ITI (s)"() -> (w430:dbl)
                    n1366 = local read "time (s)"() -> (w441:dbl)
                    n1367 = local read "mistake # 4.2R"() -> (w433:dbl)
                    n1368 = local read "mistake # 4.1L"() -> (w434:dbl)
                    n1369 = Increment(x=w440) -> (x+1=w439:dbl)
                    n1370 = local write "lick # 4.1L"(w439) -> ()
                    n1371 = local read "Mouse path 4"() -> (w443:path)
                    n1372 = Build Array(w441, w439, w438, w437, w436, w435, w435, w432, w431, w430, w435, w434, w433) -> (w442:dbl[])
                    n1373 = call-poly <vilib>:"Write To Spreadsheet File.vi"("append to file? (new file:F)"=TRUE, "1D data"=w442, "file path (dialog if empty)"=w443) -> ()  [unwired: 5 in, 1 out]
                  }
                  frame "ITI" {
                    w450 = 0.0 ("element")
                    n1374 = local read "current sound"() -> (w446:dbl)
                    n1375 = local read "water # 4.2R"() -> (w451:dbl)
                    n1376 = local read "water # 4.1L"() -> (w452:dbl)
                    n1377 = local read "lick # 4.2R"() -> (w453:dbl)
                    n1378 = local read "trial #"() -> (w447:dbl)
                    n1379 = local read "lick # 4.1L"() -> (w455:dbl)
                    n1380 = local read "ITI (s)"() -> (w445:dbl)
                    n1381 = local read "time (s)"() -> (w456:dbl)
                    n1382 = local read "mistake # 4.1L"() -> (w449:dbl)
                    n1383 = local read "mistake # 4.2R"() -> (w448:dbl)
                    n1384 = Increment(x=w455) -> (x+1=w454:dbl)
                    n1385 = local write "lick # 4.1L"(w454) -> ()
                    n1386 = local read "Mouse path 4"() -> (w458:path)
                    n1387 = Build Array(w456, w454, w453, w452, w451, w450, w450, w447, w446, w445, w450, w449, w448) -> (w457:dbl[])
                    n1388 = call-poly <vilib>:"Write To Spreadsheet File.vi"("append to file? (new file:F)"=TRUE, "1D data"=w457, "file path (dialog if empty)"=w458) -> ()  [unwired: 5 in, 1 out]
                  }
                }
              }
            }
          }
        }
        n1389 = case shown="1" w71 {
          tunnel: w73 -> [_ w1362 w1469 w1578 w1684]
          tunnel: w72 -> [_ w1361 w1470 w1577 w1683]
          frame 0, Default {
          }
          frame 1 {
            n1390 = case shown="True" w1361 {
              frame False {
              }
              frame True {
                n1391 = local read "state 1.2"() -> (w1363:enum16{"waiting", "sound", "ITI"})
                n1392 = case shown="\"sound\"" w1363 {
                  frame "waiting", Default {
                    w1374 = 0
                    n1393 = local read "LED 1"() -> (w1364:tag)
                    n1394 = local read "water # 1.2R"() -> (w1368:dbl)
                    n1395 = local read "water # 1.1L"() -> (w1380:dbl)
                    n1396 = call "_digital_on.vi"("digital port"=w1364) -> ()  [unwired: 11 in]
                    n1397 = local read "lick # 1.2R"() -> (w1378:dbl)
                    n1398 = local read "lick # 1.1L"() -> (w1377:dbl)
                    n1399 = local read "current sound"() -> (w1382:dbl)
                    n1400 = local read "time (s)"() -> (w1376:dbl)
                    n1401 = local read "trial #"() -> (w1381:dbl)
                    n1402 = local write "LED 1(i)"(1.0 ("LED 1(i)")) -> ()
                    n1403 = local read "mistake # 1.1L"() -> (w1370:dbl)
                    n1404 = Increment(x=w1378) -> (x+1=w1379:dbl)
                    n1405 = local read "mistake # 1.2R"() -> (w1372:dbl)
                    n1406 = local write "lick # 1.2R"(w1379) -> ()
                    n1407 = local write "state 1.2"(enum16{"waiting", "sound", "ITI"}."ITI") -> ()
                    n1408 = local write "state 1.1"(enum16{"waiting", "sound", "ITI"}."ITI") -> ()
                    n1409 = local read "ITI (s)"() -> (w1383:dbl)
                    n1410 = Increment(x=w1370) -> (x+1=w1369:dbl)
                    n1411 = local read "Mouse path 1"() -> (w1373:path)
                    n1412 = local write "mistake # 1.1L"(w1369) -> ()
                    n1413 = Build Array(w1376, w1377, w1379, w1380, w1368, 0.0 ("element"), w1374, w1381, w1382, w1383, w1374, w1369, w1372) -> (w1384:dbl[])
                    n1414 = call-poly <vilib>:"Write To Spreadsheet File.vi"("append to file? (new file:F)"=TRUE, "1D data"=w1384, "file path (dialog if empty)"=w1373) -> ()  [unwired: 5 in, 1 out]
                  }
                  frame "ITI" {
                    w1387 = 0 ("element")
                    n1415 = local read "lick # 1.2R"() -> (w1394:dbl)
                    n1416 = local read "water # 1.1L"() -> (w1392:dbl)
                    n1417 = local read "water # 1.2R"() -> (w1391:dbl)
                    n1418 = local read "lick # 1.1L"() -> (w1395:dbl)
                    n1419 = local read "mistake # 1.2R"() -> (w1385:dbl)
                    n1420 = local read "current sound"() -> (w1389:dbl)
                    n1421 = local read "mistake # 1.1L"() -> (w1386:dbl)
                    n1422 = local read "time (s)"() -> (w1396:dbl)
                    n1423 = local read "trial #"() -> (w1390:dbl)
                    n1424 = local read "ITI (s)"() -> (w1388:dbl)
                    n1425 = Increment(x=w1394) -> (x+1=w1393:dbl)
                    n1426 = local write "lick # 1.2R"(w1393) -> ()
                    n1427 = local read "Mouse path 1"() -> (w1399:path)
                    n1428 = Build Array(w1396, w1395, w1393, w1392, w1391, w1387, w1387, w1390, w1389, w1388, w1387, w1386, w1385) -> (w1397:dbl[])
                    n1429 = call-poly <vilib>:"Write To Spreadsheet File.vi"("append to file? (new file:F)"=TRUE, "1D data"=w1397, "file path (dialog if empty)"=w1399) -> ()  [unwired: 5 in, 1 out]
                  }
                  frame "sound" {
                    w1402 = 0 ("element")
                    n1430 = local read "water # 1.2R"() -> (w1406:dbl)
                    n1431 = local read "water # 1.1L"() -> (w1407:dbl)
                    n1432 = local read "lick # 1.2R"() -> (w1409:dbl)
                    n1433 = local read "lick # 1.1L"() -> (w1410:dbl)
                    n1434 = Increment(x=w1409) -> (x+1=w1408:dbl)
                    n1435 = local read "mistake # 1.2R"() -> (w1400:dbl)
                    n1436 = local read "mistake # 1.1L"() -> (w1401:dbl)
                    n1437 = local read "current sound"() -> (w1404:dbl)
                    n1438 = local read "time (s)"() -> (w1411:dbl)
                    n1439 = local write "lick # 1.2R"(w1408) -> ()
                    n1440 = local read "ITI (s)"() -> (w1403:dbl)
                    n1441 = local read "trial #"() -> (w1405:dbl)
                    n1442 = local read "Mouse path 1"() -> (w1414:path)
                    n1443 = Build Array(w1411, w1410, w1408, w1407, w1406, w1402, w1402, w1405, w1404, w1403, w1402, w1401, w1400) -> (w1412:dbl[])
                    n1444 = call-poly <vilib>:"Write To Spreadsheet File.vi"("append to file? (new file:F)"=TRUE, "1D data"=w1412, "file path (dialog if empty)"=w1414) -> ()  [unwired: 5 in, 1 out]
                  }
                }
              }
            }
            n1445 = case shown="True" w1362 {
              frame False {
              }
              frame True {
                n1446 = local read "Mouse path 1"() -> (w1415:path)
                n1447 = local read "state 1.1"() -> (w1416:enum16{"waiting", "sound", "ITI"})
                n1448 = case shown="\"waiting\", Default" w1416 {
                  tunnel: w1415 -> [w1423 _ w1456]
                  frame "waiting", Default {
                    w1428 = 0
                    n1449 = local read "time (s)"() -> (w1435:dbl)
                    n1450 = local read "lick # 1.1L"() -> (w1434:dbl)
                    n1451 = local read "water # 1.1L"() -> (w1433:dbl)
                    n1452 = local write "state 1.2"(enum16{"waiting", "sound", "ITI"}."ITI") -> ()
                    n1453 = local write "state 1.1"(enum16{"waiting", "sound", "ITI"}."ITI") -> ()
                    n1454 = local write "last water 1.1L"(w1435) -> ()
                    n1455 = Increment(x=w1433) -> (x+1=w1431:dbl)
                    n1456 = Increment(x=w1434) -> (x+1=w1432:dbl)
                    n1457 = local write "lick # 1.1L"(w1432) -> ()
                    n1458 = local write "water # 1.1L"(w1431) -> ()
                    n1459 = local read "lick # 1.2R"() -> (w1422:dbl)
                    n1460 = local read "free water 1.1"() -> (w1419:bool)
                    n1461 = local read "current sound"() -> (w1426:dbl)
                    n1462 = local read "trial #"() -> (w1427:dbl)
                    n1463 = local read "water # 1.2R"() -> (w1430:dbl)
                    n1464 = case shown="False" w1419 {
                      frame False {
                        n1465 = call "_digital_on_duration_off.vi"("duration (ms)"="water dur (ms) 1.1", "digital port"="water port 1.1") -> ()  [unwired: 10 in]
                      }
                      frame True {
                      }
                    }
                    n1466 = local read "ITI (s)"() -> (w1425:dbl)
                    n1467 = local read "mistake # 1.1L"() -> (w1421:dbl)
                    n1468 = local read "mistake # 1.2R"() -> (w1420:dbl)
                    n1469 = Build Array(w1435, w1432, w1422, w1431, w1430, 1, w1428, w1427, w1426, w1425, w1428, w1421, w1420) -> (w1424:dbl[])
                    n1470 = call-poly <vilib>:"Write To Spreadsheet File.vi"("append to file? (new file:F)"=TRUE, "1D data"=w1424, "file path (dialog if empty)"=w1423) -> ()  [unwired: 5 in, 1 out]
                  }
                  frame "sound" {
                    w1441 = 0 ("element")
                    n1471 = local read "mistake # 1.2R"() -> (w1439:dbl)
                    n1472 = local read "water # 1.2R"() -> (w1445:dbl)
                    n1473 = local read "water # 1.1L"() -> (w1446:dbl)
                    n1474 = local read "mistake # 1.1L"() -> (w1440:dbl)
                    n1475 = local read "current sound"() -> (w1443:dbl)
                    n1476 = local read "trial #"() -> (w1444:dbl)
                    n1477 = local read "lick # 1.2R"() -> (w1447:dbl)
                    n1478 = local read "lick # 1.1L"() -> (w1449:dbl)
                    n1479 = local read "ITI (s)"() -> (w1442:dbl)
                    n1480 = Increment(x=w1449) -> (x+1=w1448:dbl)
                    n1481 = local read "time (s)"() -> (w1450:dbl)
                    n1482 = local write "lick # 1.1L"(w1448) -> ()
                    n1483 = local read "Mouse path 1"() -> (w1452:path)
                    n1484 = Build Array(w1450, w1448, w1447, w1446, w1445, w1441, w1441, w1444, w1443, w1442, w1441, w1440, w1439) -> (w1451:dbl[])
                    n1485 = call-poly <vilib>:"Write To Spreadsheet File.vi"("append to file? (new file:F)"=TRUE, "1D data"=w1451, "file path (dialog if empty)"=w1452) -> ()  [unwired: 5 in, 1 out]
                  }
                  frame "ITI" {
                    w1462 = 0
                    n1486 = local read "time (s)"() -> (w1467:dbl)
                    n1487 = local read "lick # 1.1L"() -> (w1466:dbl)
                    n1488 = local read "lick # 1.2R"() -> (w1457:dbl)
                    n1489 = Increment(x=w1466) -> (x+1=w1465:dbl)
                    n1490 = local read "water # 1.1L"() -> (w1464:dbl)
                    n1491 = local read "water # 1.2R"() -> (w1463:dbl)
                    n1492 = local write "lick # 1.1L"(w1465) -> ()
                    n1493 = local read "current sound"() -> (w1460:dbl)
                    n1494 = local read "ITI (s)"() -> (w1459:dbl)
                    n1495 = local read "trial #"() -> (w1461:dbl)
                    n1496 = local read "mistake # 1.2R"() -> (w1454:dbl)
                    n1497 = local read "mistake # 1.1L"() -> (w1455:dbl)
                    n1498 = Build Array(w1467, w1465, w1457, w1464, w1463, w1462, w1462, w1461, w1460, w1459, w1462, w1455, w1454) -> (w1458:dbl[])
                    n1499 = call-poly <vilib>:"Write To Spreadsheet File.vi"("append to file? (new file:F)"=TRUE, "1D data"=w1458, "file path (dialog if empty)"=w1456) -> ()  [unwired: 5 in, 1 out]
                  }
                }
              }
            }
          }
          frame 2 {
            n1500 = case shown="True" w1469 {
              frame False {
              }
              frame True {
                n1501 = local read "state 1.1"() -> (w1471:enum16{"waiting", "sound", "ITI"})
                n1502 = case shown="\"waiting\", Default" w1471 {
                  frame "waiting", Default {
                    w1480 = 0
                    n1503 = local read "LED 1"() -> (w1472:tag)
                    n1504 = local read "water # 1.1L"() -> (w1474:dbl)
                    n1505 = local read "lick # 1.2R"() -> (w1486:dbl)
                    n1506 = call "_digital_on.vi"("digital port"=w1472) -> ()  [unwired: 11 in]
                    n1507 = local read "water # 1.2R"() -> (w1487:dbl)
                    n1508 = local read "time (s)"() -> (w1483:dbl)
                    n1509 = local read "current sound"() -> (w1489:dbl)
                    n1510 = local read "lick # 1.1L"() -> (w1484:dbl)
                    n1511 = local write "state 1.2"(enum16{"waiting", "sound", "ITI"}."ITI") -> ()
                    n1512 = local write "state 1.1"(enum16{"waiting", "sound", "ITI"}."ITI") -> ()
                    n1513 = local read "mistake # 1.2R"() -> (w1477:dbl)
                    n1514 = local read "ITI (s)"() -> (w1490:dbl)
                    n1515 = Increment(x=w1484) -> (x+1=w1485:dbl)
                    n1516 = local write "lick # 1.1L"(w1485) -> ()
                    n1517 = local read "mistake # 1.1L"() -> (w1479:dbl)
                    n1518 = local read "trial #"() -> (w1488:dbl)
                    n1519 = Increment(x=w1477) -> (x+1=w1476:dbl)
                    n1520 = local read "Mouse path 1"() -> (w1492:path)
                    n1521 = local write "mistake # 1.2R"(w1476) -> ()
                    n1522 = Build Array(w1483, w1485, w1486, w1474, w1487, 0.0 ("element"), w1480, w1488, w1489, w1490, w1480, w1479, w1476) -> (w1491:dbl[])
                    n1523 = call-poly <vilib>:"Write To Spreadsheet File.vi"("append to file? (new file:F)"=TRUE, "1D data"=w1491, "file path (dialog if empty)"=w1492) -> ()  [unwired: 5 in, 1 out]
                    n1524 = local write "LED 1(i)"(1.0 ("LED 1(i)")) -> ()
                  }
                  frame "ITI" {
                    w1495 = 0 ("element")
                    n1525 = local read "lick # 1.1L"() -> (w1503:dbl)
                    n1526 = local read "water # 1.2R"() -> (w1499:dbl)
                    n1527 = local read "water # 1.1L"() -> (w1500:dbl)
                    n1528 = local read "lick # 1.2R"() -> (w1501:dbl)
                    n1529 = local read "mistake # 1.2R"() -> (w1493:dbl)
                    n1530 = local read "current sound"() -> (w1497:dbl)
                    n1531 = local read "mistake # 1.1L"() -> (w1494:dbl)
                    n1532 = local read "trial #"() -> (w1498:dbl)
                    n1533 = Increment(x=w1503) -> (x+1=w1502:dbl)
                    n1534 = local read "time (s)"() -> (w1504:dbl)
                    n1535 = local read "ITI (s)"() -> (w1496:dbl)
                    n1536 = local write "lick # 1.1L"(w1502) -> ()
                    n1537 = Build Array(w1504, w1502, w1501, w1500, w1499, w1495, w1495, w1498, w1497, w1496, w1495, w1494, w1493) -> (w1505:dbl[])
                    n1538 = local read "Mouse path 1"() -> (w1507:path)
                    n1539 = call-poly <vilib>:"Write To Spreadsheet File.vi"("append to file? (new file:F)"=TRUE, "1D data"=w1505, "file path (dialog if empty)"=w1507) -> ()  [unwired: 5 in, 1 out]
                  }
                  frame "sound" {
                    w1510 = 0 ("element")
                    n1540 = local read "water # 1.2R"() -> (w1514:dbl)
                    n1541 = local read "water # 1.1L"() -> (w1515:dbl)
                    n1542 = local read "lick # 1.2R"() -> (w1516:dbl)
                    n1543 = local read "mistake # 1.2R"() -> (w1508:dbl)
                    n1544 = local read "mistake # 1.1L"() -> (w1509:dbl)
                    n1545 = local read "current sound"() -> (w1512:dbl)
                    n1546 = local read "lick # 1.1L"() -> (w1518:dbl)
                    n1547 = local read "trial #"() -> (w1513:dbl)
                    n1548 = local read "ITI (s)"() -> (w1511:dbl)
                    n1549 = local read "time (s)"() -> (w1519:dbl)
                    n1550 = Increment(x=w1518) -> (x+1=w1517:dbl)
                    n1551 = local write "lick # 1.1L"(w1517) -> ()
                    n1552 = local read "Mouse path 1"() -> (w1522:path)
                    n1553 = Build Array(w1519, w1517, w1516, w1515, w1514, w1510, w1510, w1513, w1512, w1511, w1510, w1509, w1508) -> (w1520:dbl[])
                    n1554 = call-poly <vilib>:"Write To Spreadsheet File.vi"("append to file? (new file:F)"=TRUE, "1D data"=w1520, "file path (dialog if empty)"=w1522) -> ()  [unwired: 5 in, 1 out]
                  }
                }
              }
            }
            n1555 = case shown="True" w1470 {
              frame False {
              }
              frame True {
                n1556 = local read "Mouse path 1"() -> (w1523:path)
                n1557 = local read "state 1.2"() -> (w1524:enum16{"waiting", "sound", "ITI"})
                n1558 = case shown="\"waiting\", Default" w1524 {
                  tunnel: w1523 -> [w1532 _ w1564]
                  frame "waiting", Default {
                    w1538 = 0
                    n1559 = local read "lick # 1.1L"() -> (w1531:dbl)
                    n1560 = local read "lick # 1.2R"() -> (w1530:dbl)
                    n1561 = local read "time (s)"() -> (w1543:dbl)
                    n1562 = local read "water # 1.2R"() -> (w1541:dbl)
                    n1563 = Increment(x=w1530) -> (x+1=w1529:dbl)
                    n1564 = local write "last water 1.2R"(w1543) -> ()
                    n1565 = local write "lick # 1.2R"(w1529) -> ()
                    n1566 = Increment(x=w1541) -> (x+1=w1540:dbl)
                    n1567 = local read "free water 1.2"() -> (w1526:bool)
                    n1568 = local write "water # 1.2R"(w1540) -> ()
                    n1569 = case shown="False" w1526 {
                      frame False {
                        n1570 = call "_digital_on_duration_off.vi"("duration (ms)"="water dur (ms) 1.2", "digital port"="water port 1.2") -> ()  [unwired: 10 in]
                      }
                      frame True {
                      }
                    }
                    n1571 = local read "water # 1.1L"() -> (w1542:dbl)
                    n1572 = local read "current sound"() -> (w1536:dbl)
                    n1573 = local read "trial #"() -> (w1537:dbl)
                    n1574 = local read "mistake # 1.2R"() -> (w1527:dbl)
                    n1575 = local read "mistake # 1.1L"() -> (w1528:dbl)
                    n1576 = local read "ITI (s)"() -> (w1535:dbl)
                    n1577 = Build Array(w1543, w1531, w1529, w1542, w1540, 1, w1538, w1537, w1536, w1535, w1538, w1528, w1527) -> (w1534:dbl[])
                    n1578 = local write "state 1.1"(enum16{"waiting", "sound", "ITI"}."ITI") -> ()
                    n1579 = local write "state 1.2"(enum16{"waiting", "sound", "ITI"}."ITI") -> ()
                    n1580 = call-poly <vilib>:"Write To Spreadsheet File.vi"("append to file? (new file:F)"=TRUE, "1D data"=w1534, "file path (dialog if empty)"=w1532) -> ()  [unwired: 5 in, 1 out]
                  }
                  frame "sound" {
                    w1549 = 0 ("element")
                    n1581 = local read "water # 1.2R"() -> (w1553:dbl)
                    n1582 = local read "water # 1.1L"() -> (w1554:dbl)
                    n1583 = local read "lick # 1.1L"() -> (w1556:dbl)
                    n1584 = local read "lick # 1.2R"() -> (w1557:dbl)
                    n1585 = local read "current sound"() -> (w1551:dbl)
                    n1586 = local read "mistake # 1.1L"() -> (w1548:dbl)
                    n1587 = local read "ITI (s)"() -> (w1550:dbl)
                    n1588 = local read "mistake # 1.2R"() -> (w1547:dbl)
                    n1589 = local read "trial #"() -> (w1552:dbl)
                    n1590 = local read "time (s)"() -> (w1558:dbl)
                    n1591 = Increment(x=w1557) -> (x+1=w1555:dbl)
                    n1592 = local write "lick # 1.2R"(w1555) -> ()
                    n1593 = local read "Mouse path 1"() -> (w1561:path)
                    n1594 = Build Array(w1558, w1556, w1555, w1554, w1553, w1549, w1549, w1552, w1551, w1550, w1549, w1548, w1547) -> (w1559:dbl[])
                    n1595 = call-poly <vilib>:"Write To Spreadsheet File.vi"("append to file? (new file:F)"=TRUE, "1D data"=w1559, "file path (dialog if empty)"=w1561) -> ()  [unwired: 5 in, 1 out]
                  }
                  frame "ITI" {
                    w1570 = 0
                    n1596 = local read "lick # 1.1L"() -> (w1565:dbl)
                    n1597 = local read "lick # 1.2R"() -> (w1574:dbl)
                    n1598 = local read "time (s)"() -> (w1575:dbl)
                    n1599 = Increment(x=w1574) -> (x+1=w1573:dbl)
                    n1600 = local write "lick # 1.2R"(w1573) -> ()
                    n1601 = local read "water # 1.1L"() -> (w1572:dbl)
                    n1602 = local read "current sound"() -> (w1568:dbl)
                    n1603 = local read "water # 1.2R"() -> (w1571:dbl)
                    n1604 = local read "trial #"() -> (w1569:dbl)
                    n1605 = local read "mistake # 1.1L"() -> (w1563:dbl)
                    n1606 = local read "mistake # 1.2R"() -> (w1562:dbl)
                    n1607 = local read "ITI (s)"() -> (w1567:dbl)
                    n1608 = Build Array(w1575, w1565, w1573, w1572, w1571, w1570, w1570, w1569, w1568, w1567, w1570, w1563, w1562) -> (w1566:dbl[])
                    n1609 = call-poly <vilib>:"Write To Spreadsheet File.vi"("append to file? (new file:F)"=TRUE, "1D data"=w1566, "file path (dialog if empty)"=w1564) -> ()  [unwired: 5 in, 1 out]
                  }
                }
              }
            }
          }
          frame 3 {
            n1610 = case shown="True" w1578 {
              frame False {
              }
              frame True {
                n1611 = local read "state 1.1"() -> (w1630:enum16{"waiting", "sound", "ITI"})
                n1612 = case shown="\"waiting\", Default" w1630 {
                  frame "waiting", Default {
                    w1635 = 0 ("element")
                    n1613 = local read "water # 1.2R"() -> (w1640:dbl)
                    n1614 = local read "water # 1.1L"() -> (w1642:dbl)
                    n1615 = local read "lick # 1.2R"() -> (w1643:dbl)
                    n1616 = local read "lick # 1.1L"() -> (w1645:dbl)
                    n1617 = local read "time (s)"() -> (w1646:dbl)
                    n1618 = Increment(x=w1642) -> (x+1=w1641:dbl)
                    n1619 = Increment(x=w1645) -> (x+1=w1644:dbl)
                    n1620 = local write "state 1.1"(enum16{"waiting", "sound", "ITI"}."ITI") -> ()
                    n1621 = local write "water # 1.1L"(w1641) -> ()
                    n1622 = local read "Mouse path 1"() -> (w1648:path)
                    n1623 = local write "lick # 1.1L"(w1644) -> ()
                    n1624 = local write "last water 1.1L"(w1646) -> ()
                    n1625 = local read "current sound"() -> (w1637:dbl)
                    n1626 = local read "mistake # 1.2R"() -> (w1633:dbl)
                    n1627 = local read "mistake # 1.1L"() -> (w1634:dbl)
                    n1628 = local read "ITI (s)"() -> (w1636:dbl)
                    n1629 = local read "trial #"() -> (w1638:dbl)
                    n1630 = local read "free water 1.1"() -> (w1631:bool)
                    n1631 = local write "state 1.2"(enum16{"waiting", "sound", "ITI"}."ITI") -> ()
                    n1632 = case shown="False" w1631 {
                      frame False {
                        n1633 = local read "water port 1.1"() -> (w1651:tag)
                        n1634 = local read "water dur (ms) 1.1"() -> (w1652:dbl)
                        n1635 = call "_digital_on_duration_off.vi"("duration (ms)"=w1652, "digital port"=w1651) -> ()  [unwired: 10 in]
                      }
                      frame True {
                      }
                    }
                    n1636 = Build Array(w1646, w1644, w1643, w1641, w1640, 1 ("element"), w1635, w1638, w1637, w1636, w1635, w1634, w1633) -> (w1647:dbl[])
                    n1637 = call-poly <vilib>:"Write To Spreadsheet File.vi"("append to file? (new file:F)"=TRUE, "1D data"=w1647, "file path (dialog if empty)"=w1648) -> ()  [unwired: 5 in, 1 out]
                  }
                  frame "ITI" {
                    w1655 = 0 ("element")
                    n1638 = local read "water # 1.2R"() -> (w1659:dbl)
                    n1639 = local read "water # 1.1L"() -> (w1660:dbl)
                    n1640 = local read "lick # 1.1L"() -> (w1663:dbl)
                    n1641 = local read "lick # 1.2R"() -> (w1661:dbl)
                    n1642 = local read "current sound"() -> (w1657:dbl)
                    n1643 = local read "trial #"() -> (w1658:dbl)
                    n1644 = local read "ITI (s)"() -> (w1656:dbl)
                    n1645 = local read "time (s)"() -> (w1664:dbl)
                    n1646 = Increment(x=w1663) -> (x+1=w1662:dbl)
                    n1647 = local read "mistake # 1.1L"() -> (w1654:dbl)
                    n1648 = local read "mistake # 1.2R"() -> (w1653:dbl)
                    n1649 = local write "lick # 1.1L"(w1662) -> ()
                    n1650 = local read "Mouse path 1"() -> (w1667:path)
                    n1651 = Build Array(w1664, w1662, w1661, w1660, w1659, w1655, w1655, w1658, w1657, w1656, w1655, w1654, w1653) -> (w1665:dbl[])
                    n1652 = call-poly <vilib>:"Write To Spreadsheet File.vi"("append to file? (new file:F)"=TRUE, "1D data"=w1665, "file path (dialog if empty)"=w1667) -> ()  [unwired: 5 in, 1 out]
                  }
                  frame "sound" {
                    w1670 = 0 ("element")
                    n1653 = local read "water # 1.2R"() -> (w1674:dbl)
                    n1654 = local read "water # 1.1L"() -> (w1675:dbl)
                    n1655 = local read "lick # 1.2R"() -> (w1676:dbl)
                    n1656 = local read "lick # 1.1L"() -> (w1678:dbl)
                    n1657 = local read "current sound"() -> (w1672:dbl)
                    n1658 = local read "mistake # 1.2R"() -> (w1668:dbl)
                    n1659 = local read "ITI (s)"() -> (w1671:dbl)
                    n1660 = local read "trial #"() -> (w1673:dbl)
                    n1661 = local read "mistake # 1.1L"() -> (w1669:dbl)
                    n1662 = local read "time (s)"() -> (w1679:dbl)
                    n1663 = Increment(x=w1678) -> (x+1=w1677:dbl)
                    n1664 = local write "lick # 1.1L"(w1677) -> ()
                    n1665 = local read "Mouse path 1"() -> (w1682:path)
                    n1666 = Build Array(w1679, w1677, w1676, w1675, w1674, w1670, w1670, w1673, w1672, w1671, w1670, w1669, w1668) -> (w1680:dbl[])
                    n1667 = call-poly <vilib>:"Write To Spreadsheet File.vi"("append to file? (new file:F)"=TRUE, "1D data"=w1680, "file path (dialog if empty)"=w1682) -> ()  [unwired: 5 in, 1 out]
                  }
                }
              }
            }
            n1668 = case shown="True" w1577 {
              frame False {
              }
              frame True {
                n1669 = local read "state 1.2"() -> (w1579:enum16{"waiting", "sound", "ITI"})
                n1670 = case shown="\"waiting\", Default" w1579 {
                  frame "waiting", Default {
                    w1586 = 0 ("element")
                    n1671 = local read "water # 1.2R"() -> (w1590:dbl)
                    n1672 = local read "water # 1.1L"() -> (w1591:dbl)
                    n1673 = local read "lick # 1.2R"() -> (w1593:dbl)
                    n1674 = local read "lick # 1.1L"() -> (w1594:dbl)
                    n1675 = local read "current sound"() -> (w1588:dbl)
                    n1676 = local read "mistake # 1.1L"() -> (w1584:dbl)
                    n1677 = Increment(x=w1593) -> (x+1=w1592:dbl)
                    n1678 = local read "time (s)"() -> (w1595:dbl)
                    n1679 = local read "mistake # 1.2R"() -> (w1585:dbl)
                    n1680 = local read "trial #"() -> (w1589:dbl)
                    n1681 = local read "ITI (s)"() -> (w1587:dbl)
                    n1682 = local write "lick # 1.2R"(w1592) -> ()
                    n1683 = local write "state 1.1"(enum16{"waiting", "sound", "ITI"}."ITI") -> ()
                    n1684 = Increment(x=w1584) -> (x+1=w1583:dbl)
                    n1685 = local read "Mouse path 1"() -> (w1598:path)
                    n1686 = local write "mistake # 1.1L"(w1583) -> ()
                    n1687 = local write "LED 1(i)"(1.0 ("LED 1(i)")) -> ()
                    n1688 = Build Array(w1595, w1594, w1592, w1591, w1590, w1586, w1586, w1589, w1588, w1587, w1586, w1583, w1585) -> (w1597:dbl[])
                    n1689 = call-poly <vilib>:"Write To Spreadsheet File.vi"("append to file? (new file:F)"=TRUE, "1D data"=w1597, "file path (dialog if empty)"=w1598) -> ()  [unwired: 5 in, 1 out]
                    n1690 = local read "LED 1"() -> (w1580:tag)
                    n1691 = local write "state 1.2"(enum16{"waiting", "sound", "ITI"}."ITI") -> ()
                    n1692 = call "_digital_on.vi"("digital port"=w1580) -> ()  [unwired: 11 in]
                  }
                  frame "sound" {
                    w1602 = 0 ("element")
                    n1693 = local read "water # 1.2R"() -> (w1606:dbl)
                    n1694 = local read "water # 1.1L"() -> (w1607:dbl)
                    n1695 = local read "lick # 1.2R"() -> (w1609:dbl)
                    n1696 = local read "current sound"() -> (w1604:dbl)
                    n1697 = local read "mistake # 1.2R"() -> (w1600:dbl)
                    n1698 = local read "lick # 1.1L"() -> (w1610:dbl)
                    n1699 = local read "ITI (s)"() -> (w1603:dbl)
                    n1700 = local read "mistake # 1.1L"() -> (w1601:dbl)
                    n1701 = local read "trial #"() -> (w1605:dbl)
                    n1702 = Increment(x=w1609) -> (x+1=w1608:dbl)
                    n1703 = local read "time (s)"() -> (w1611:dbl)
                    n1704 = local write "lick # 1.2R"(w1608) -> ()
                    n1705 = local read "Mouse path 1"() -> (w1613:path)
                    n1706 = Build Array(w1611, w1610, w1608, w1607, w1606, w1602, w1602, w1605, w1604, w1603, w1602, w1601, w1600) -> (w1612:dbl[])
                    n1707 = call-poly <vilib>:"Write To Spreadsheet File.vi"("append to file? (new file:F)"=TRUE, "1D data"=w1612, "file path (dialog if empty)"=w1613) -> ()  [unwired: 5 in, 1 out]
                  }
                  frame "ITI" {
                    w1617 = 0 ("element")
                    n1708 = local read "water # 1.2R"() -> (w1621:dbl)
                    n1709 = local read "water # 1.1L"() -> (w1622:dbl)
                    n1710 = local read "lick # 1.2R"() -> (w1624:dbl)
                    n1711 = local read "current sound"() -> (w1619:dbl)
                    n1712 = local read "lick # 1.1L"() -> (w1625:dbl)
                    n1713 = local read "mistake # 1.2R"() -> (w1615:dbl)
                    n1714 = local read "mistake # 1.1L"() -> (w1616:dbl)
                    n1715 = local read "trial #"() -> (w1620:dbl)
                    n1716 = local read "ITI (s)"() -> (w1618:dbl)
                    n1717 = local read "time (s)"() -> (w1626:dbl)
                    n1718 = Increment(x=w1624) -> (x+1=w1623:dbl)
                    n1719 = local write "lick # 1.2R"(w1623) -> ()
                    n1720 = local read "Mouse path 1"() -> (w1629:path)
                    n1721 = Build Array(w1626, w1625, w1623, w1622, w1621, w1617, w1617, w1620, w1619, w1618, w1617, w1616, w1615) -> (w1627:dbl[])
                    n1722 = call-poly <vilib>:"Write To Spreadsheet File.vi"("append to file? (new file:F)"=TRUE, "1D data"=w1627, "file path (dialog if empty)"=w1629) -> ()  [unwired: 5 in, 1 out]
                  }
                }
              }
            }
          }
          frame 4 {
            n1723 = case shown="True" w1684 {
              frame False {
              }
              frame True {
                n1724 = local read "state 1.1"() -> (w1738:enum16{"waiting", "sound", "ITI"})
                n1725 = case shown="\"sound\"" w1738 {
                  frame "waiting", Default {
                    w1739 = 0 ("element")
                    n1726 = local read "water # 1.1L"() -> (w1750:dbl)
                    n1727 = local read "lick # 1.2R"() -> (w1751:dbl)
                    n1728 = local read "lick # 1.1L"() -> (w1753:dbl)
                    n1729 = local read "water # 1.2R"() -> (w1749:dbl)
                    n1730 = local read "mistake # 1.2R"() -> (w1745:dbl)
                    n1731 = local read "mistake # 1.1L"() -> (w1740:dbl)
                    n1732 = local read "current sound"() -> (w1747:dbl)
                    n1733 = local read "time (s)"() -> (w1754:dbl)
                    n1734 = Increment(x=w1753) -> (x+1=w1752:dbl)
                    n1735 = local read "trial #"() -> (w1748:dbl)
                    n1736 = local read "ITI (s)"() -> (w1746:dbl)
                    n1737 = local write "state 1.2"(enum16{"waiting", "sound", "ITI"}."ITI") -> ()
                    n1738 = local write "state 1.1"(enum16{"waiting", "sound", "ITI"}."ITI") -> ()
                    n1739 = local write "lick # 1.1L"(w1752) -> ()
                    n1740 = Increment(x=w1745) -> (x+1=w1741:dbl)
                    n1741 = local write "mistake # 1.2R"(w1741) -> ()
                    n1742 = local read "Mouse path 1"() -> (w1757:path)
                    n1743 = Build Array(w1754, w1752, w1751, w1750, w1749, w1739, w1739, w1748, w1747, w1746, w1739, w1740, w1741) -> (w1755:dbl[])
                    n1744 = local read "LED 1"() -> (w1742:tag)
                    n1745 = call-poly <vilib>:"Write To Spreadsheet File.vi"("append to file? (new file:F)"=TRUE, "1D data"=w1755, "file path (dialog if empty)"=w1757) -> ()  [unwired: 5 in, 1 out]
                    n1746 = call "_digital_on.vi"("digital port"=w1742) -> ()  [unwired: 11 in]
                    n1747 = local write "LED 1(i)"(1.0 ("LED 1(i)")) -> ()
                  }
                  frame "sound" {
                    w1761 = 0 ("element")
                    n1748 = local read "water # 1.2R"() -> (w1765:dbl)
                    n1749 = local read "water # 1.1L"() -> (w1766:dbl)
                    n1750 = local read "lick # 1.2R"() -> (w1767:dbl)
                    n1751 = local read "mistake # 1.2R"() -> (w1759:dbl)
                    n1752 = local read "current sound"() -> (w1763:dbl)
                    n1753 = local read "lick # 1.1L"() -> (w1769:dbl)
                    n1754 = local read "mistake # 1.1L"() -> (w1760:dbl)
                    n1755 = local read "trial #"() -> (w1764:dbl)
                    n1756 = local read "ITI (s)"() -> (w1762:dbl)
                    n1757 = local read "time (s)"() -> (w1770:dbl)
                    n1758 = Increment(x=w1769) -> (x+1=w1768:dbl)
                    n1759 = local read "Mouse path 1"() -> (w1773:path)
                    n1760 = local write "lick # 1.1L"(w1768) -> ()
                    n1761 = Build Array(w1770, w1768, w1767, w1766, w1765, w1761, w1761, w1764, w1763, w1762, w1761, w1760, w1759) -> (w1771:dbl[])
                    n1762 = call-poly <vilib>:"Write To Spreadsheet File.vi"("append to file? (new file:F)"=TRUE, "1D data"=w1771, "file path (dialog if empty)"=w1773) -> ()  [unwired: 5 in, 1 out]
                  }
                  frame "ITI" {
                    w1776 = 0 ("element")
                    n1763 = local read "water # 1.2R"() -> (w1780:dbl)
                    n1764 = local read "lick # 1.1L"() -> (w1784:dbl)
                    n1765 = local read "water # 1.1L"() -> (w1781:dbl)
                    n1766 = local read "lick # 1.2R"() -> (w1782:dbl)
                    n1767 = local read "mistake # 1.2R"() -> (w1774:dbl)
                    n1768 = local read "current sound"() -> (w1778:dbl)
                    n1769 = local read "mistake # 1.1L"() -> (w1775:dbl)
                    n1770 = Increment(x=w1784) -> (x+1=w1783:dbl)
                    n1771 = local read "trial #"() -> (w1779:dbl)
                    n1772 = local read "ITI (s)"() -> (w1777:dbl)
                    n1773 = local read "time (s)"() -> (w1785:dbl)
                    n1774 = local write "lick # 1.1L"(w1783) -> ()
                    n1775 = local read "Mouse path 1"() -> (w1788:path)
                    n1776 = Build Array(w1785, w1783, w1782, w1781, w1780, w1776, w1776, w1779, w1778, w1777, w1776, w1775, w1774) -> (w1786:dbl[])
                    n1777 = call-poly <vilib>:"Write To Spreadsheet File.vi"("append to file? (new file:F)"=TRUE, "1D data"=w1786, "file path (dialog if empty)"=w1788) -> ()  [unwired: 5 in, 1 out]
                  }
                }
              }
            }
            n1778 = case shown="True" w1683 {
              frame False {
              }
              frame True {
                n1779 = local read "state 1.2"() -> (w1685:enum16{"waiting", "sound", "ITI"})
                n1780 = case shown="\"waiting\", Default" w1685 {
                  frame "waiting", Default {
                    w1690 = 0 ("element")
                    n1781 = local read "water # 1.2R"() -> (w1696:dbl)
                    n1782 = local read "lick # 1.2R"() -> (w1699:dbl)
                    n1783 = local read "free water 1.2"() -> (w1686:bool)
                    n1784 = local read "water # 1.1L"() -> (w1697:dbl)
                    n1785 = local read "lick # 1.1L"() -> (w1700:dbl)
                    n1786 = local read "time (s)"() -> (w1701:dbl)
                    n1787 = local write "state 1.2"(enum16{"waiting", "sound", "ITI"}."ITI") -> ()
                    n1788 = local write "state 1.1"(enum16{"waiting", "sound", "ITI"}."ITI") -> ()
                    n1789 = Increment(x=w1696) -> (x+1=w1695:dbl)
                    n1790 = Increment(x=w1699) -> (x+1=w1698:dbl)
                    n1791 = case shown="False" w1686 {
                      frame False {
                        n1792 = local read "water dur (ms) 1.2"() -> (w1707:dbl)
                        n1793 = local read "water port 1.2"() -> (w1706:tag)
                        n1794 = call "_digital_on_duration_off.vi"("duration (ms)"=w1707, "digital port"=w1706) -> ()  [unwired: 10 in]
                      }
                      frame True {
                      }
                    }
                    n1795 = local write "water # 1.2R"(w1695) -> ()
                    n1796 = local write "lick # 1.2R"(w1698) -> ()
                    n1797 = local write "last water 1.2R"(w1701) -> ()
                    n1798 = local read "mistake # 1.2R"() -> (w1688:dbl)
                    n1799 = local read "mistake # 1.1L"() -> (w1689:dbl)
                    n1800 = local read "current sound"() -> (w1692:dbl)
                    n1801 = local read "ITI (s)"() -> (w1691:dbl)
                    n1802 = local read "trial #"() -> (w1693:dbl)
                    n1803 = local read "Mouse path 1"() -> (w1704:path)
                    n1804 = Build Array(w1701, w1700, w1698, w1697, w1695, 1 ("element"), w1690, w1693, w1692, w1691, w1690, w1689, w1688) -> (w1702:dbl[])
                    n1805 = call-poly <vilib>:"Write To Spreadsheet File.vi"("append to file? (new file:F)"=TRUE, "1D data"=w1702, "file path (dialog if empty)"=w1704) -> ()  [unwired: 5 in, 1 out]
                  }
                  frame "sound" {
                    w1710 = 0 ("element")
                    n1806 = local read "lick # 1.2R"() -> (w1717:dbl)
                    n1807 = local read "water # 1.2R"() -> (w1714:dbl)
                    n1808 = local read "water # 1.1L"() -> (w1715:dbl)
                    n1809 = local read "lick # 1.1L"() -> (w1718:dbl)
                    n1810 = local read "mistake # 1.2R"() -> (w1708:dbl)
                    n1811 = local read "current sound"() -> (w1712:dbl)
                    n1812 = Increment(x=w1717) -> (x+1=w1716:dbl)
                    n1813 = local read "mistake # 1.1L"() -> (w1709:dbl)
                    n1814 = local read "time (s)"() -> (w1719:dbl)
                    n1815 = local read "trial #"() -> (w1713:dbl)
                    n1816 = local read "ITI (s)"() -> (w1711:dbl)
                    n1817 = local write "lick # 1.2R"(w1716) -> ()
                    n1818 = local read "Mouse path 1"() -> (w1722:path)
                    n1819 = Build Array(w1719, w1718, w1716, w1715, w1714, w1710, w1710, w1713, w1712, w1711, w1710, w1709, w1708) -> (w1720:dbl[])
                    n1820 = call-poly <vilib>:"Write To Spreadsheet File.vi"("append to file? (new file:F)"=TRUE, "1D data"=w1720, "file path (dialog if empty)"=w1722) -> ()  [unwired: 5 in, 1 out]
                  }
                  frame "ITI" {
                    w1725 = 0 ("element")
                    n1821 = local read "water # 1.2R"() -> (w1729:dbl)
                    n1822 = local read "water # 1.1L"() -> (w1730:dbl)
                    n1823 = local read "lick # 1.2R"() -> (w1732:dbl)
                    n1824 = local read "lick # 1.1L"() -> (w1733:dbl)
                    n1825 = local read "mistake # 1.2R"() -> (w1723:dbl)
                    n1826 = local read "current sound"() -> (w1727:dbl)
                    n1827 = local read "mistake # 1.1L"() -> (w1724:dbl)
                    n1828 = Increment(x=w1732) -> (x+1=w1731:dbl)
                    n1829 = local read "ITI (s)"() -> (w1726:dbl)
                    n1830 = local read "trial #"() -> (w1728:dbl)
                    n1831 = local read "time (s)"() -> (w1734:dbl)
                    n1832 = local write "lick # 1.2R"(w1731) -> ()
                    n1833 = local read "Mouse path 1"() -> (w1737:path)
                    n1834 = Build Array(w1734, w1733, w1731, w1730, w1729, w1725, w1725, w1728, w1727, w1726, w1725, w1724, w1723) -> (w1735:dbl[])
                    n1835 = call-poly <vilib>:"Write To Spreadsheet File.vi"("append to file? (new file:F)"=TRUE, "1D data"=w1735, "file path (dialog if empty)"=w1737) -> ()  [unwired: 5 in, 1 out]
                  }
                }
              }
            }
          }
        }
        n1836 = call "_loop_time.vi"("from shift register"=w84) -> ("to shift register"=w83:dbl)  [unwired: 9 in, 1 out]
        n1837 = call "Elapsed Time"() -> ("Elapsed Time (s)"=→"time (s)":dbl)  [unwired: 12 in, 7 out]
      }
      n1838 = call <vilib>:"DAQmx Clear Task.vi"("task in"=w30) -> ()  [unwired: 14 in, 1 out]
      n1839 = while {
        shift-right: [w1792] -> _
        shift-left: T1."prepare" -> [w1791]
        stop <- FALSE stop-if-true
        n1840 = local write "trial state"(w1791) -> ()
        n1841 = case shown="\"free water\"" w1791 {
          tunnel: [w1793 w1873 w1902 w1917 w1923 T1."ITI" T1."prepare"] -> w1792
          frame "prepare", Default {
            n1842 = flat-sequence {
              tunnel: [T1."sound"] -> w1793
              frame #0 {
                w1797 = 500
                w1804 = 1000
                n1843 = Subtract(x="ITI max (ms)", y=w1797) -> (x-y=w1800:dbl)
                n1844 = Subtract(x="ITI min (ms)", y=w1797) -> (x-y=w1801:dbl)
                n1845 = local read "next sound"() -> (w1807:dbl[])
                n1846 = Divide(x=w1800, y=w1804) -> (x/y=w1795:dbl)
                n1847 = Divide(x=w1801, y=w1804) -> (x/y=w1794:dbl)
                n1848 = Delete From Array(array=w1807, index=0) -> (deleted portion=w1805:dbl, array with subset deleted=w1806:dbl[])  [unwired: 1 in]
                n1849 = local write "next sound"(w1806) -> ()
                n1850 = call "_random_integer.vi"("max"=w1795, "min"=w1794) -> ("output"=w1798:dbl)  [unwired: 9 in]
                n1851 = local write "current sound"(w1805) -> ()
                n1852 = Add(x=w1798, y=0.5) -> (x+y=w1799:dbl)
                n1853 = local write "ITI (s)"(w1799) -> ()
              }
              frame #1 {
                n1854 = local read "trial #"() -> (w1870:dbl)
                n1855 = local read "water # 3.2R"() -> (w1832:dbl)
                n1856 = local read "water # 3.1L"() -> (w1833:dbl)
                n1857 = local read "water # 2.2R"() -> (w1847:dbl)
                n1858 = local read "lick # 3.2R"() -> (w1834:dbl)
                n1859 = local read "current sound"() -> (w1813:dbl)
                n1860 = local read "water # 4.2R"() -> (w1817:dbl)
                n1861 = Increment(x=w1870) -> (x+1=w1814:dbl)
                n1862 = local read "water # 2.1L"() -> (w1848:dbl)
                n1863 = local read "water # 4.1L"() -> (w1818:dbl)
                n1864 = local read "mistake # 4.1L"() -> (w1810:dbl)
                n1865 = local read "mistake # 4.2R"() -> (w1809:dbl)
                n1866 = local read "lick # 3.1L"() -> (w1835:dbl)
                n1867 = local read "lick # 4.2R"() -> (w1819:dbl)
                n1868 = local read "lick # 4.1L"() -> (w1820:dbl)
                n1869 = local read "current sound"() -> (w1829:dbl)
                n1870 = local read "ITI (s)"() -> (w1812:dbl)
                n1871 = local read "lick  #  2.1L"() -> (w1850:dbl)
                n1872 = local read "lick  #  2.2R"() -> (w1849:dbl)
                n1873 = local read "ITI (s)"() -> (w1828:dbl)
                n1874 = local read "current sound"() -> (w1844:dbl)
                n1875 = local write "trial #"(w1814) -> ()
                n1876 = local read "time (s)"() -> (w1836:dbl)
                n1877 = local read "water # 1.2R"() -> (w1858:dbl)
                n1878 = local read "mistake # 2.2R"() -> (w1840:dbl)
                n1879 = local read "ITI (s)"() -> (w1843:dbl)
                n1880 = local read "mistake # 3.2R"() -> (w1825:dbl)
                n1881 = local read "mistake # 3.1L"() -> (w1826:dbl)
                n1882 = local read "time (s)"() -> (w1821:dbl)
                n1883 = local read "water # 1.1L"() -> (w1859:dbl)
                n1884 = local read "mistake # 1.2R"() -> (w1855:dbl)
                n1885 = local read "lick # 1.1L"() -> (w1861:dbl)
                n1886 = local read "mistake # 2.1L"() -> (w1841:dbl)
                n1887 = local read "lick # 1.2R"() -> (w1860:dbl)
                n1888 = local read "mistake # 1.1L"() -> (w1856:dbl)
                n1889 = local read "current sound"() -> (w1865:dbl)
                n1890 = local read "time (s)"() -> (w1851:dbl)
                n1891 = local read "ITI (s)"() -> (w1864:dbl)
                n1892 = local read "time (s)"() -> (w1867:dbl)
                n1893 = local read "Mouse path 1"() -> (w1869:path)
                n1894 = local read "Mouse path 2"() -> (w1852:path)
                n1895 = Build Array(w1821, w1820, w1819, w1818, w1817, 0.0 ("element"), 1.0 ("element"), w1814, w1813, w1812, 0.0 ("element"), w1810, w1809) -> (w1822:dbl[])
                n1896 = Build Array(w1836, w1835, w1834, w1833, w1832, 0.0 ("element"), 1 ("element"), w1814, w1829, w1828, 0.0 ("element"), w1826, w1825) -> (w1838:dbl[])
                n1897 = local read "Mouse path 4"() -> (w1823:path)
                n1898 = Build Array(w1851, w1850, w1849, w1848, w1847, 0.0 ("element"), 1 ("element"), w1814, w1844, w1843, 0 ("element"), w1841, w1840) -> (w1853:dbl[])
                n1899 = local read "Mouse path 3"() -> (w1837:path)
                n1900 = Build Array(w1867, w1861, w1860, w1859, w1858, 0.0 ("element"), 1, w1814, w1865, w1864, 0, w1856, w1855) -> (w1862:dbl[])
                n1901 = call-poly <vilib>:"Write To Spreadsheet File.vi"("append to file? (new file:F)"=TRUE, "1D data"=w1853, "file path (dialog if empty)"=w1852) -> ()  [unwired: 5 in, 1 out]
                n1902 = call-poly <vilib>:"Write To Spreadsheet File.vi"("append to file? (new file:F)"=TRUE, "1D data"=w1862, "file path (dialog if empty)"=w1869) -> ()  [unwired: 5 in, 1 out]
                n1903 = call-poly <vilib>:"Write To Spreadsheet File.vi"("append to file? (new file:F)"=TRUE, "1D data"=w1822, "file path (dialog if empty)"=w1823) -> ()  [unwired: 5 in, 1 out]
                n1904 = call-poly <vilib>:"Write To Spreadsheet File.vi"("append to file? (new file:F)"=TRUE, "1D data"=w1838, "file path (dialog if empty)"=w1837) -> ()  [unwired: 5 in, 1 out]
              }
              frame #2 {
                w1871 = enum16{"waiting", "sound", "ITI"}."sound"
                n1905 = local write "state 1.2"(w1871) -> ()
                n1906 = local write "state 1.1"(w1871) -> ()
                n1907 = local write "state 3.2"(w1871) -> ()
                n1908 = local write "state 3.1"(w1871) -> ()
                n1909 = local write "state 4.2"(w1871) -> ()
                n1910 = local write "state 2.1"(w1871) -> ()
                n1911 = local write "state 2.2"(w1871) -> ()
                n1912 = local write "state 4.1"(w1871) -> ()
              }
              frame #3 {
              }
            }
          }
          frame "sound" {
            n1913 = flat-sequence {
              tunnel: [T1."free water"] -> w1873
              frame #0 {
                n1914 = local read "current sound"() -> (w1879:dbl)
                n1915 = case shown="3" w1879 {
                  tunnel: "sound dur (ms)" -> [w1884 w1889 w1894 w1898]
                  tunnel: "sound port 1" -> [w1881 _ w1891 _]
                  tunnel: "sound port 2" -> [_ w1886 _ w1899]
                  tunnel: "sound file 1" -> [w1880 _ _ w1895]
                  tunnel: "sound file 2" -> [_ w1885 w1890 _]
                  frame ..1 {
                    n1916 = local read "Left Speaker"() -> (w1883:dbl)
                    n1917 = Increment(x=w1883) -> (x+1=w1882:dbl)
                    n1918 = local write "Left Speaker"(w1882) -> ()
                    n1919 = call "_play_wave_file.vi"("sound length (ms)"=w1884, "sound file"=w1880, "sound port"=w1881) -> ()  [unwired: 9 in]
                  }
                  frame 2 {
                    n1920 = local read "Right Speaker"() -> (w1888:dbl)
                    n1921 = Increment(x=w1888) -> (x+1=w1887:dbl)
                    n1922 = call "_play_wave_file.vi"("sound length (ms)"=w1889, "sound file"=w1885, "sound port"=w1886) -> ()  [unwired: 9 in]
                    n1923 = local write "Right Speaker"(w1887) -> ()
                  }
                  frame 3 {
                    n1924 = local read "Left Speaker"() -> (w1893:dbl)
                    n1925 = call "_play_wave_file.vi"("sound length (ms)"=w1894, "sound file"=w1890, "sound port"=w1891) -> ()  [unwired: 9 in]
                    n1926 = Increment(x=w1893) -> (x+1=w1892:dbl)
                    n1927 = local write "Left Speaker"(w1892) -> ()
                  }
                  frame 4.. {
                    n1928 = local read "Right Speaker"() -> (w1897:dbl)
                    n1929 = Increment(x=w1897) -> (x+1=w1896:dbl)
                    n1930 = call "_play_wave_file.vi"("sound length (ms)"=w1898, "sound file"=w1895, "sound port"=w1899) -> ()  [unwired: 9 in]
                    n1931 = local write "Right Speaker"(w1896) -> ()
                  }
                }
              }
              frame #1 {
                w1900 = enum16{"waiting", "sound", "ITI"}."waiting"
                n1932 = local write "state 1.1"(w1900) -> ()
                n1933 = local write "state 1.2"(w1900) -> ()
                n1934 = local write "state 2.1"(w1900) -> ()
                n1935 = local write "state 2.2"(w1900) -> ()
                n1936 = local write "state 3.2"(w1900) -> ()
                n1937 = local write "state 3.1"(w1900) -> ()
                n1938 = local write "state 4.1"(w1900) -> ()
                n1939 = local write "state 4.2"(w1900) -> ()
              }
              frame #2 {
              }
            }
          }
          frame "reaction window" {
            n1940 = flat-sequence {
              tunnel: [T1."graph"] -> w1902
              frame #0 {
                n1941 = Wait (ms)(milliseconds to wait="reaction dur (ms)") -> ()  [unwired: 1 out]
              }
              frame #1 {
                n1942 = local read "LED 2 (i)"() -> (w1906:dbl)
                n1943 = local read "LED 3 (i)"() -> (w1905:dbl)
                n1944 = local read "LED 1(i)"() -> (w1907:dbl)
                n1945 = local read "LED 4 (i)"() -> (w1904:dbl)
                n1946 = case shown="1" w1906 {
                  frame 0, Default {
                  }
                  frame 1 {
                    n1947 = local read "LED 2"() -> (w1913:tag)
                    n1948 = local write "LED 2 (i)"(0.0 ("LED 2 (i)")) -> ()
                    n1949 = call "_digital_on_LED.vi"("digital port"=w1913) -> ()  [unwired: 11 in]
                  }
                }
                n1950 = case shown="1" w1907 {
                  frame 0, Default {
                  }
                  frame 1 {
                    n1951 = local write "LED 1(i)"(0.0 ("LED 1(i)")) -> ()
                    n1952 = call "_digital_on_LED.vi"("digital port"="LED 1") -> ()  [unwired: 11 in]
                  }
                }
                n1953 = case shown="1" w1905 {
                  frame 0, Default {
                  }
                  frame 1 {
                    n1954 = local read "LED 3"() -> (w1911:tag)
                    n1955 = local write "LED 3 (i)"(0.0 ("LED 3 (i)")) -> ()
                    n1956 = call "_digital_on_LED.vi"("digital port"=w1911) -> ()  [unwired: 11 in]
                  }
                }
                n1957 = case shown="1" w1904 {
                  frame 0, Default {
                  }
                  frame 1 {
                    n1958 = local read "LED 4"() -> (w1909:tag)
                    n1959 = local write "LED 4 (i)"(0.0 ("LED 4 (i)")) -> ()
                    n1960 = call "_digital_on_LED.vi"("digital port"=w1909) -> ()  [unwired: 11 in]
                  }
                }
              }
              frame #2 {
              }
            }
          }
          frame "ITI" {
            n1961 = flat-sequence {
              tunnel: [T1."prepare"] -> w1917
              frame #0 {
                w1918 = enum16{"waiting", "sound", "ITI"}."ITI"
                n1962 = local write "state 1.1"(w1918) -> ()
                n1963 = local write "state 4.1"(w1918) -> ()
                n1964 = local write "state 1.2"(w1918) -> ()
                n1965 = local write "state 4.2"(w1918) -> ()
                n1966 = local write "state 2.2"(w1918) -> ()
                n1967 = local write "state 3.1"(w1918) -> ()
                n1968 = local write "state 2.1"(w1918) -> ()
                n1969 = local write "state 3.2"(w1918) -> ()
              }
              frame #1 {
                n1970 = local read "ITI (s)"() -> (w1921:dbl)
                n1971 = Multiply(x=w1921, y=1000) -> (x*y=w1919:dbl)
                n1972 = Wait (ms)(milliseconds to wait=w1919) -> ()  [unwired: 1 out]
              }
              frame #2 {
              }
            }
          }
          frame "free water" {
            n1973 = flat-sequence {
              tunnel: [T1."reaction window"] -> w1923
              frame #0 {
                n1974 = local read "state 4.2"() -> (w1927:enum16{"waiting", "sound", "ITI"})
                n1975 = local read "state 4.1"() -> (w1928:enum16{"waiting", "sound", "ITI"})
                n1976 = local read "state 1.1"() -> (w1952:enum16{"waiting", "sound", "ITI"})
                n1977 = local read "state 1.2"() -> (w1951:enum16{"waiting", "sound", "ITI"})
                n1978 = local read "state 2.1"() -> (w1939:enum16{"waiting", "sound", "ITI"})
                n1979 = local read "state 2.2"() -> (w1938:enum16{"waiting", "sound", "ITI"})
                n1980 = local read "state 3.1"() -> (w1935:enum16{"waiting", "sound", "ITI"})
                n1981 = local read "state 3.2"() -> (w1934:enum16{"waiting", "sound", "ITI"})
                n1982 = Build Array(w1952, w1951, w1939, w1938, w1935, w1934, w1928, w1927) -> (w1950:enum16{"waiting", "sound", "ITI"}[])
                n1983 = local write "free water 1.1"("free water 1.1") -> ()
                n1984 = local write "free water 1.2"("free water 1.2") -> ()
                n1985 = local write "free water 2.1"("free water 2.1") -> ()
                n1986 = local write "free water 3.1"("free water 3.1") -> ()
                n1987 = local write "free water 2.2"("free water 2.2") -> ()
                n1988 = local write "free water 3.2"("free water 3.2") -> ()
                n1989 = local write "free water 4.2"("free water 4.2") -> ()
                n1990 = local write "free water 4.1"("free water 4.1") -> ()
                n1991 = Build Array("free water 1.1", "free water 1.2", "free water 2.1", "free water 2.2", "free water 3.1", "free water 3.2", "free water 4.1", "free water 4.2") -> (w1954:bool[])
                n1992 = Equal?(x=w1950, y=enum16{"waiting", "water", "ITI"}."waiting") -> (x = y?=w1955:bool[])
                n1993 = And(x=w1955, y=w1954) -> (x .and. y?=w1953:bool[])
                n1994 = Index Array(array=w1953) -> (element #1=w1948:bool, element #2=w1945:bool, element #3=w1941:bool, element #4=w1940:bool, element #5=w1932:bool, element #6=w1931:bool, element #7=w1925:bool, element #8=w1924:bool)  [unwired: 8 in]
                n1995 = local read "current sound"() -> (w1949:dbl)
                n1996 = local read "current sound"() -> (w1942:dbl)
                n1997 = local read "current sound"() -> (w1926:dbl)
                n1998 = local read "current sound"() -> (w1933:dbl)
                n1999 = case shown="4" w1942 {
                  tunnel: w1941 -> [_ w2101 _ w2137 _]
                  tunnel: w1940 -> [_ _ w2119 _ w2155]
                  frame 0, Default {
                  }
                  frame 1 {
                    n2000 = case shown="True" w2101 {
                      frame False {
                      }
                      frame True {
                        w2108 = 0.0 ("element")
                        n2001 = local read "water # 2.1L"() -> (w2110:dbl)
                        n2002 = local read "water dur (ms) 2.1"() -> (w2117:dbl)
                        n2003 = local read "water # 2.2R"() -> (w2109:dbl)
                        n2004 = local read "water port 2.1"() -> (w2118:tag)
                        n2005 = local read "lick  #  2.2R"() -> (w2111:dbl)
                        n2006 = local read "lick  #  2.1L"() -> (w2112:dbl)
                        n2007 = local read "time (s)"() -> (w2113:dbl)
                        n2008 = local read "mistake # 2.2R"() -> (w2102:dbl)
                        n2009 = local read "current sound"() -> (w2106:dbl)
                        n2010 = local read "mistake # 2.1L"() -> (w2103:dbl)
                        n2011 = local read "ITI (s)"() -> (w2105:dbl)
                        n2012 = local read "trial #"() -> (w2107:dbl)
                        n2013 = local read "Mouse path 2"() -> (w2114:path)
                        n2014 = call "_digital_on_duration_off.vi"("duration (ms)"=w2117, "digital port"=w2118) -> ()  [unwired: 10 in]
                        n2015 = Build Array(w2113, w2112, w2111, w2110, w2109, w2108, w2108, w2107, w2106, w2105, 1.0 ("element"), w2103, w2102) -> (w2116:dbl[])
                        n2016 = call-poly <vilib>:"Write To Spreadsheet File.vi"("append to file? (new file:F)"=TRUE, "1D data"=w2116, "file path (dialog if empty)"=w2114) -> ()  [unwired: 5 in, 1 out]
                      }
                    }
                  }
                  frame 2 {
                    n2017 = case shown="True" w2119 {
                      frame False {
                      }
                      frame True {
                        w2126 = 0.0 ("element")
                        n2018 = local read "water # 2.2R"() -> (w2127:dbl)
                        n2019 = local read "water # 2.1L"() -> (w2128:dbl)
                        n2020 = local read "lick  #  2.2R"() -> (w2129:dbl)
                        n2021 = local read "lick  #  2.1L"() -> (w2130:dbl)
                        n2022 = local read "current sound"() -> (w2124:dbl)
                        n2023 = local read "ITI (s)"() -> (w2123:dbl)
                        n2024 = local read "trial #"() -> (w2125:dbl)
                        n2025 = local read "time (s)"() -> (w2131:dbl)
                        n2026 = local read "water dur (ms) 2.2"() -> (w2135:dbl)
                        n2027 = local read "mistake # 2.2R"() -> (w2120:dbl)
                        n2028 = local read "water port 2.2"() -> (w2136:tag)
                        n2029 = local read "mistake # 2.1L"() -> (w2121:dbl)
                        n2030 = local read "Mouse path 2"() -> (w2132:path)
                        n2031 = Build Array(w2131, w2130, w2129, w2128, w2127, w2126, w2126, w2125, w2124, w2123, 1.0 ("element"), w2121, w2120) -> (w2133:dbl[])
                        n2032 = call "_digital_on_duration_off.vi"("duration (ms)"=w2135, "digital port"=w2136) -> ()  [unwired: 10 in]
                        n2033 = call-poly <vilib>:"Write To Spreadsheet File.vi"("append to file? (new file:F)"=TRUE, "1D data"=w2133, "file path (dialog if empty)"=w2132) -> ()  [unwired: 5 in, 1 out]
                      }
                    }
                  }
                  frame 3 {
                    n2034 = case shown="True" w2137 {
                      frame False {
                      }
                      frame True {
                        w2144 = 0.0 ("element")
                        n2035 = local read "water # 2.2R"() -> (w2145:dbl)
                        n2036 = local read "water # 2.1L"() -> (w2146:dbl)
                        n2037 = local read "lick  #  2.1L"() -> (w2148:dbl)
                        n2038 = local read "lick  #  2.2R"() -> (w2147:dbl)
                        n2039 = local read "current sound"() -> (w2142:dbl)
                        n2040 = local read "time (s)"() -> (w2149:dbl)
                        n2041 = local read "ITI (s)"() -> (w2141:dbl)
                        n2042 = local read "trial #"() -> (w2143:dbl)
                        n2043 = local read "water dur (ms) 2.1"() -> (w2153:dbl)
                        n2044 = local read "mistake # 2.2R"() -> (w2138:dbl)
                        n2045 = local read "mistake # 2.1L"() -> (w2139:dbl)
                        n2046 = local read "water port 2.1"() -> (w2154:tag)
                        n2047 = local read "Mouse path 2"() -> (w2150:path)
                        n2048 = call "_digital_on_duration_off.vi"("duration (ms)"=w2153, "digital port"=w2154) -> ()  [unwired: 10 in]
                        n2049 = Build Array(w2149, w2148, w2147, w2146, w2145, w2144, w2144, w2143, w2142, w2141, 1.0 ("element"), w2139, w2138) -> (w2151:dbl[])
                        n2050 = call-poly <vilib>:"Write To Spreadsheet File.vi"("append to file? (new file:F)"=TRUE, "1D data"=w2151, "file path (dialog if empty)"=w2150) -> ()  [unwired: 5 in, 1 out]
                      }
                    }
                  }
                  frame 4 {
                    n2051 = case shown="True" w2155 {
                      frame False {
                      }
                      frame True {
                        w2162 = 0.0 ("element")
                        n2052 = local read "water # 2.2R"() -> (w2163:dbl)
                        n2053 = local read "water # 2.1L"() -> (w2164:dbl)
                        n2054 = local read "lick  #  2.2R"() -> (w2165:dbl)
                        n2055 = local read "current sound"() -> (w2160:dbl)
                        n2056 = local read "lick  #  2.1L"() -> (w2166:dbl)
                        n2057 = local read "ITI (s)"() -> (w2159:dbl)
                        n2058 = local read "trial #"() -> (w2161:dbl)
                        n2059 = local read "mistake # 2.2R"() -> (w2156:dbl)
                        n2060 = local read "mistake # 2.1L"() -> (w2157:dbl)
                        n2061 = local read "time (s)"() -> (w2167:dbl)
                        n2062 = local read "water dur (ms) 2.2"() -> (w2171:dbl)
                        n2063 = local read "water port 2.2"() -> (w2172:tag)
                        n2064 = local read "Mouse path 2"() -> (w2169:path)
                        n2065 = Build Array(w2167, w2166, w2165, w2164, w2163, w2162, w2162, w2161, w2160, w2159, 1.0 ("element"), w2157, w2156) -> (w2168:dbl[])
                        n2066 = call "_digital_on_duration_off.vi"("duration (ms)"=w2171, "digital port"=w2172) -> ()  [unwired: 10 in]
                        n2067 = call-poly <vilib>:"Write To Spreadsheet File.vi"("append to file? (new file:F)"=TRUE, "1D data"=w2168, "file path (dialog if empty)"=w2169) -> ()  [unwired: 5 in, 1 out]
                      }
                    }
                  }
                }
                n2068 = case shown="4" w1949 {
                  tunnel: w1948 -> [_ w2173 _ w2209 _]
                  tunnel: w1945 -> [_ _ w2191 _ w2227]
                  frame 0, Default {
                  }
                  frame 1 {
                    n2069 = case shown="True" w2173 {
                      frame False {
                      }
                      frame True {
                        w2180 = 0
                        n2070 = local read "water # 1.1L"() -> (w2177:dbl)
                        n2071 = local read "water # 1.2R"() -> (w2176:dbl)
                        n2072 = local read "water port 1.1"() -> (w2182:tag)
                        n2073 = local read "water dur (ms) 1.1"() -> (w2181:dbl)
                        n2074 = local read "lick # 1.2R"() -> (w2178:dbl)
                        n2075 = local read "lick # 1.1L"() -> (w2179:dbl)
                        n2076 = local read "current sound"() -> (w2186:dbl)
                        n2077 = local read "mistake # 1.2R"() -> (w2174:dbl)
                        n2078 = local read "trial #"() -> (w2187:dbl)
                        n2079 = local read "time (s)"() -> (w2188:dbl)
                        n2080 = local read "mistake # 1.1L"() -> (w2175:dbl)
                        n2081 = local read "ITI (s)"() -> (w2185:dbl)
                        n2082 = call "_digital_on_duration_off.vi"("duration (ms)"=w2181, "digital port"=w2182) -> ()  [unwired: 10 in]
                        n2083 = local read "Mouse path 1"() -> (w2189:path)
                        n2084 = Build Array(w2188, w2179, w2178, w2177, w2176, w2180, w2180, w2187, w2186, w2185, 1, w2175, w2174) -> (w2183:dbl[])
                        n2085 = call-poly <vilib>:"Write To Spreadsheet File.vi"("append to file? (new file:F)"=TRUE, "1D data"=w2183, "file path (dialog if empty)"=w2189) -> ()  [unwired: 5 in, 1 out]
                      }
                    }
                  }
                  frame 2 {
                    n2086 = case shown="True" w2191 {
                      frame False {
                      }
                      frame True {
                        w2200 = 0 ("element")
                        n2087 = local read "water # 1.1L"() -> (w2195:dbl)
                        n2088 = local read "lick # 1.2R"() -> (w2196:dbl)
                        n2089 = local read "water # 1.2R"() -> (w2194:dbl)
                        n2090 = local read "mistake # 1.2R"() -> (w2192:dbl)
                        n2091 = local read "lick # 1.1L"() -> (w2197:dbl)
                        n2092 = local read "current sound"() -> (w2203:dbl)
                        n2093 = local read "mistake # 1.1L"() -> (w2193:dbl)
                        n2094 = local read "trial #"() -> (w2204:dbl)
                        n2095 = local read "ITI (s)"() -> (w2202:dbl)
                        n2096 = local read "time (s)"() -> (w2205:dbl)
                        n2097 = local read "water dur (ms) 1.2"() -> (w2198:dbl)
                        n2098 = Build Array(w2205, w2197, w2196, w2195, w2194, w2200, w2200, w2204, w2203, w2202, 1 ("element"), w2193, w2192) -> (w2206:dbl[])
                        n2099 = local read "Mouse path 1"() -> (w2207:path)
                        n2100 = local read "water port 1.2"() -> (w2199:tag)
                        n2101 = call-poly <vilib>:"Write To Spreadsheet File.vi"("append to file? (new file:F)"=TRUE, "1D data"=w2206, "file path (dialog if empty)"=w2207) -> ()  [unwired: 5 in, 1 out]
                        n2102 = call "_digital_on_duration_off.vi"("duration (ms)"=w2198, "digital port"=w2199) -> ()  [unwired: 10 in]
                      }
                    }
                  }
                  frame 3 {
                    n2103 = case shown="True" w2209 {
                      frame False {
                      }
                      frame True {
                        w2216 = 0.0 ("element")
                        n2104 = local read "lick # 1.2R"() -> (w2219:dbl)
                        n2105 = local read "water # 1.2R"() -> (w2217:dbl)
                        n2106 = local read "water # 1.1L"() -> (w2218:dbl)
                        n2107 = local read "lick # 1.1L"() -> (w2220:dbl)
                        n2108 = local read "time (s)"() -> (w2221:dbl)
                        n2109 = local read "current sound"() -> (w2214:dbl)
                        n2110 = local read "mistake # 1.1L"() -> (w2211:dbl)
                        n2111 = local read "mistake # 1.2R"() -> (w2210:dbl)
                        n2112 = local read "trial #"() -> (w2215:dbl)
                        n2113 = local read "ITI (s)"() -> (w2213:dbl)
                        n2114 = local read "water dur (ms) 1.1"() -> (w2225:dbl)
                        n2115 = local read "water port 1.1"() -> (w2226:tag)
                        n2116 = local read "Mouse path 1"() -> (w2222:path)
                        n2117 = Build Array(w2221, w2220, w2219, w2218, w2217, w2216, w2216, w2215, w2214, w2213, 1.0 ("element"), w2211, w2210) -> (w2223:dbl[])
                        n2118 = call "_digital_on_duration_off.vi"("duration (ms)"=w2225, "digital port"=w2226) -> ()  [unwired: 10 in]
                        n2119 = call-poly <vilib>:"Write To Spreadsheet File.vi"("append to file? (new file:F)"=TRUE, "1D data"=w2223, "file path (dialog if empty)"=w2222) -> ()  [unwired: 5 in, 1 out]
                      }
                    }
                  }
                  frame 4 {
                    n2120 = case shown="True" w2227 {
                      frame False {
                      }
                      frame True {
                        w2234 = 0.0 ("element")
                        n2121 = local read "water # 1.1L"() -> (w2236:dbl)
                        n2122 = local read "water # 1.2R"() -> (w2235:dbl)
                        n2123 = local read "lick # 1.2R"() -> (w2237:dbl)
                        n2124 = local read "lick # 1.1L"() -> (w2238:dbl)
                        n2125 = local read "water dur (ms) 1.2"() -> (w2243:dbl)
                        n2126 = local read "current sound"() -> (w2232:dbl)
                        n2127 = local read "time (s)"() -> (w2239:dbl)
                        n2128 = local read "water port 1.2"() -> (w2244:tag)
                        n2129 = local read "trial #"() -> (w2233:dbl)
                        n2130 = local read "ITI (s)"() -> (w2231:dbl)
                        n2131 = local read "mistake # 1.2R"() -> (w2228:dbl)
                        n2132 = local read "mistake # 1.1L"() -> (w2229:dbl)
                        n2133 = local read "Mouse path 1"() -> (w2240:path)
                        n2134 = call "_digital_on_duration_off.vi"("duration (ms)"=w2243, "digital port"=w2244) -> ()  [unwired: 10 in]
                        n2135 = Build Array(w2239, w2238, w2237, w2236, w2235, w2234, w2234, w2233, w2232, w2231, 1.0 ("element"), w2229, w2228) -> (w2241:dbl[])
                        n2136 = call-poly <vilib>:"Write To Spreadsheet File.vi"("append to file? (new file:F)"=TRUE, "1D data"=w2241, "file path (dialog if empty)"=w2240) -> ()  [unwired: 5 in, 1 out]
                      }
                    }
                  }
                }
                n2137 = case shown="4" w1933 {
                  tunnel: w1932 -> [_ w2029 _ w2065 _]
                  tunnel: w1931 -> [_ _ w2047 _ w2083]
                  frame 0, Default {
                  }
                  frame 1 {
                    n2138 = case shown="True" w2029 {
                      frame False {
                      }
                      frame True {
                        w2036 = 0.0 ("element")
                        n2139 = local read "water # 3.2R"() -> (w2037:dbl)
                        n2140 = local read "water # 3.1L"() -> (w2038:dbl)
                        n2141 = local read "current sound"() -> (w2034:dbl)
                        n2142 = local read "lick # 3.2R"() -> (w2039:dbl)
                        n2143 = local read "lick # 3.1L"() -> (w2040:dbl)
                        n2144 = local read "mistake # 3.2R"() -> (w2030:dbl)
                        n2145 = local read "trial #"() -> (w2035:dbl)
                        n2146 = local read "mistake # 3.1L"() -> (w2031:dbl)
                        n2147 = local read "ITI (s)"() -> (w2033:dbl)
                        n2148 = local read "time (s)"() -> (w2041:dbl)
                        n2149 = local read "water dur (ms) 3.1"() -> (w2045:dbl)
                        n2150 = local read "water port 3.1"() -> (w2046:tag)
                        n2151 = local read "Mouse path 3"() -> (w2043:path)
                        n2152 = Build Array(w2041, w2040, w2039, w2038, w2037, w2036, w2036, w2035, w2034, w2033, 1.0 ("element"), w2031, w2030) -> (w2042:dbl[])
                        n2153 = call "_digital_on_duration_off.vi"("duration (ms)"=w2045, "digital port"=w2046) -> ()  [unwired: 10 in]
                        n2154 = call-poly <vilib>:"Write To Spreadsheet File.vi"("append to file? (new file:F)"=TRUE, "1D data"=w2042, "file path (dialog if empty)"=w2043) -> ()  [unwired: 5 in, 1 out]
                      }
                    }
                  }
                  frame 2 {
                    n2155 = case shown="True" w2047 {
                      frame False {
                      }
                      frame True {
                        w2054 = 0.0 ("element")
                        n2156 = local read "water # 3.2R"() -> (w2055:dbl)
                        n2157 = local read "water # 3.1L"() -> (w2056:dbl)
                        n2158 = local read "current sound"() -> (w2052:dbl)
                        n2159 = local read "mistake # 3.2R"() -> (w2048:dbl)
                        n2160 = local read "lick # 3.2R"() -> (w2057:dbl)
                        n2161 = local read "mistake # 3.1L"() -> (w2049:dbl)
                        n2162 = local read "lick # 3.1L"() -> (w2058:dbl)
                        n2163 = local read "trial #"() -> (w2053:dbl)
                        n2164 = local read "ITI (s)"() -> (w2051:dbl)
                        n2165 = local read "time (s)"() -> (w2059:dbl)
                        n2166 = local read "water dur (ms) 3. 2"() -> (w2063:dbl)
                        n2167 = local read "Mouse path 3"() -> (w2061:path)
                        n2168 = local read "water port 3.2"() -> (w2064:tag)
                        n2169 = Build Array(w2059, w2058, w2057, w2056, w2055, w2054, w2054, w2053, w2052, w2051, 1.0 ("element"), w2049, w2048) -> (w2060:dbl[])
                        n2170 = call-poly <vilib>:"Write To Spreadsheet File.vi"("append to file? (new file:F)"=TRUE, "1D data"=w2060, "file path (dialog if empty)"=w2061) -> ()  [unwired: 5 in, 1 out]
                        n2171 = call "_digital_on_duration_off.vi"("duration (ms)"=w2063, "digital port"=w2064) -> ()  [unwired: 10 in]
                      }
                    }
                  }
                  frame 3 {
                    n2172 = case shown="True" w2065 {
                      frame False {
                      }
                      frame True {
                        w2072 = 0.0 ("element")
                        n2173 = local read "water # 3.1L"() -> (w2074:dbl)
                        n2174 = local read "water # 3.2R"() -> (w2073:dbl)
                        n2175 = local read "lick # 3.1L"() -> (w2076:dbl)
                        n2176 = local read "lick # 3.2R"() -> (w2075:dbl)
                        n2177 = local read "current sound"() -> (w2070:dbl)
                        n2178 = local read "ITI (s)"() -> (w2069:dbl)
                        n2179 = local read "trial #"() -> (w2071:dbl)
                        n2180 = local read "mistake # 3.2R"() -> (w2066:dbl)
                        n2181 = local read "time (s)"() -> (w2077:dbl)
                        n2182 = local read "mistake # 3.1L"() -> (w2067:dbl)
                        n2183 = local read "water dur (ms) 3.1"() -> (w2081:dbl)
                        n2184 = local read "water port 3.1"() -> (w2082:tag)
                        n2185 = local read "Mouse path 3"() -> (w2079:path)
                        n2186 = Build Array(w2077, w2076, w2075, w2074, w2073, w2072, w2072, w2071, w2070, w2069, 1.0 ("element"), w2067, w2066) -> (w2078:dbl[])
                        n2187 = call "_digital_on_duration_off.vi"("duration (ms)"=w2081, "digital port"=w2082) -> ()  [unwired: 10 in]
                        n2188 = call-poly <vilib>:"Write To Spreadsheet File.vi"("append to file? (new file:F)"=TRUE, "1D data"=w2078, "file path (dialog if empty)"=w2079) -> ()  [unwired: 5 in, 1 out]
                      }
                    }
                  }
                  frame 4 {
                    n2189 = case shown="True" w2083 {
                      frame False {
                      }
                      frame True {
                        w2090 = 0.0 ("element")
                        n2190 = local read "water # 3.1L"() -> (w2092:dbl)
                        n2191 = local read "water # 3.2R"() -> (w2091:dbl)
                        n2192 = local read "current sound"() -> (w2088:dbl)
                        n2193 = local read "lick # 3.2R"() -> (w2093:dbl)
                        n2194 = local read "lick # 3.1L"() -> (w2094:dbl)
                        n2195 = local read "trial #"() -> (w2089:dbl)
                        n2196 = local read "ITI (s)"() -> (w2087:dbl)
                        n2197 = local read "time (s)"() -> (w2095:dbl)
                        n2198 = local read "mistake # 3.1L"() -> (w2085:dbl)
                        n2199 = local read "mistake # 3.2R"() -> (w2084:dbl)
                        n2200 = local read "water dur (ms) 3. 2"() -> (w2099:dbl)
                        n2201 = local read "water port 3.2"() -> (w2100:tag)
                        n2202 = local read "Mouse path 3"() -> (w2097:path)
                        n2203 = Build Array(w2095, w2094, w2093, w2092, w2091, w2090, w2090, w2089, w2088, w2087, 1.0 ("element"), w2085, w2084) -> (w2096:dbl[])
                        n2204 = call "_digital_on_duration_off.vi"("duration (ms)"=w2099, "digital port"=w2100) -> ()  [unwired: 10 in]
                        n2205 = call-poly <vilib>:"Write To Spreadsheet File.vi"("append to file? (new file:F)"=TRUE, "1D data"=w2096, "file path (dialog if empty)"=w2097) -> ()  [unwired: 5 in, 1 out]
                      }
                    }
                  }
                }
                n2206 = case shown="4" w1926 {
                  tunnel: w1925 -> [_ w1957 _ w1993 _]
                  tunnel: w1924 -> [_ _ w1975 _ w2011]
                  frame 0, Default {
                  }
                  frame 1 {
                    n2207 = case shown="True" w1957 {
                      frame False {
                      }
                      frame True {
                        w1964 = 0.0 ("element")
                        n2208 = local read "water # 4.1L"() -> (w1966:dbl)
                        n2209 = local read "water # 4.2R"() -> (w1965:dbl)
                        n2210 = local read "lick # 4.2R"() -> (w1967:dbl)
                        n2211 = local read "lick # 4.1L"() -> (w1968:dbl)
                        n2212 = local read "current sound"() -> (w1962:dbl)
                        n2213 = local read "mistake # 4.2R"() -> (w1958:dbl)
                        n2214 = local read "mistake # 4.1L"() -> (w1959:dbl)
                        n2215 = local read "ITI (s)"() -> (w1961:dbl)
                        n2216 = local read "trial #"() -> (w1963:dbl)
                        n2217 = local read "time (s)"() -> (w1969:dbl)
                        n2218 = local read "water dur (ms) 4.1"() -> (w1973:dbl)
                        n2219 = local read "water port 4.1"() -> (w1974:tag)
                        n2220 = local read "Mouse path 4"() -> (w1970:path)
                        n2221 = Build Array(w1969, w1968, w1967, w1966, w1965, w1964, w1964, w1963, w1962, w1961, 1.0 ("element"), w1959, w1958) -> (w1971:dbl[])
                        n2222 = call "_digital_on_duration_off.vi"("duration (ms)"=w1973, "digital port"=w1974) -> ()  [unwired: 10 in]
                        n2223 = call-poly <vilib>:"Write To Spreadsheet File.vi"("append to file? (new file:F)"=TRUE, "1D data"=w1971, "file path (dialog if empty)"=w1970) -> ()  [unwired: 5 in, 1 out]
                      }
                    }
                  }
                  frame 2 {
                    n2224 = case shown="True" w1975 {
                      frame False {
                      }
                      frame True {
                        w1982 = 0.0 ("element")
                        n2225 = local read "lick # 4.2R"() -> (w1985:dbl)
                        n2226 = local read "current sound"() -> (w1980:dbl)
                        n2227 = local read "water # 4.2R"() -> (w1983:dbl)
                        n2228 = local read "water # 4.1L"() -> (w1984:dbl)
                        n2229 = local read "lick # 4.1L"() -> (w1986:dbl)
                        n2230 = local read "trial #"() -> (w1981:dbl)
                        n2231 = local read "time (s)"() -> (w1987:dbl)
                        n2232 = local read "ITI (s)"() -> (w1979:dbl)
                        n2233 = local read "mistake # 4.1L"() -> (w1977:dbl)
                        n2234 = local read "mistake # 4.2R"() -> (w1976:dbl)
                        n2235 = local read "water dur (ms) 4.2"() -> (w1991:dbl)
                        n2236 = local read "water port 4.2"() -> (w1992:tag)
                        n2237 = local read "Mouse path 4"() -> (w1988:path)
                        n2238 = Build Array(w1987, w1986, w1985, w1984, w1983, w1982, w1982, w1981, w1980, w1979, 1.0 ("element"), w1977, w1976) -> (w1989:dbl[])
                        n2239 = call "_digital_on_duration_off.vi"("duration (ms)"=w1991, "digital port"=w1992) -> ()  [unwired: 10 in]
                        n2240 = call-poly <vilib>:"Write To Spreadsheet File.vi"("append to file? (new file:F)"=TRUE, "1D data"=w1989, "file path (dialog if empty)"=w1988) -> ()  [unwired: 5 in, 1 out]
                      }
                    }
                  }
                  frame 3 {
                    n2241 = case shown="True" w1993 {
                      frame False {
                      }
                      frame True {
                        w2000 = 0.0 ("element")
                        n2242 = local read "water # 4.2R"() -> (w2001:dbl)
                        n2243 = local read "current sound"() -> (w1998:dbl)
                        n2244 = local read "water # 4.1L"() -> (w2002:dbl)
                        n2245 = local read "lick # 4.2R"() -> (w2003:dbl)
                        n2246 = local read "ITI (s)"() -> (w1997:dbl)
                        n2247 = local read "lick # 4.1L"() -> (w2004:dbl)
                        n2248 = local read "trial #"() -> (w1999:dbl)
                        n2249 = local read "mistake # 4.2R"() -> (w1994:dbl)
                        n2250 = local read "mistake # 4.1L"() -> (w1995:dbl)
                        n2251 = local read "time (s)"() -> (w2005:dbl)
                        n2252 = local read "water dur (ms) 4.1"() -> (w2009:dbl)
                        n2253 = local read "water port 4.1"() -> (w2010:tag)
                        n2254 = local read "Mouse path 4"() -> (w2007:path)
                        n2255 = Build Array(w2005, w2004, w2003, w2002, w2001, w2000, w2000, w1999, w1998, w1997, 1.0 ("element"), w1995, w1994) -> (w2006:dbl[])
                        n2256 = call-poly <vilib>:"Write To Spreadsheet File.vi"("append to file? (new file:F)"=TRUE, "1D data"=w2006, "file path (dialog if empty)"=w2007) -> ()  [unwired: 5 in, 1 out]
                        n2257 = call "_digital_on_duration_off.vi"("duration (ms)"=w2009, "digital port"=w2010) -> ()  [unwired: 10 in]
                      }
                    }
                  }
                  frame 4 {
                    n2258 = case shown="True" w2011 {
                      frame False {
                      }
                      frame True {
                        w2018 = 0.0 ("element")
                        n2259 = local read "water # 4.2R"() -> (w2019:dbl)
                        n2260 = local read "water # 4.1L"() -> (w2020:dbl)
                        n2261 = local read "current sound"() -> (w2016:dbl)
                        n2262 = local read "lick # 4.2R"() -> (w2021:dbl)
                        n2263 = local read "lick # 4.1L"() -> (w2022:dbl)
                        n2264 = local read "ITI (s)"() -> (w2015:dbl)
                        n2265 = local read "trial #"() -> (w2017:dbl)
                        n2266 = local read "time (s)"() -> (w2023:dbl)
                        n2267 = local read "mistake # 4.2R"() -> (w2012:dbl)
                        n2268 = local read "mistake # 4.1L"() -> (w2013:dbl)
                        n2269 = local read "water dur (ms) 4.2"() -> (w2027:dbl)
                        n2270 = local read "water port 4.2"() -> (w2028:tag)
                        n2271 = local read "Mouse path 4"() -> (w2025:path)
                        n2272 = Build Array(w2023, w2022, w2021, w2020, w2019, w2018, w2018, w2017, w2016, w2015, 1.0 ("element"), w2013, w2012) -> (w2024:dbl[])
                        n2273 = call-poly <vilib>:"Write To Spreadsheet File.vi"("append to file? (new file:F)"=TRUE, "1D data"=w2024, "file path (dialog if empty)"=w2025) -> ()  [unwired: 5 in, 1 out]
                        n2274 = call "_digital_on_duration_off.vi"("duration (ms)"=w2027, "digital port"=w2028) -> ()  [unwired: 10 in]
                      }
                    }
                  }
                }
              }
              frame #1 {
              }
            }
          }
          frame "graph" {
            n2275 = local read "mistake # 2.2R"() -> (w2280:dbl)
            n2276 = local read "mistake # 3.1L"() -> (w2272:dbl)
            n2277 = local read "mistake # 4.2R"() -> (w2248:dbl)
            n2278 = local read "mistake # 4.1L"() -> (w2256:dbl)
            n2279 = local read "water # 4.2R"() -> (w2249:dbl)
            n2280 = local read "water # 2.2R"() -> (w2281:dbl)
            n2281 = local read "water # 4.2R"() -> (w2250:dbl)
            n2282 = local read "mistake # 2.1L"() -> (w2288:dbl)
            n2283 = local read "water # 3.1L"() -> (w2273:dbl)
            n2284 = local read "water # 2.2R"() -> (w2282:dbl)
            n2285 = local read "water # 4.1L"() -> (w2257:dbl)
            n2286 = local read "water # 2.1L"() -> (w2289:dbl)
            n2287 = local read "water # 3.1L"() -> (w2275:dbl)
            n2288 = local read "mistake # 3.2R"() -> (w2264:dbl)
            n2289 = local read "mistake # 1.2R"() -> (w2297:dbl)
            n2290 = local read "water # 3.2R"() -> (w2265:dbl)
            n2291 = local read "water # 2.1L"() -> (w2290:dbl)
            n2292 = local read "water # 4.1L"() -> (w2259:dbl)
            n2293 = local read "mistake # 1.1L"() -> (w2304:dbl)
            n2294 = local read "water # 3.2R"() -> (w2267:dbl)
            n2295 = local read "water # 1.1L"() -> (w2305:dbl)
            n2296 = local read "water # 1.2R"() -> (w2298:dbl)
            n2297 = local read "water # 1.2R"() -> (w2299:dbl)
            n2298 = local read "water # 1.1L"() -> (w2307:dbl)
            n2299 = Add(x=w2249, y=w2248) -> (x+y=w2247:dbl)
            n2300 = Add(x=w2281, y=w2280) -> (x+y=w2279:dbl)
            n2301 = Add(x=w2289, y=w2288) -> (x+y=w2287:dbl)
            n2302 = Add(x=w2273, y=w2272) -> (x+y=w2271:dbl)
            n2303 = Add(x=w2305, y=w2304) -> (x+y=w2303:dbl)
            n2304 = Add(x=w2265, y=w2264) -> (x+y=w2263:dbl)
            n2305 = Add(x=w2298, y=w2297) -> (x+y=w2296:dbl)
            n2306 = Add(x=w2257, y=w2256) -> (x+y=w2255:dbl)
            n2307 = Divide(x=w2290, y=w2287) -> (x/y=w2291:dbl)
            n2308 = Divide(x=w2267, y=w2263) -> (x/y=w2266:dbl)
            n2309 = Divide(x=w2275, y=w2271) -> (x/y=w2274:dbl)
            n2310 = Divide(x=w2282, y=w2279) -> (x/y=w2283:dbl)
            n2311 = Divide(x=w2299, y=w2296) -> (x/y=w2295:dbl)
            n2312 = Divide(x=w2307, y=w2303) -> (x/y=w2306:dbl)
            n2313 = Divide(x=w2250, y=w2247) -> (x/y=w2251:dbl)
            n2314 = Divide(x=w2259, y=w2255) -> (x/y=w2258:dbl)
            n2315 = local read "time (s)"() -> (w2311:dbl)
            n2316 = call <vilib>:"Mean PtByPt.vi"("x"=w2274) -> ("mean"=w2276:dbl)  [unwired: 3 in, 1 out]
            n2317 = call <vilib>:"Mean PtByPt.vi"("x"=w2266) -> ("mean"=w2268:dbl)  [unwired: 3 in, 1 out]
            n2318 = call <vilib>:"Mean PtByPt.vi"("x"=w2295) -> ("mean"=w2300:dbl)  [unwired: 3 in, 1 out]
            n2319 = call <vilib>:"Mean PtByPt.vi"("x"=w2258) -> ("mean"=w2260:dbl)  [unwired: 3 in, 1 out]
            n2320 = call <vilib>:"Mean PtByPt.vi"("x"=w2251) -> ("mean"=w2246:dbl)  [unwired: 3 in, 1 out]
            n2321 = call <vilib>:"Mean PtByPt.vi"("x"=w2291) -> ("mean"=w2292:dbl)  [unwired: 3 in, 1 out]
            n2322 = call <vilib>:"Mean PtByPt.vi"("x"=w2283) -> ("mean"=w2284:dbl)  [unwired: 3 in, 1 out]
            n2323 = call <vilib>:"Mean PtByPt.vi"("x"=w2306) -> ("mean"=w2308:dbl)  [unwired: 3 in, 1 out]
            n2324 = local write "ratio 1.2R"(w2300) -> ()
            n2325 = local write "ratio 1.1L"(w2308) -> ()
            n2326 = local write "ratio 2.1L"(w2292) -> ()
            n2327 = local write "ratio 3.1L"(w2276) -> ()
            n2328 = local write "ratio 2.2R"(w2284) -> ()
            n2329 = local write "ratio 3.2R"(w2268) -> ()
            n2330 = call "ratio"("Signals"=w2311) -> ("Collected Signals"=w2252:dynamicdata)  [unwired: 9 in, 1 out]
            n2331 = call "ratio1"("Signals"=w2308) -> ("Collected Signals"=w2310:dynamicdata)  [unwired: 9 in, 1 out]
            n2332 = local write "ratio 4.2R"(w2246) -> ()
            n2333 = call "ratio2"("Signals"=w2300) -> ("Collected Signals"=w2302:dynamicdata)  [unwired: 9 in, 1 out]
            n2334 = local write "ratio 4.1L"(w2260) -> ()
            n2335 = call "ratio3"("Signals"=w2292) -> ("Collected Signals"=w2294:dynamicdata)  [unwired: 9 in, 1 out]
            n2336 = call "ratio5"("Signals"=w2276) -> ("Collected Signals"=w2278:dynamicdata)  [unwired: 9 in, 1 out]
            n2337 = call "ratio4"("Signals"=w2284) -> ("Collected Signals"=w2286:dynamicdata)  [unwired: 9 in, 1 out]
            n2338 = call "ratio6"("Signals"=w2268) -> ("Collected Signals"=w2270:dynamicdata)  [unwired: 9 in, 1 out]
            n2339 = call "ratio7"("Signals"=w2260) -> ("Collected Signals"=w2262:dynamicdata)  [unwired: 9 in, 1 out]
            n2340 = call "ratio8"("Signals"=w2246) -> ("Collected Signals"=w2254:dynamicdata)  [unwired: 9 in, 1 out]
            n2341 = call "Build ratio1"("Y Input"=w2310, "X Input"=w2252) -> ("XY Graph"=→"ratio 1.1L":cluster{"Y":dbl[], "Y":dbl[]}[])  [unwired: 3 in, 6 out]
            n2342 = call "Build ratio"("Y Input"=w2302, "X Input"=w2252) -> ("XY Graph"=→"ratio 1.2R":cluster{"Y":dbl[], "Y":dbl[]}[])  [unwired: 3 in, 6 out]
            n2343 = call "Build ratio2"("Y Input"=w2294, "X Input"=w2252) -> ("XY Graph"=→"ratio 2.1L":cluster{"Y":dbl[], "Y":dbl[]}[])  [unwired: 3 in, 6 out]
            n2344 = call "Build ratio4"("Y Input"=w2278, "X Input"=w2252) -> ("XY Graph"=→"ratio 3.1L":cluster{"Y":dbl[], "Y":dbl[]}[])  [unwired: 3 in, 6 out]
            n2345 = call "Build ratio3"("Y Input"=w2286, "X Input"=w2252) -> ("XY Graph"=→"ratio 2.2R":cluster{"Y":dbl[], "Y":dbl[]}[])  [unwired: 3 in, 6 out]
            n2346 = call "Build ratio5"("Y Input"=w2270, "X Input"=w2252) -> ("XY Graph"=→"ratio 3.2R":cluster{"Y":dbl[], "Y":dbl[]}[])  [unwired: 3 in, 6 out]
            n2347 = call "Build ratio6"("Y Input"=w2262, "X Input"=w2252) -> ("XY Graph"=→"ratio 4.1L":cluster{"Y":dbl[], "Y":dbl[]}[])  [unwired: 3 in, 6 out]
            n2348 = call "Build ratio7"("Y Input"=w2254, "X Input"=w2252) -> ("XY Graph"=→"ratio 4.2R":cluster{"Y":dbl[], "Y":dbl[]}[])  [unwired: 3 in, 6 out]
          }
          frame "data collection" {
          }
        }
        n2349 = Wait (ms)(milliseconds to wait=u32 0) -> ()  [unwired: 1 out]
      }
    }
  }
